vi "DrawOneLineXY.vi"() -> ()   [LabVIEW 2019]
uses:
  <vilib>/Utility/miscctls.llb/LVBoundsTypeDef.ctl
panel:
  out "Plot Area:Size":T1
  in  "stop":bool
  out "XY Graph":cluster{"X":dbl, "Y":dbl}[](graph)
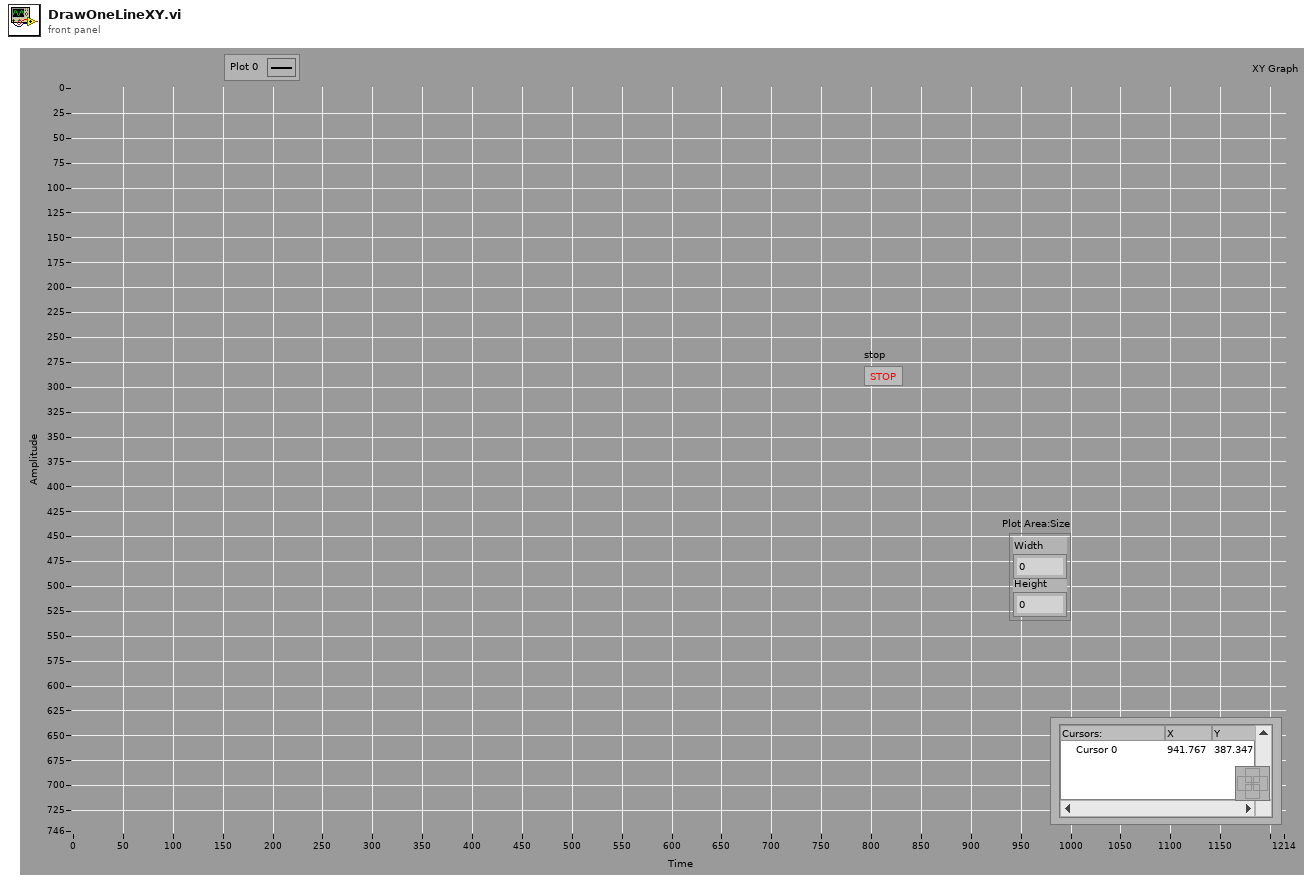
[diagram p1: front panel]
types:
  T1 = typedef "LVBoundsTypeDef.ctl" = cluster{"Width":u32, "Height":u32}
  T2 = typedef "LVPoint32TypeDef.ctl" = cluster{"Horizontal":i32, "Vertical":i32}
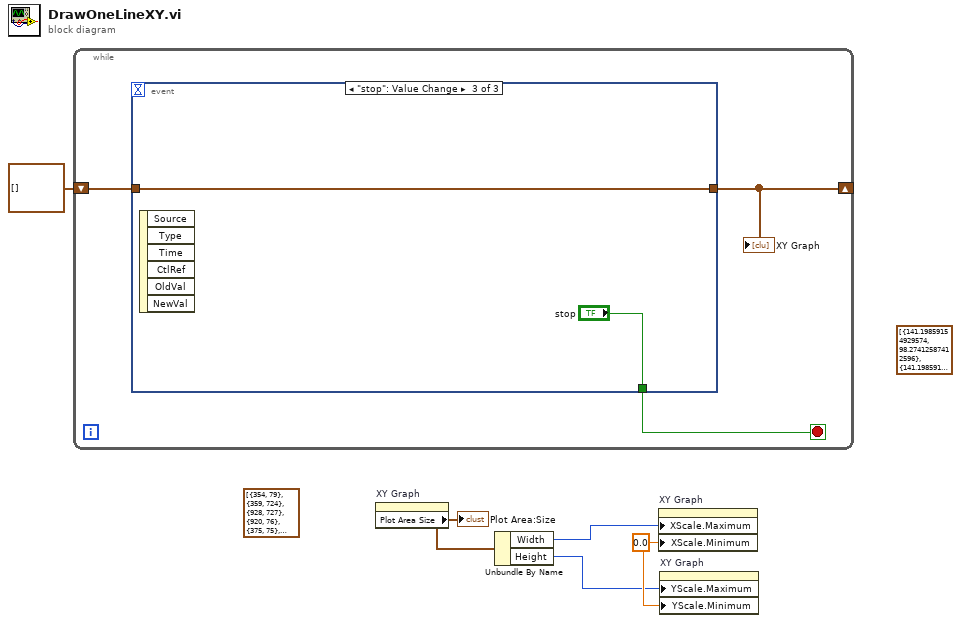
[diagram p0: block diagram]
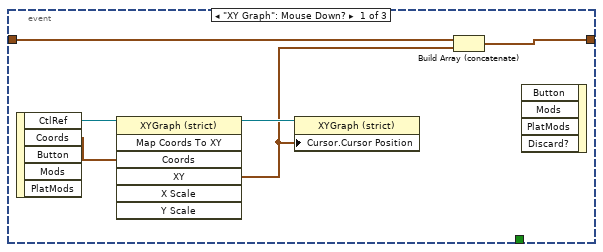
[diagram p2: hidden frame]
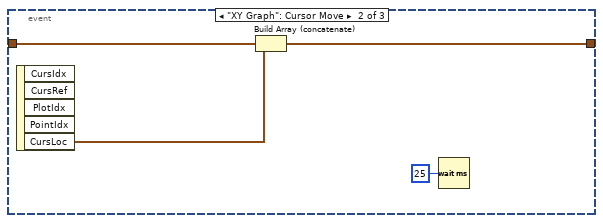
[diagram p3: hidden frame]
diagram:
  w4 = 0.0 ("X Scale.Range:Minimum")
  (unwired) cluster{"X":dbl, "Y":dbl}[] [{"X"=141.19859154929574, "Y"=98.27412587412596}, {"X"=141.19859154929574, "Y"=97.27132867132866}, {"X"=141.19859154929574, "Y"=98.27412587412596}, {"X"=142.19999999999996, "Y"=98.27412587412596}, {"X"=142.19999999999996, "Y"=99.27692307692314}, {"X"=142.19999999999996, "Y"=100.27972027972032}, {"X"=142.19999999999996, "Y"=101.2825174825175}, {"X"=141.19859154929574, "Y"=102.28531468531469}, {"X"=140.1971830985915, "Y"=103.28811188811187}, {"X"=140.1971830985915, "Y"=104.29090909090917}, {"X"=139.19577464788728, "Y"=104.29090909090917}, {"X"=139.19577464788728, "Y"=105.29370629370635}, {"X"=139.19577464788728, "Y"=106.29650349650353}, {"X"=138.19436619718306, "Y"=107.29930069930072}, {"X"=138.19436619718306, "Y"=110.30769230769238}, {"X"=138.19436619718306, "Y"=112.31328671328674}, {"X"=138.19436619718306, "Y"=115.3216783216784}, {"X"=137.19295774647884, "Y"=118.33006993006995}, {"X"=136.1915492957746, "Y"=122.3412587412588}, {"X"=135.19014084507037, "Y"=126.35244755244753}, {"X"=134.18873239436616, "Y"=129.3608391608392}, {"X"=134.18873239436616, "Y"=132.36923076923085}, {"X"=133.18732394366194, "Y"=135.3776223776224}, {"X"=132.18591549295772, "Y"=138.38601398601406}, {"X"=130.18309859154925, "Y"=143.39999999999998}, {"X"=129.18169014084503, "Y"=146.40839160839164}, {"X"=128.18028169014082, "Y"=148.413986013986}, {"X"=126.17746478873235, "Y"=151.42237762237767}, {"X"=126.17746478873235, "Y"=153.42797202797203}, {"X"=125.17605633802813, "Y"=155.4335664335665}, {"X"=124.17464788732391, "Y"=157.43916083916088}, {"X"=122.17183098591545, "Y"=161.45034965034972}, {"X"=121.17042253521123, "Y"=162.4531468531469}, {"X"=121.17042253521123, "Y"=164.45874125874127}, {"X"=120.16901408450701, "Y"=167.46713286713293}, {"X"=119.16760563380276, "Y"=169.4727272727273}, {"X"=118.16619718309855, "Y"=172.48111888111896}, {"X"=117.16478873239433, "Y"=175.4895104895105}, {"X"=116.16338028169011, "Y"=178.49790209790217}, {"X"=115.16197183098589, "Y"=180.50349650349654}, {"X"=113.15915492957743, "Y"=182.5090909090909}, {"X"=112.15774647887321, "Y"=185.51748251748256}, {"X"=111.15633802816899, "Y"=187.52307692307693}, {"X"=109.15352112676052, "Y"=190.5314685314686}, {"X"=108.1521126760563, "Y"=193.53986013986014}, {"X"=107.15070422535209, "Y"=195.54545454545462}, {"X"=106.14929577464784, "Y"=196.5482517482518}, {"X"=106.14929577464784, "Y"=198.55384615384617}, {"X"=105.14788732394362, "Y"=199.55664335664335}, {"X"=104.1464788732394, "Y"=201.56223776223783}, {"X"=103.14507042253518, "Y"=204.57062937062938}, {"X"=101.14225352112672, "Y"=205.57342657342662}, {"X"=100.1408450704225, "Y"=208.58181818181822}, {"X"=98.13802816901406, "Y"=209.5846153846154}, {"X"=97.13661971830982, "Y"=210.5874125874126}, {"X"=96.1352112676056, "Y"=211.59020979020983}, {"X"=95.13380281690138, "Y"=212.593006993007}, {"X"=94.13239436619716, "Y"=214.59860139860143}, {"X"=93.13098591549291, "Y"=216.60419580419585}, {"X"=91.12816901408448, "Y"=217.60699300699304}, {"X"=91.12816901408448, "Y"=219.61258741258746}, {"X"=90.12676056338026, "Y"=221.61818181818182}, {"X"=89.12535211267601, "Y"=221.61818181818182}, {"X"=88.1239436619718, "Y"=222.62097902097906}, {"X"=88.1239436619718, "Y"=223.62377622377625}, {"X"=87.12253521126758, "Y"=224.62657342657343}, {"X"=87.12253521126758, "Y"=225.62937062937067}, {"X"=86.12112676056336, "Y"=226.63216783216785}, {"X"=86.12112676056336, "Y"=227.63496503496503}, {"X"=85.11971830985914, "Y"=228.63776223776227}, {"X"=84.11830985915489, "Y"=228.63776223776227}, {"X"=85.11971830985914, "Y"=227.63496503496503}, {"X"=87.12253521126758, "Y"=224.62657342657343}, {"X"=90.12676056338026, "Y"=220.61538461538464}, {"X"=92.1295774647887, "Y"=218.60979020979022}, {"X"=94.13239436619716, "Y"=215.6013986013986}, {"X"=95.13380281690138, "Y"=214.59860139860143}, {"X"=96.1352112676056, "Y"=213.59580419580425}, {"X"=98.13802816901406, "Y"=212.593006993007}, {"X"=100.1408450704225, "Y"=211.59020979020983}, {"X"=101.14225352112672, "Y"=210.5874125874126}, {"X"=103.14507042253518, "Y"=208.58181818181822}, {"X"=106.14929577464784, "Y"=206.5762237762238}, {"X"=108.1521126760563, "Y"=205.57342657342662}, {"X"=109.15352112676052, "Y"=205.57342657342662}, {"X"=111.15633802816899, "Y"=204.57062937062938}, {"X"=113.15915492957743, "Y"=203.5678321678322}, {"X"=115.16197183098589, "Y"=202.565034965035}, {"X"=117.16478873239433, "Y"=202.565034965035}, {"X"=119.16760563380276, "Y"=201.56223776223783}, {"X"=120.16901408450701, "Y"=201.56223776223783}, {"X"=123.17323943661967, "Y"=200.55944055944053}, {"X"=125.17605633802813, "Y"=200.55944055944053}, {"X"=126.17746478873235, "Y"=200.55944055944053}, {"X"=127.17887323943657, "Y"=200.55944055944053}, {"X"=128.18028169014082, "Y"=200.55944055944053}, {"X"=129.18169014084503, "Y"=199.55664335664335}, {"X"=131.18450704225347, "Y"=200.55944055944053}, {"X"=132.18591549295772, "Y"=200.55944055944053}, {"X"=134.18873239436616, "Y"=201.56223776223783}, {"X"=136.1915492957746, "Y"=202.565034965035}, {"X"=138.19436619718306, "Y"=203.5678321678322}, {"X"=140.1971830985915, "Y"=204.57062937062938}, {"X"=141.19859154929574, "Y"=204.57062937062938}, {"X"=142.19999999999996, "Y"=204.57062937062938}, {"X"=143.20140845070418, "Y"=205.57342657342662}, {"X"=145.20422535211264, "Y"=205.57342657342662}, {"X"=145.20422535211264, "Y"=206.5762237762238}, {"X"=146.20563380281686, "Y"=207.57902097902098}, {"X"=147.20704225352108, "Y"=207.57902097902098}, {"X"=148.2084507042253, "Y"=207.57902097902098}, {"X"=148.2084507042253, "Y"=208.58181818181822}, {"X"=149.20985915492952, "Y"=208.58181818181822}, {"X"=150.21126760563376, "Y"=209.5846153846154}, {"X"=151.21267605633798, "Y"=209.5846153846154}, {"X"=152.2140845070422, "Y"=209.5846153846154}, {"X"=151.21267605633798, "Y"=209.5846153846154}, {"X"=150.21126760563376, "Y"=209.5846153846154}, {"X"=191.26901408450698, "Y"=181.50629370629372}, {"X"=190.26760563380276, "Y"=182.5090909090909}, {"X"=190.26760563380276, "Y"=183.51188811188808}, {"X"=190.26760563380276, "Y"=184.51468531468538}, {"X"=189.26619718309854, "Y"=186.52027972027975}, {"X"=189.26619718309854, "Y"=188.5258741258741}, {"X"=189.26619718309854, "Y"=189.5286713286714}, {"X"=188.26478873239432, "Y"=191.53426573426577}, {"X"=188.26478873239432, "Y"=193.53986013986014}, {"X"=187.2633802816901, "Y"=196.5482517482518}, {"X"=187.2633802816901, "Y"=198.55384615384617}, {"X"=186.26197183098589, "Y"=198.55384615384617}, {"X"=186.26197183098589, "Y"=200.55944055944053}, {"X"=185.2605633802816, "Y"=201.56223776223783}, {"X"=185.2605633802816, "Y"=203.5678321678322}, {"X"=184.2591549295774, "Y"=204.57062937062938}, {"X"=184.2591549295774, "Y"=205.57342657342662}, {"X"=184.2591549295774, "Y"=207.57902097902098}, {"X"=183.25774647887317, "Y"=208.58181818181822}, {"X"=183.25774647887317, "Y"=210.5874125874126}, {"X"=183.25774647887317, "Y"=212.593006993007}, {"X"=182.25633802816895, "Y"=212.593006993007}, {"X"=182.25633802816895, "Y"=215.6013986013986}, {"X"=182.25633802816895, "Y"=216.60419580419585}, {"X"=182.25633802816895, "Y"=217.60699300699304}, {"X"=182.25633802816895, "Y"=218.60979020979022}, {"X"=181.25492957746474, "Y"=218.60979020979022}, {"X"=181.25492957746474, "Y"=219.61258741258746}, {"X"=181.25492957746474, "Y"=220.61538461538464}, {"X"=182.25633802816895, "Y"=221.61818181818182}, {"X"=183.25774647887317, "Y"=221.61818181818182}, {"X"=184.2591549295774, "Y"=221.61818181818182}, {"X"=185.2605633802816, "Y"=221.61818181818182}, {"X"=186.26197183098589, "Y"=221.61818181818182}, {"X"=187.2633802816901, "Y"=221.61818181818182}, {"X"=188.26478873239432, "Y"=220.61538461538464}, {"X"=190.26760563380276, "Y"=220.61538461538464}, {"X"=192.2704225352112, "Y"=219.61258741258746}, {"X"=193.27183098591541, "Y"=218.60979020979022}, {"X"=195.2746478873239, "Y"=218.60979020979022}, {"X"=199.28028169014078, "Y"=217.60699300699304}, {"X"=201.28309859154922, "Y"=217.60699300699304}, {"X"=203.2859154929577, "Y"=216.60419580419585}, {"X"=205.28873239436615, "Y"=216.60419580419585}, {"X"=208.2929577464788, "Y"=215.6013986013986}, {"X"=210.29577464788724, "Y"=215.6013986013986}, {"X"=211.29718309859152, "Y"=215.6013986013986}, {"X"=214.30140845070417, "Y"=214.59860139860143}, {"X"=215.3028169014084, "Y"=214.59860139860143}, {"X"=218.30704225352105, "Y"=213.59580419580425}, {"X"=220.30985915492954, "Y"=213.59580419580425}, {"X"=221.31126760563376, "Y"=212.593006993007}, {"X"=224.31549295774641, "Y"=212.593006993007}, {"X"=226.31830985915485, "Y"=211.59020979020983}, {"X"=227.31971830985907, "Y"=211.59020979020983}, {"X"=228.32112676056335, "Y"=211.59020979020983}, {"X"=229.32253521126756, "Y"=210.5874125874126}, {"X"=230.32394366197178, "Y"=210.5874125874126}, {"X"=231.325352112676, "Y"=210.5874125874126}, {"X"=232.32676056338022, "Y"=210.5874125874126}, {"X"=232.32676056338022, "Y"=209.5846153846154}, {"X"=233.32816901408444, "Y"=209.5846153846154}, {"X"=234.32957746478866, "Y"=209.5846153846154}, {"X"=235.33098591549287, "Y"=208.58181818181822}, {"X"=236.3323943661971, "Y"=208.58181818181822}, {"X"=237.33380281690137, "Y"=208.58181818181822}, {"X"=236.3323943661971, "Y"=208.58181818181822}, {"X"=237.33380281690137, "Y"=208.58181818181822}, {"X"=236.3323943661971, "Y"=208.58181818181822}, {"X"=235.33098591549287, "Y"=208.58181818181822}, {"X"=234.32957746478866, "Y"=208.58181818181822}, {"X"=233.32816901408444, "Y"=208.58181818181822}, {"X"=232.32676056338022, "Y"=208.58181818181822}, {"X"=231.325352112676, "Y"=208.58181818181822}, {"X"=230.32394366197178, "Y"=208.58181818181822}, {"X"=229.32253521126756, "Y"=208.58181818181822}, {"X"=229.32253521126756, "Y"=209.5846153846154}, {"X"=228.32112676056335, "Y"=209.5846153846154}, {"X"=227.31971830985907, "Y"=209.5846153846154}, {"X"=225.31690140845063, "Y"=210.5874125874126}, {"X"=222.31267605633798, "Y"=210.5874125874126}, {"X"=220.30985915492954, "Y"=211.59020979020983}, {"X"=217.30563380281683, "Y"=212.593006993007}, {"X"=213.29999999999995, "Y"=212.593006993007}, {"X"=210.29577464788724, "Y"=213.59580419580425}, {"X"=208.2929577464788, "Y"=213.59580419580425}, {"X"=205.28873239436615, "Y"=214.59860139860143}, {"X"=201.28309859154922, "Y"=214.59860139860143}, {"X"=196.27605633802813, "Y"=215.6013986013986}, {"X"=194.2732394366197, "Y"=216.60419580419585}, {"X"=192.2704225352112, "Y"=216.60419580419585}, {"X"=191.26901408450698, "Y"=216.60419580419585}, {"X"=190.26760563380276, "Y"=216.60419580419585}, {"X"=189.26619718309854, "Y"=216.60419580419585}, {"X"=189.26619718309854, "Y"=217.60699300699304}, {"X"=188.26478873239432, "Y"=217.60699300699304}, {"X"=187.2633802816901, "Y"=217.60699300699304}, {"X"=186.26197183098589, "Y"=217.60699300699304}, {"X"=186.26197183098589, "Y"=216.60419580419585}, {"X"=185.2605633802816, "Y"=216.60419580419585}, {"X"=185.2605633802816, "Y"=215.6013986013986}, {"X"=185.2605633802816, "Y"=214.59860139860143}, {"X"=185.2605633802816, "Y"=213.59580419580425}, {"X"=184.2591549295774, "Y"=213.59580419580425}, {"X"=184.2591549295774, "Y"=212.593006993007}, {"X"=184.2591549295774, "Y"=211.59020979020983}, {"X"=183.25774647887317, "Y"=211.59020979020983}, {"X"=183.25774647887317, "Y"=210.5874125874126}, {"X"=183.25774647887317, "Y"=209.5846153846154}, {"X"=184.2591549295774, "Y"=208.58181818181822}, {"X"=184.2591549295774, "Y"=207.57902097902098}, {"X"=184.2591549295774, "Y"=206.5762237762238}, {"X"=184.2591549295774, "Y"=205.57342657342662}, {"X"=185.2605633802816, "Y"=203.5678321678322}, {"X"=186.26197183098589, "Y"=201.56223776223783}, {"X"=187.2633802816901, "Y"=198.55384615384617}, {"X"=187.2633802816901, "Y"=195.54545454545462}, {"X"=188.26478873239432, "Y"=193.53986013986014}, {"X"=188.26478873239432, "Y"=192.53706293706296}, {"X"=189.26619718309854, "Y"=190.5314685314686}, {"X"=189.26619718309854, "Y"=188.5258741258741}, {"X"=189.26619718309854, "Y"=186.52027972027975}, {"X"=189.26619718309854, "Y"=184.51468531468538}, {"X"=189.26619718309854, "Y"=183.51188811188808}, {"X"=189.26619718309854, "Y"=182.5090909090909}, {"X"=189.26619718309854, "Y"=181.50629370629372}, {"X"=189.26619718309854, "Y"=180.50349650349654}, {"X"=189.26619718309854, "Y"=179.50069930069935}, {"X"=189.26619718309854, "Y"=178.49790209790217}, {"X"=190.26760563380276, "Y"=178.49790209790217}, {"X"=190.26760563380276, "Y"=177.49510489510487}, {"X"=190.26760563380276, "Y"=176.4923076923077}, {"X"=191.26901408450698, "Y"=176.4923076923077}, {"X"=191.26901408450698, "Y"=177.49510489510487}, {"X"=192.2704225352112, "Y"=177.49510489510487}, {"X"=193.27183098591541, "Y"=177.49510489510487}, {"X"=194.2732394366197, "Y"=177.49510489510487}, {"X"=196.27605633802813, "Y"=176.4923076923077}, {"X"=200.281690140845, "Y"=175.4895104895105}, {"X"=205.28873239436615, "Y"=174.48671328671333}, {"X"=210.29577464788724, "Y"=173.48391608391614}, {"X"=216.3042253521126, "Y"=171.47832167832166}, {"X"=220.30985915492954, "Y"=169.4727272727273}, {"X"=223.3140845070422, "Y"=168.46993006993011}, {"X"=227.31971830985907, "Y"=167.46713286713293}, {"X"=230.32394366197178, "Y"=166.46433566433564}, {"X"=233.32816901408444, "Y"=165.46153846153845}, {"X"=236.3323943661971, "Y"=164.45874125874127}, {"X"=239.3366197183098, "Y"=163.4559440559441}, {"X"=241.33943661971824, "Y"=163.4559440559441}, {"X"=242.34084507042246, "Y"=163.4559440559441}, {"X"=244.3436619718309, "Y"=162.4531468531469}, {"X"=247.3478873239436, "Y"=162.4531468531469}, {"X"=248.34929577464783, "Y"=161.45034965034972}, {"X"=249.35070422535205, "Y"=161.45034965034972}, {"X"=250.35211267605627, "Y"=161.45034965034972}, {"X"=251.35352112676048, "Y"=161.45034965034972}, {"X"=252.3549295774647, "Y"=161.45034965034972}, {"X"=253.35633802816892, "Y"=160.44755244755243}, {"X"=254.3577464788732, "Y"=160.44755244755243}, {"X"=255.35915492957741, "Y"=160.44755244755243}, {"X"=256.36056338028163, "Y"=160.44755244755243}, {"X"=257.36197183098585, "Y"=160.44755244755243}, {"X"=258.36338028169007, "Y"=160.44755244755243}, {"X"=257.36197183098585, "Y"=160.44755244755243}, {"X"=257.36197183098585, "Y"=161.45034965034972}, {"X"=256.36056338028163, "Y"=161.45034965034972}, {"X"=251.35352112676048, "Y"=161.45034965034972}, {"X"=246.3464788732394, "Y"=162.4531468531469}, {"X"=240.33802816901402, "Y"=162.4531468531469}, {"X"=234.32957746478866, "Y"=164.45874125874127}, {"X"=228.32112676056335, "Y"=165.46153846153845}, {"X"=223.3140845070422, "Y"=167.46713286713293}, {"X"=219.30845070422527, "Y"=169.4727272727273}, {"X"=216.3042253521126, "Y"=170.47552447552448}, {"X"=213.29999999999995, "Y"=171.47832167832166}, {"X"=210.29577464788724, "Y"=172.48111888111896}, {"X"=208.2929577464788, "Y"=172.48111888111896}, {"X"=206.29014084507037, "Y"=173.48391608391614}, {"X"=204.28732394366193, "Y"=174.48671328671333}, {"X"=202.28450704225344, "Y"=174.48671328671333}, {"X"=200.281690140845, "Y"=175.4895104895105}, {"X"=199.28028169014078, "Y"=175.4895104895105}, {"X"=198.27887323943656, "Y"=176.4923076923077}, {"X"=196.27605633802813, "Y"=176.4923076923077}, {"X"=193.27183098591541, "Y"=177.49510489510487}, {"X"=192.2704225352112, "Y"=178.49790209790217}, {"X"=191.26901408450698, "Y"=181.50629370629372}, {"X"=190.26760563380276, "Y"=183.51188811188808}, {"X"=190.26760563380276, "Y"=186.52027972027975}, {"X"=189.26619718309854, "Y"=189.5286713286714}, {"X"=188.26478873239432, "Y"=190.5314685314686}, {"X"=188.26478873239432, "Y"=191.53426573426577}, {"X"=187.2633802816901, "Y"=193.53986013986014}, {"X"=186.26197183098589, "Y"=194.54265734265732}, {"X"=186.26197183098589, "Y"=195.54545454545462}, {"X"=186.26197183098589, "Y"=196.5482517482518}, {"X"=185.2605633802816, "Y"=196.5482517482518}, {"X"=185.2605633802816, "Y"=197.55104895104898}, {"X"=184.2591549295774, "Y"=197.55104895104898}, {"X"=184.2591549295774, "Y"=198.55384615384617}, {"X"=185.2605633802816, "Y"=198.55384615384617}, {"X"=186.26197183098589, "Y"=198.55384615384617}, {"X"=187.2633802816901, "Y"=198.55384615384617}, {"X"=188.26478873239432, "Y"=198.55384615384617}, {"X"=189.26619718309854, "Y"=198.55384615384617}, {"X"=190.26760563380276, "Y"=198.55384615384617}, {"X"=191.26901408450698, "Y"=197.55104895104898}, {"X"=192.2704225352112, "Y"=197.55104895104898}, {"X"=193.27183098591541, "Y"=197.55104895104898}, {"X"=194.2732394366197, "Y"=197.55104895104898}, {"X"=197.27746478873235, "Y"=197.55104895104898}, {"X"=198.27887323943656, "Y"=197.55104895104898}, {"X"=200.281690140845, "Y"=197.55104895104898}, {"X"=203.2859154929577, "Y"=196.5482517482518}, {"X"=205.28873239436615, "Y"=196.5482517482518}, {"X"=207.2915492957746, "Y"=196.5482517482518}, {"X"=210.29577464788724, "Y"=196.5482517482518}, {"X"=213.29999999999995, "Y"=195.54545454545462}, {"X"=217.30563380281683, "Y"=195.54545454545462}, {"X"=221.31126760563376, "Y"=194.54265734265732}, {"X"=223.3140845070422, "Y"=194.54265734265732}, {"X"=226.31830985915485, "Y"=193.53986013986014}, {"X"=228.32112676056335, "Y"=192.53706293706296}, {"X"=230.32394366197178, "Y"=192.53706293706296}, {"X"=233.32816901408444, "Y"=191.53426573426577}, {"X"=234.32957746478866, "Y"=191.53426573426577}, {"X"=237.33380281690137, "Y"=190.5314685314686}, {"X"=239.3366197183098, "Y"=190.5314685314686}, {"X"=240.33802816901402, "Y"=189.5286713286714}, {"X"=241.33943661971824, "Y"=189.5286713286714}, {"X"=242.34084507042246, "Y"=188.5258741258741}, {"X"=243.34225352112668, "Y"=188.5258741258741}, {"X"=244.3436619718309, "Y"=188.5258741258741}, {"X"=246.3464788732394, "Y"=187.52307692307693}, {"X"=248.34929577464783, "Y"=187.52307692307693}, {"X"=249.35070422535205, "Y"=187.52307692307693}, {"X"=250.35211267605627, "Y"=187.52307692307693}, {"X"=250.35211267605627, "Y"=186.52027972027975}, {"X"=251.35352112676048, "Y"=186.52027972027975}, {"X"=252.3549295774647, "Y"=186.52027972027975}, {"X"=251.35352112676048, "Y"=186.52027972027975}, {"X"=268.3774647887323, "Y"=177.49510489510487}, {"X"=269.37887323943653, "Y"=177.49510489510487}, {"X"=270.38028169014075, "Y"=177.49510489510487}, {"X"=271.381690140845, "Y"=177.49510489510487}, {"X"=272.38309859154924, "Y"=177.49510489510487}, {"X"=273.38450704225346, "Y"=177.49510489510487}, {"X"=274.3859154929577, "Y"=177.49510489510487}, {"X"=275.3873239436619, "Y"=177.49510489510487}, {"X"=277.39014084507033, "Y"=176.4923076923077}, {"X"=278.39154929577455, "Y"=176.4923076923077}, {"X"=281.39577464788727, "Y"=176.4923076923077}, {"X"=283.3985915492957, "Y"=176.4923076923077}, {"X"=286.40281690140836, "Y"=175.4895104895105}, {"X"=288.40563380281685, "Y"=175.4895104895105}, {"X"=289.40704225352107, "Y"=174.48671328671333}, {"X"=291.4098591549295, "Y"=174.48671328671333}, {"X"=293.41267605633794, "Y"=174.48671328671333}, {"X"=296.4169014084506, "Y"=174.48671328671333}, {"X"=299.4211267605633, "Y"=174.48671328671333}, {"X"=301.42394366197175, "Y"=173.48391608391614}, {"X"=304.4281690140844, "Y"=173.48391608391614}, {"X"=308.43380281690133, "Y"=173.48391608391614}, {"X"=312.4394366197182, "Y"=173.48391608391614}, {"X"=315.4436619718309, "Y"=173.48391608391614}, {"X"=317.44647887323936, "Y"=172.48111888111896}, {"X"=320.450704225352, "Y"=172.48111888111896}, {"X"=321.45211267605623, "Y"=172.48111888111896}, {"X"=322.4535211267605, "Y"=172.48111888111896}, {"X"=323.4549295774647, "Y"=172.48111888111896}, {"X"=324.45633802816894, "Y"=172.48111888111896}, {"X"=325.45774647887316, "Y"=172.48111888111896}, {"X"=327.4605633802816, "Y"=172.48111888111896}, {"X"=328.4619718309858, "Y"=172.48111888111896}, {"X"=329.46338028169004, "Y"=172.48111888111896}, {"X"=330.46478873239425, "Y"=172.48111888111896}, {"X"=330.46478873239425, "Y"=171.47832167832166}, {"X"=331.46619718309853, "Y"=171.47832167832166}, {"X"=332.46760563380275, "Y"=171.47832167832166}, {"X"=329.46338028169004, "Y"=171.47832167832166}, {"X"=326.4591549295774, "Y"=172.48111888111896}, {"X"=323.4549295774647, "Y"=172.48111888111896}, {"X"=320.450704225352, "Y"=172.48111888111896}, {"X"=317.44647887323936, "Y"=173.48391608391614}, {"X"=314.4422535211267, "Y"=173.48391608391614}, {"X"=310.43661971830977, "Y"=173.48391608391614}, {"X"=305.4295774647887, "Y"=173.48391608391614}, {"X"=303.4267605633802, "Y"=173.48391608391614}, {"X"=301.42394366197175, "Y"=173.48391608391614}, {"X"=298.4197183098591, "Y"=173.48391608391614}, {"X"=297.4183098591549, "Y"=173.48391608391614}, {"X"=295.4154929577464, "Y"=172.48111888111896}, {"X"=293.41267605633794, "Y"=172.48111888111896}, {"X"=292.4112676056337, "Y"=173.48391608391614}, {"X"=291.4098591549295, "Y"=173.48391608391614}, {"X"=290.4084507042253, "Y"=173.48391608391614}, {"X"=289.40704225352107, "Y"=173.48391608391614}, {"X"=288.40563380281685, "Y"=173.48391608391614}, {"X"=287.4042253521126, "Y"=173.48391608391614}, {"X"=286.40281690140836, "Y"=173.48391608391614}, {"X"=285.40140845070414, "Y"=173.48391608391614}, {"X"=285.40140845070414, "Y"=174.48671328671333}, {"X"=284.3999999999999, "Y"=175.4895104895105}, {"X"=284.3999999999999, "Y"=176.4923076923077}, {"X"=283.3985915492957, "Y"=176.4923076923077}, {"X"=283.3985915492957, "Y"=177.49510489510487}, {"X"=282.3971830985915, "Y"=179.50069930069935}, {"X"=281.39577464788727, "Y"=180.50349650349654}, {"X"=280.39436619718305, "Y"=181.50629370629372}, {"X"=279.39295774647877, "Y"=183.51188811188808}, {"X"=278.39154929577455, "Y"=185.51748251748256}, {"X"=277.39014084507033, "Y"=187.52307692307693}, {"X"=275.3873239436619, "Y"=190.5314685314686}, {"X"=274.3859154929577, "Y"=192.53706293706296}, {"X"=273.38450704225346, "Y"=193.53986013986014}, {"X"=271.381690140845, "Y"=195.54545454545462}, {"X"=270.38028169014075, "Y"=197.55104895104898}, {"X"=268.3774647887323, "Y"=199.55664335664335}, {"X"=267.3760563380281, "Y"=200.55944055944053}, {"X"=266.3746478873239, "Y"=201.56223776223783}, {"X"=265.37323943661966, "Y"=203.5678321678322}, {"X"=264.37183098591544, "Y"=204.57062937062938}, {"X"=264.37183098591544, "Y"=205.57342657342662}, {"X"=263.3704225352112, "Y"=205.57342657342662}, {"X"=263.3704225352112, "Y"=206.5762237762238}, {"X"=263.3704225352112, "Y"=207.57902097902098}, {"X"=262.36901408450694, "Y"=207.57902097902098}, {"X"=262.36901408450694, "Y"=208.58181818181822}, {"X"=262.36901408450694, "Y"=209.5846153846154}, {"X"=261.3676056338027, "Y"=209.5846153846154}, {"X"=260.3661971830985, "Y"=208.58181818181822}, {"X"=259.3647887323943, "Y"=208.58181818181822}, {"X"=259.3647887323943, "Y"=207.57902097902098}, {"X"=372.5239436619717, "Y"=157.43916083916088}, {"X"=371.5225352112675, "Y"=157.43916083916088}, {"X"=371.5225352112675, "Y"=156.4363636363637}, {"X"=370.5211267605633, "Y"=156.4363636363637}, {"X"=369.51971830985906, "Y"=156.4363636363637}, {"X"=368.51830985915484, "Y"=156.4363636363637}, {"X"=367.5169014084506, "Y"=156.4363636363637}, {"X"=366.5154929577464, "Y"=156.4363636363637}, {"X"=365.5140845070422, "Y"=156.4363636363637}, {"X"=364.5126760563379, "Y"=156.4363636363637}, {"X"=364.5126760563379, "Y"=157.43916083916088}, {"X"=363.5112676056337, "Y"=157.43916083916088}, {"X"=362.5098591549295, "Y"=157.43916083916088}, {"X"=361.50845070422525, "Y"=157.43916083916088}, {"X"=360.50704225352104, "Y"=157.43916083916088}, {"X"=359.5056338028168, "Y"=157.43916083916088}, {"X"=358.5042253521126, "Y"=157.43916083916088}, {"X"=357.5028169014084, "Y"=157.43916083916088}, {"X"=357.5028169014084, "Y"=158.44195804195806}, {"X"=356.50140845070416, "Y"=158.44195804195806}, {"X"=355.4999999999999, "Y"=158.44195804195806}, {"X"=354.49859154929567, "Y"=158.44195804195806}, {"X"=353.49718309859145, "Y"=159.44475524475524}, {"X"=352.49577464788723, "Y"=159.44475524475524}, {"X"=351.494366197183, "Y"=159.44475524475524}, {"X"=350.4929577464788, "Y"=160.44755244755243}, {"X"=349.4915492957746, "Y"=160.44755244755243}, {"X"=348.49014084507036, "Y"=161.45034965034972}, {"X"=348.49014084507036, "Y"=162.4531468531469}, {"X"=347.4887323943661, "Y"=163.4559440559441}, {"X"=347.4887323943661, "Y"=164.45874125874127}, {"X"=346.48732394366186, "Y"=164.45874125874127}, {"X"=346.48732394366186, "Y"=165.46153846153845}, {"X"=346.48732394366186, "Y"=168.46993006993011}, {"X"=346.48732394366186, "Y"=169.4727272727273}, {"X"=346.48732394366186, "Y"=170.47552447552448}, {"X"=347.4887323943661, "Y"=171.47832167832166}, {"X"=347.4887323943661, "Y"=172.48111888111896}, {"X"=347.4887323943661, "Y"=173.48391608391614}, {"X"=348.49014084507036, "Y"=173.48391608391614}, {"X"=348.49014084507036, "Y"=175.4895104895105}, {"X"=349.4915492957746, "Y"=176.4923076923077}, {"X"=350.4929577464788, "Y"=177.49510489510487}, {"X"=351.494366197183, "Y"=178.49790209790217}, {"X"=352.49577464788723, "Y"=178.49790209790217}, {"X"=352.49577464788723, "Y"=179.50069930069935}, {"X"=354.49859154929567, "Y"=180.50349650349654}, {"X"=355.4999999999999, "Y"=181.50629370629372}, {"X"=357.5028169014084, "Y"=182.5090909090909}, {"X"=358.5042253521126, "Y"=182.5090909090909}, {"X"=360.50704225352104, "Y"=183.51188811188808}, {"X"=361.50845070422525, "Y"=184.51468531468538}, {"X"=363.5112676056337, "Y"=185.51748251748256}, {"X"=365.5140845070422, "Y"=186.52027972027975}, {"X"=365.5140845070422, "Y"=188.5258741258741}, {"X"=366.5154929577464, "Y"=189.5286713286714}, {"X"=367.5169014084506, "Y"=189.5286713286714}, {"X"=367.5169014084506, "Y"=190.5314685314686}, {"X"=368.51830985915484, "Y"=191.53426573426577}, {"X"=368.51830985915484, "Y"=192.53706293706296}, {"X"=368.51830985915484, "Y"=193.53986013986014}, {"X"=368.51830985915484, "Y"=195.54545454545462}, {"X"=368.51830985915484, "Y"=196.5482517482518}, {"X"=368.51830985915484, "Y"=197.55104895104898}, {"X"=368.51830985915484, "Y"=198.55384615384617}, {"X"=367.5169014084506, "Y"=199.55664335664335}, {"X"=367.5169014084506, "Y"=200.55944055944053}, {"X"=367.5169014084506, "Y"=201.56223776223783}, {"X"=367.5169014084506, "Y"=202.565034965035}, {"X"=366.5154929577464, "Y"=202.565034965035}, {"X"=366.5154929577464, "Y"=203.5678321678322}, {"X"=365.5140845070422, "Y"=204.57062937062938}, {"X"=363.5112676056337, "Y"=204.57062937062938}, {"X"=362.5098591549295, "Y"=205.57342657342662}, {"X"=359.5056338028168, "Y"=205.57342657342662}, {"X"=357.5028169014084, "Y"=205.57342657342662}, {"X"=355.4999999999999, "Y"=205.57342657342662}, {"X"=353.49718309859145, "Y"=205.57342657342662}, {"X"=350.4929577464788, "Y"=205.57342657342662}, {"X"=348.49014084507036, "Y"=205.57342657342662}, {"X"=347.4887323943661, "Y"=205.57342657342662}, {"X"=344.4845070422534, "Y"=205.57342657342662}, {"X"=342.481690140845, "Y"=205.57342657342662}, {"X"=340.47887323943655, "Y"=205.57342657342662}, {"X"=338.47605633802806, "Y"=205.57342657342662}, {"X"=336.4732394366196, "Y"=205.57342657342662}, {"X"=334.4704225352112, "Y"=205.57342657342662}, {"X"=332.46760563380275, "Y"=205.57342657342662}, {"X"=329.46338028169004, "Y"=205.57342657342662}, {"X"=327.4605633802816, "Y"=205.57342657342662}, {"X"=325.45774647887316, "Y"=205.57342657342662}, {"X"=324.45633802816894, "Y"=205.57342657342662}, {"X"=322.4535211267605, "Y"=205.57342657342662}, {"X"=320.450704225352, "Y"=205.57342657342662}, {"X"=318.4478873239436, "Y"=205.57342657342662}, {"X"=317.44647887323936, "Y"=205.57342657342662}, {"X"=317.44647887323936, "Y"=204.57062937062938}, {"X"=316.44507042253514, "Y"=204.57062937062938}, {"X"=315.4436619718309, "Y"=204.57062937062938}, {"X"=314.4422535211267, "Y"=204.57062937062938}, {"X"=313.4408450704224, "Y"=204.57062937062938}, {"X"=312.4394366197182, "Y"=204.57062937062938}, {"X"=312.4394366197182, "Y"=203.5678321678322}, {"X"=552.7774647887322, "Y"=139.38881118881125}, {"X"=552.7774647887322, "Y"=140.39160839160843}, {"X"=551.7760563380281, "Y"=140.39160839160843}, {"X"=550.7746478873238, "Y"=140.39160839160843}, {"X"=549.7732394366196, "Y"=140.39160839160843}, {"X"=548.7718309859154, "Y"=140.39160839160843}, {"X"=547.7704225352111, "Y"=139.38881118881125}, {"X"=546.7690140845069, "Y"=139.38881118881125}, {"X"=545.7676056338026, "Y"=139.38881118881125}, {"X"=544.7661971830985, "Y"=139.38881118881125}, {"X"=543.7647887323942, "Y"=139.38881118881125}, {"X"=542.76338028169, "Y"=139.38881118881125}, {"X"=541.7619718309858, "Y"=138.38601398601406}, {"X"=540.7605633802816, "Y"=138.38601398601406}, {"X"=539.7591549295773, "Y"=138.38601398601406}, {"X"=538.7577464788731, "Y"=138.38601398601406}, {"X"=535.7535211267605, "Y"=138.38601398601406}, {"X"=534.7521126760562, "Y"=138.38601398601406}, {"X"=532.7492957746477, "Y"=137.38321678321677}, {"X"=531.7478873239436, "Y"=137.38321678321677}, {"X"=529.745070422535, "Y"=137.38321678321677}, {"X"=527.7422535211266, "Y"=137.38321678321677}, {"X"=525.7394366197182, "Y"=137.38321678321677}, {"X"=524.738028169014, "Y"=136.38041958041958}, {"X"=522.7352112676055, "Y"=136.38041958041958}, {"X"=520.732394366197, "Y"=136.38041958041958}, {"X"=518.7295774647886, "Y"=136.38041958041958}, {"X"=516.7267605633801, "Y"=136.38041958041958}, {"X"=516.7267605633801, "Y"=137.38321678321677}, {"X"=513.7225352112674, "Y"=137.38321678321677}, {"X"=511.719718309859, "Y"=137.38321678321677}, {"X"=510.71830985915483, "Y"=137.38321678321677}, {"X"=507.7140845070421, "Y"=137.38321678321677}, {"X"=505.7112676056337, "Y"=137.38321678321677}, {"X"=503.70845070422524, "Y"=137.38321678321677}, {"X"=502.70704225352097, "Y"=137.38321678321677}, {"X"=500.70422535211253, "Y"=138.38601398601406}, {"X"=498.7014084507041, "Y"=138.38601398601406}, {"X"=496.69859154929566, "Y"=138.38601398601406}, {"X"=495.6971830985914, "Y"=138.38601398601406}, {"X"=493.69436619718294, "Y"=138.38601398601406}, {"X"=490.69014084507035, "Y"=138.38601398601406}, {"X"=489.68873239436607, "Y"=139.38881118881125}, {"X"=486.68450704225336, "Y"=139.38881118881125}, {"X"=485.6830985915492, "Y"=140.39160839160843}, {"X"=484.6816901408449, "Y"=140.39160839160843}, {"X"=481.6774647887323, "Y"=140.39160839160843}, {"X"=480.67605633802805, "Y"=140.39160839160843}, {"X"=479.6746478873238, "Y"=141.3944055944056}, {"X"=477.67183098591534, "Y"=141.3944055944056}, {"X"=474.66760563380274, "Y"=142.3972027972028}, {"X"=472.6647887323943, "Y"=142.3972027972028}, {"X"=471.66338028169, "Y"=142.3972027972028}, {"X"=469.6605633802816, "Y"=143.39999999999998}, {"X"=467.65774647887315, "Y"=143.39999999999998}, {"X"=466.6563380281689, "Y"=144.40279720279727}, {"X"=464.65352112676044, "Y"=144.40279720279727}, {"X"=463.6521126760563, "Y"=145.40559440559446}, {"X"=462.650704225352, "Y"=145.40559440559446}, {"X"=461.6492957746477, "Y"=145.40559440559446}, {"X"=460.64788732394356, "Y"=145.40559440559446}, {"X"=460.64788732394356, "Y"=146.40839160839164}, {"X"=459.6464788732393, "Y"=146.40839160839164}, {"X"=458.6450704225351, "Y"=146.40839160839164}, {"X"=457.64366197183085, "Y"=147.41118881118882}, {"X"=456.6422535211267, "Y"=147.41118881118882}, {"X"=455.6408450704224, "Y"=147.41118881118882}, {"X"=455.6408450704224, "Y"=148.413986013986}, {"X"=454.63943661971814, "Y"=148.413986013986}, {"X"=452.6366197183097, "Y"=149.4167832167833}, {"X"=452.6366197183097, "Y"=150.41958041958048}, {"X"=451.63521126760554, "Y"=150.41958041958048}, {"X"=450.63380281690127, "Y"=150.41958041958048}, {"X"=450.63380281690127, "Y"=151.42237762237767}, {"X"=449.6323943661971, "Y"=151.42237762237767}, {"X"=448.63098591549283, "Y"=151.42237762237767}, {"X"=449.6323943661971, "Y"=151.42237762237767}, {"X"=489.68873239436607, "Y"=142.3972027972028}, {"X"=488.6873239436618, "Y"=143.39999999999998}, {"X"=487.68591549295763, "Y"=143.39999999999998}, {"X"=487.68591549295763, "Y"=144.40279720279727}, {"X"=486.68450704225336, "Y"=144.40279720279727}, {"X"=485.6830985915492, "Y"=145.40559440559446}, {"X"=484.6816901408449, "Y"=146.40839160839164}, {"X"=483.68028169014076, "Y"=146.40839160839164}, {"X"=483.68028169014076, "Y"=147.41118881118882}, {"X"=482.6788732394365, "Y"=147.41118881118882}, {"X"=480.67605633802805, "Y"=148.413986013986}, {"X"=479.6746478873238, "Y"=149.4167832167833}, {"X"=477.67183098591534, "Y"=150.41958041958048}, {"X"=476.6704225352112, "Y"=151.42237762237767}, {"X"=475.6690140845069, "Y"=152.42517482517485}, {"X"=474.66760563380274, "Y"=152.42517482517485}, {"X"=473.66619718309846, "Y"=153.42797202797203}, {"X"=472.6647887323943, "Y"=154.43076923076922}, {"X"=471.66338028169, "Y"=155.4335664335665}, {"X"=470.66197183098575, "Y"=156.4363636363637}, {"X"=469.6605633802816, "Y"=156.4363636363637}, {"X"=467.65774647887315, "Y"=157.43916083916088}, {"X"=466.6563380281689, "Y"=158.44195804195806}, {"X"=465.6549295774647, "Y"=159.44475524475524}, {"X"=463.6521126760563, "Y"=160.44755244755243}, {"X"=461.6492957746477, "Y"=161.45034965034972}, {"X"=460.64788732394356, "Y"=162.4531468531469}, {"X"=459.6464788732393, "Y"=163.4559440559441}, {"X"=458.6450704225351, "Y"=164.45874125874127}, {"X"=457.64366197183085, "Y"=165.46153846153845}, {"X"=457.64366197183085, "Y"=166.46433566433564}, {"X"=456.6422535211267, "Y"=168.46993006993011}, {"X"=455.6408450704224, "Y"=170.47552447552448}, {"X"=454.63943661971814, "Y"=172.48111888111896}, {"X"=454.63943661971814, "Y"=174.48671328671333}, {"X"=453.638028169014, "Y"=175.4895104895105}, {"X"=453.638028169014, "Y"=176.4923076923077}, {"X"=452.6366197183097, "Y"=176.4923076923077}, {"X"=452.6366197183097, "Y"=177.49510489510487}, {"X"=451.63521126760554, "Y"=179.50069930069935}, {"X"=451.63521126760554, "Y"=180.50349650349654}, {"X"=450.63380281690127, "Y"=181.50629370629372}, {"X"=450.63380281690127, "Y"=182.5090909090909}, {"X"=449.6323943661971, "Y"=184.51468531468538}, {"X"=449.6323943661971, "Y"=185.51748251748256}, {"X"=449.6323943661971, "Y"=186.52027972027975}, {"X"=448.63098591549283, "Y"=187.52307692307693}, {"X"=448.63098591549283, "Y"=189.5286713286714}, {"X"=448.63098591549283, "Y"=190.5314685314686}, {"X"=448.63098591549283, "Y"=191.53426573426577}, {"X"=447.62957746478867, "Y"=191.53426573426577}, {"X"=447.62957746478867, "Y"=192.53706293706296}, {"X"=447.62957746478867, "Y"=193.53986013986014}, {"X"=447.62957746478867, "Y"=194.54265734265732}, {"X"=447.62957746478867, "Y"=195.54545454545462}, {"X"=447.62957746478867, "Y"=196.5482517482518}, {"X"=448.63098591549283, "Y"=197.55104895104898}, {"X"=448.63098591549283, "Y"=198.55384615384617}, {"X"=448.63098591549283, "Y"=199.55664335664335}, {"X"=448.63098591549283, "Y"=200.55944055944053}, {"X"=448.63098591549283, "Y"=201.56223776223783}, {"X"=448.63098591549283, "Y"=202.565034965035}, {"X"=449.6323943661971, "Y"=203.5678321678322}, {"X"=449.6323943661971, "Y"=204.57062937062938}, {"X"=449.6323943661971, "Y"=205.57342657342662}, {"X"=449.6323943661971, "Y"=206.5762237762238}, {"X"=450.63380281690127, "Y"=206.5762237762238}, {"X"=450.63380281690127, "Y"=207.57902097902098}, {"X"=451.63521126760554, "Y"=207.57902097902098}, {"X"=452.6366197183097, "Y"=207.57902097902098}, {"X"=453.638028169014, "Y"=208.58181818181822}, {"X"=454.63943661971814, "Y"=208.58181818181822}, {"X"=455.6408450704224, "Y"=208.58181818181822}, {"X"=456.6422535211267, "Y"=209.5846153846154}, {"X"=458.6450704225351, "Y"=209.5846153846154}, {"X"=460.64788732394356, "Y"=209.5846153846154}, {"X"=463.6521126760563, "Y"=209.5846153846154}, {"X"=465.6549295774647, "Y"=209.5846153846154}, {"X"=471.66338028169, "Y"=209.5846153846154}, {"X"=475.6690140845069, "Y"=209.5846153846154}, {"X"=479.6746478873238, "Y"=208.58181818181822}, {"X"=484.6816901408449, "Y"=207.57902097902098}, {"X"=487.68591549295763, "Y"=207.57902097902098}, {"X"=489.68873239436607, "Y"=206.5762237762238}, {"X"=494.6957746478872, "Y"=205.57342657342662}, {"X"=497.69999999999993, "Y"=205.57342657342662}, {"X"=501.7056338028168, "Y"=204.57062937062938}, {"X"=504.7098591549294, "Y"=203.5678321678322}, {"X"=508.7154929577464, "Y"=202.565034965035}, {"X"=511.719718309859, "Y"=201.56223776223783}, {"X"=513.7225352112674, "Y"=200.55944055944053}, {"X"=515.725352112676, "Y"=200.55944055944053}, {"X"=517.7281690140844, "Y"=199.55664335664335}, {"X"=519.7309859154929, "Y"=198.55384615384617}, {"X"=520.732394366197, "Y"=198.55384615384617}, {"X"=521.7338028169013, "Y"=198.55384615384617}, {"X"=522.7352112676055, "Y"=197.55104895104898}, {"X"=524.738028169014, "Y"=197.55104895104898}, {"X"=523.7366197183097, "Y"=197.55104895104898}, {"X"=522.7352112676055, "Y"=197.55104895104898}, {"X"=521.7338028169013, "Y"=196.5482517482518}, {"X"=520.732394366197, "Y"=196.5482517482518}, {"X"=448.63098591549283, "Y"=187.52307692307693}, {"X"=453.638028169014, "Y"=184.51468531468538}, {"X"=454.63943661971814, "Y"=184.51468531468538}, {"X"=455.6408450704224, "Y"=184.51468531468538}, {"X"=456.6422535211267, "Y"=184.51468531468538}, {"X"=457.64366197183085, "Y"=184.51468531468538}, {"X"=458.6450704225351, "Y"=184.51468531468538}, {"X"=460.64788732394356, "Y"=183.51188811188808}, {"X"=462.650704225352, "Y"=183.51188811188808}, {"X"=466.6563380281689, "Y"=182.5090909090909}, {"X"=469.6605633802816, "Y"=182.5090909090909}, {"X"=473.66619718309846, "Y"=181.50629370629372}, {"X"=475.6690140845069, "Y"=181.50629370629372}, {"X"=479.6746478873238, "Y"=180.50349650349654}, {"X"=482.6788732394365, "Y"=179.50069930069935}, {"X"=486.68450704225336, "Y"=178.49790209790217}, {"X"=489.68873239436607, "Y"=178.49790209790217}, {"X"=492.6929577464788, "Y"=177.49510489510487}, {"X"=494.6957746478872, "Y"=177.49510489510487}, {"X"=498.7014084507041, "Y"=176.4923076923077}, {"X"=500.70422535211253, "Y"=176.4923076923077}, {"X"=503.70845070422524, "Y"=175.4895104895105}, {"X"=505.7112676056337, "Y"=175.4895104895105}, {"X"=507.7140845070421, "Y"=174.48671328671333}, {"X"=509.71690140845055, "Y"=174.48671328671333}, {"X"=511.719718309859, "Y"=174.48671328671333}, {"X"=513.7225352112674, "Y"=173.48391608391614}, {"X"=515.725352112676, "Y"=173.48391608391614}, {"X"=516.7267605633801, "Y"=173.48391608391614}, {"X"=517.7281690140844, "Y"=173.48391608391614}, {"X"=518.7295774647886, "Y"=172.48111888111896}, {"X"=519.7309859154929, "Y"=172.48111888111896}, {"X"=520.732394366197, "Y"=172.48111888111896}, {"X"=521.7338028169013, "Y"=172.48111888111896}, {"X"=522.7352112676055, "Y"=171.47832167832166}, {"X"=523.7366197183097, "Y"=171.47832167832166}, {"X"=525.7394366197182, "Y"=171.47832167832166}, {"X"=524.738028169014, "Y"=171.47832167832166}, {"X"=523.7366197183097, "Y"=171.47832167832166}, {"X"=522.7352112676055, "Y"=170.47552447552448}, {"X"=521.7338028169013, "Y"=170.47552447552448}, {"X"=536.7549295774646, "Y"=198.55384615384617}, {"X"=538.7577464788731, "Y"=197.55104895104898}, {"X"=539.7591549295773, "Y"=196.5482517482518}, {"X"=541.7619718309858, "Y"=195.54545454545462}, {"X"=544.7661971830985, "Y"=194.54265734265732}, {"X"=547.7704225352111, "Y"=191.53426573426577}, {"X"=550.7746478873238, "Y"=189.5286713286714}, {"X"=553.7788732394365, "Y"=186.52027972027975}, {"X"=555.781690140845, "Y"=184.51468531468538}, {"X"=557.7845070422534, "Y"=182.5090909090909}, {"X"=558.7859154929577, "Y"=181.50629370629372}, {"X"=559.7873239436618, "Y"=179.50069930069935}, {"X"=560.7887323943661, "Y"=178.49790209790217}, {"X"=563.7929577464787, "Y"=174.48671328671333}, {"X"=564.794366197183, "Y"=173.48391608391614}, {"X"=565.7957746478872, "Y"=172.48111888111896}, {"X"=568.7999999999998, "Y"=169.4727272727273}, {"X"=570.8028169014083, "Y"=166.46433566433564}, {"X"=572.8056338028167, "Y"=165.46153846153845}, {"X"=573.807042253521, "Y"=164.45874125874127}, {"X"=575.8098591549294, "Y"=162.4531468531469}, {"X"=578.8140845070421, "Y"=159.44475524475524}, {"X"=580.8169014084506, "Y"=158.44195804195806}, {"X"=582.819718309859, "Y"=157.43916083916088}, {"X"=583.8211267605633, "Y"=156.4363636363637}, {"X"=584.8225352112674, "Y"=155.4335664335665}, {"X"=587.8267605633802, "Y"=152.42517482517485}, {"X"=589.8295774647886, "Y"=150.41958041958048}, {"X"=590.8309859154928, "Y"=149.4167832167833}, {"X"=592.8338028169013, "Y"=148.413986013986}, {"X"=592.8338028169013, "Y"=147.41118881118882}, {"X"=593.8352112676055, "Y"=147.41118881118882}, {"X"=593.8352112676055, "Y"=146.40839160839164}, {"X"=594.8366197183097, "Y"=145.40559440559446}, {"X"=595.8380281690139, "Y"=144.40279720279727}, {"X"=595.8380281690139, "Y"=143.39999999999998}, {"X"=596.8394366197182, "Y"=142.3972027972028}, {"X"=596.8394366197182, "Y"=141.3944055944056}, {"X"=596.8394366197182, "Y"=142.3972027972028}, {"X"=595.8380281690139, "Y"=142.3972027972028}, {"X"=595.8380281690139, "Y"=143.39999999999998}, {"X"=594.8366197183097, "Y"=144.40279720279727}, {"X"=593.8352112676055, "Y"=146.40839160839164}, {"X"=592.8338028169013, "Y"=148.413986013986}, {"X"=591.832394366197, "Y"=150.41958041958048}, {"X"=590.8309859154928, "Y"=152.42517482517485}, {"X"=590.8309859154928, "Y"=154.43076923076922}, {"X"=589.8295774647886, "Y"=156.4363636363637}, {"X"=589.8295774647886, "Y"=158.44195804195806}, {"X"=588.8281690140843, "Y"=159.44475524475524}, {"X"=588.8281690140843, "Y"=162.4531468531469}, {"X"=587.8267605633802, "Y"=163.4559440559441}, {"X"=587.8267605633802, "Y"=165.46153846153845}, {"X"=586.8253521126759, "Y"=168.46993006993011}, {"X"=586.8253521126759, "Y"=170.47552447552448}, {"X"=586.8253521126759, "Y"=172.48111888111896}, {"X"=585.8239436619717, "Y"=174.48671328671333}, {"X"=585.8239436619717, "Y"=176.4923076923077}, {"X"=584.8225352112674, "Y"=178.49790209790217}, {"X"=584.8225352112674, "Y"=179.50069930069935}, {"X"=584.8225352112674, "Y"=181.50629370629372}, {"X"=584.8225352112674, "Y"=182.5090909090909}, {"X"=584.8225352112674, "Y"=183.51188811188808}, {"X"=584.8225352112674, "Y"=185.51748251748256}, {"X"=584.8225352112674, "Y"=186.52027972027975}, {"X"=584.8225352112674, "Y"=187.52307692307693}, {"X"=584.8225352112674, "Y"=188.5258741258741}, {"X"=585.8239436619717, "Y"=188.5258741258741}, {"X"=585.8239436619717, "Y"=189.5286713286714}, {"X"=585.8239436619717, "Y"=190.5314685314686}, {"X"=585.8239436619717, "Y"=191.53426573426577}, {"X"=586.8253521126759, "Y"=192.53706293706296}, {"X"=586.8253521126759, "Y"=193.53986013986014}, {"X"=587.8267605633802, "Y"=193.53986013986014}, {"X"=587.8267605633802, "Y"=194.54265734265732}, {"X"=588.8281690140843, "Y"=194.54265734265732}, {"X"=589.8295774647886, "Y"=194.54265734265732}, {"X"=590.8309859154928, "Y"=194.54265734265732}, {"X"=590.8309859154928, "Y"=193.53986013986014}, {"X"=591.832394366197, "Y"=193.53986013986014}, {"X"=594.8366197183097, "Y"=191.53426573426577}, {"X"=596.8394366197182, "Y"=189.5286713286714}, {"X"=597.8408450704223, "Y"=188.5258741258741}, {"X"=599.8436619718308, "Y"=186.52027972027975}, {"X"=600.8450704225351, "Y"=185.51748251748256}, {"X"=601.8464788732393, "Y"=184.51468531468538}, {"X"=603.8492957746478, "Y"=181.50629370629372}, {"X"=606.8535211267604, "Y"=178.49790209790217}, {"X"=607.8549295774646, "Y"=176.4923076923077}, {"X"=608.8563380281689, "Y"=174.48671328671333}, {"X"=609.8577464788731, "Y"=172.48111888111896}, {"X"=611.8605633802815, "Y"=170.47552447552448}, {"X"=611.8605633802815, "Y"=169.4727272727273}, {"X"=613.86338028169, "Y"=167.46713286713293}, {"X"=615.8661971830984, "Y"=164.45874125874127}, {"X"=617.869014084507, "Y"=161.45034965034972}, {"X"=618.8704225352111, "Y"=160.44755244755243}, {"X"=619.8718309859154, "Y"=159.44475524475524}, {"X"=621.8746478873238, "Y"=156.4363636363637}, {"X"=622.876056338028, "Y"=154.43076923076922}, {"X"=624.8788732394364, "Y"=151.42237762237767}, {"X"=625.8802816901407, "Y"=151.42237762237767}, {"X"=626.881690140845, "Y"=150.41958041958048}, {"X"=627.8830985915491, "Y"=148.413986013986}, {"X"=630.8873239436618, "Y"=144.40279720279727}, {"X"=632.8901408450703, "Y"=143.39999999999998}, {"X"=633.8915492957744, "Y"=142.3972027972028}, {"X"=636.8957746478872, "Y"=140.39160839160843}, {"X"=639.8999999999999, "Y"=138.38601398601406}, {"X"=640.901408450704, "Y"=136.38041958041958}, {"X"=642.9042253521126, "Y"=134.37482517482522}, {"X"=643.9056338028167, "Y"=133.37202797202804}, {"X"=644.907042253521, "Y"=133.37202797202804}, {"X"=645.9084507042252, "Y"=131.36643356643356}, {"X"=646.9098591549294, "Y"=130.36363636363637}, {"X"=646.9098591549294, "Y"=129.3608391608392}, {"X"=647.9112676056336, "Y"=129.3608391608392}, {"X"=647.9112676056336, "Y"=128.358041958042}, {"X"=648.9126760563379, "Y"=128.358041958042}, {"X"=648.9126760563379, "Y"=127.35524475524483}, {"X"=649.914084507042, "Y"=127.35524475524483}, {"X"=649.914084507042, "Y"=126.35244755244753}, {"X"=648.9126760563379, "Y"=126.35244755244753}, {"X"=710.9999999999998, "Y"=136.38041958041958}, {"X"=710.9999999999998, "Y"=135.3776223776224}, {"X"=710.9999999999998, "Y"=134.37482517482522}, {"X"=709.9985915492956, "Y"=134.37482517482522}, {"X"=709.9985915492956, "Y"=133.37202797202804}, {"X"=708.9971830985913, "Y"=133.37202797202804}, {"X"=708.9971830985913, "Y"=132.36923076923085}, {"X"=707.9957746478872, "Y"=132.36923076923085}, {"X"=707.9957746478872, "Y"=131.36643356643356}, {"X"=706.9943661971829, "Y"=131.36643356643356}, {"X"=705.9929577464787, "Y"=131.36643356643356}, {"X"=704.9915492957745, "Y"=131.36643356643356}, {"X"=703.9901408450703, "Y"=130.36363636363637}, {"X"=702.988732394366, "Y"=131.36643356643356}, {"X"=700.9859154929576, "Y"=131.36643356643356}, {"X"=698.9830985915492, "Y"=132.36923076923085}, {"X"=696.9802816901407, "Y"=133.37202797202804}, {"X"=693.976056338028, "Y"=134.37482517482522}, {"X"=692.9746478873237, "Y"=135.3776223776224}, {"X"=690.9718309859153, "Y"=135.3776223776224}, {"X"=687.9676056338027, "Y"=137.38321678321677}, {"X"=686.9661971830984, "Y"=137.38321678321677}, {"X"=685.9647887323943, "Y"=138.38601398601406}, {"X"=682.9605633802815, "Y"=140.39160839160843}, {"X"=681.9591549295773, "Y"=141.3944055944056}, {"X"=679.9563380281688, "Y"=142.3972027972028}, {"X"=678.9549295774647, "Y"=143.39999999999998}, {"X"=676.9521126760562, "Y"=144.40279720279727}, {"X"=675.950704225352, "Y"=145.40559440559446}, {"X"=674.9492957746477, "Y"=146.40839160839164}, {"X"=672.9464788732392, "Y"=147.41118881118882}, {"X"=671.9450704225351, "Y"=148.413986013986}, {"X"=669.9422535211266, "Y"=150.41958041958048}, {"X"=668.9408450704224, "Y"=150.41958041958048}, {"X"=667.9394366197181, "Y"=151.42237762237767}, {"X"=664.9352112676055, "Y"=153.42797202797203}, {"X"=661.9309859154928, "Y"=155.4335664335665}, {"X"=660.9295774647886, "Y"=155.4335664335665}, {"X"=659.9281690140843, "Y"=156.4363636363637}, {"X"=657.9253521126759, "Y"=158.44195804195806}, {"X"=655.9225352112675, "Y"=161.45034965034972}, {"X"=654.9211267605632, "Y"=162.4531468531469}, {"X"=653.919718309859, "Y"=162.4531468531469}, {"X"=652.9183098591548, "Y"=164.45874125874127}, {"X"=651.9169014084506, "Y"=167.46713286713293}, {"X"=650.9154929577463, "Y"=169.4727272727273}, {"X"=649.914084507042, "Y"=171.47832167832166}, {"X"=649.914084507042, "Y"=173.48391608391614}, {"X"=648.9126760563379, "Y"=174.48671328671333}, {"X"=647.9112676056336, "Y"=176.4923076923077}, {"X"=646.9098591549294, "Y"=177.49510489510487}, {"X"=645.9084507042252, "Y"=179.50069930069935}, {"X"=644.907042253521, "Y"=181.50629370629372}, {"X"=644.907042253521, "Y"=182.5090909090909}, {"X"=643.9056338028167, "Y"=184.51468531468538}, {"X"=643.9056338028167, "Y"=185.51748251748256}, {"X"=642.9042253521126, "Y"=186.52027972027975}, {"X"=641.9028169014083, "Y"=187.52307692307693}, {"X"=641.9028169014083, "Y"=188.5258741258741}, {"X"=640.901408450704, "Y"=189.5286713286714}, {"X"=640.901408450704, "Y"=190.5314685314686}, {"X"=640.901408450704, "Y"=191.53426573426577}, {"X"=641.9028169014083, "Y"=191.53426573426577}, {"X"=641.9028169014083, "Y"=192.53706293706296}, {"X"=641.9028169014083, "Y"=193.53986013986014}, {"X"=642.9042253521126, "Y"=195.54545454545462}, {"X"=642.9042253521126, "Y"=196.5482517482518}, {"X"=643.9056338028167, "Y"=197.55104895104898}, {"X"=644.907042253521, "Y"=197.55104895104898}, {"X"=646.9098591549294, "Y"=198.55384615384617}, {"X"=648.9126760563379, "Y"=198.55384615384617}, {"X"=651.9169014084506, "Y"=198.55384615384617}, {"X"=654.9211267605632, "Y"=198.55384615384617}, {"X"=655.9225352112675, "Y"=197.55104895104898}, {"X"=658.9267605633801, "Y"=197.55104895104898}, {"X"=660.9295774647886, "Y"=196.5482517482518}, {"X"=662.9323943661971, "Y"=195.54545454545462}, {"X"=665.9366197183097, "Y"=194.54265734265732}, {"X"=667.9394366197181, "Y"=193.53986013986014}, {"X"=670.9436619718308, "Y"=191.53426573426577}, {"X"=672.9464788732392, "Y"=189.5286713286714}, {"X"=673.9478873239435, "Y"=187.52307692307693}, {"X"=674.9492957746477, "Y"=186.52027972027975}, {"X"=676.9521126760562, "Y"=182.5090909090909}, {"X"=677.9535211267604, "Y"=181.50629370629372}, {"X"=678.9549295774647, "Y"=179.50069930069935}, {"X"=678.9549295774647, "Y"=176.4923076923077}, {"X"=679.9563380281688, "Y"=175.4895104895105}, {"X"=679.9563380281688, "Y"=174.48671328671333}, {"X"=679.9563380281688, "Y"=172.48111888111896}, {"X"=679.9563380281688, "Y"=170.47552447552448}, {"X"=678.9549295774647, "Y"=169.4727272727273}, {"X"=678.9549295774647, "Y"=168.46993006993011}, {"X"=678.9549295774647, "Y"=167.46713286713293}, {"X"=676.9521126760562, "Y"=166.46433566433564}, {"X"=676.9521126760562, "Y"=165.46153846153845}, {"X"=675.950704225352, "Y"=165.46153846153845}, {"X"=675.950704225352, "Y"=166.46433566433564}, {"X"=674.9492957746477, "Y"=166.46433566433564}, {"X"=675.950704225352, "Y"=167.46713286713293}, {"X"=676.9521126760562, "Y"=167.46713286713293}, {"X"=678.9549295774647, "Y"=167.46713286713293}, {"X"=682.9605633802815, "Y"=166.46433566433564}, {"X"=684.96338028169, "Y"=166.46433566433564}, {"X"=687.9676056338027, "Y"=166.46433566433564}, {"X"=689.9704225352111, "Y"=166.46433566433564}, {"X"=690.9718309859153, "Y"=166.46433566433564}, {"X"=692.9746478873237, "Y"=166.46433566433564}, {"X"=694.9774647887323, "Y"=166.46433566433564}, {"X"=695.9788732394364, "Y"=166.46433566433564}, {"X"=696.9802816901407, "Y"=166.46433566433564}, {"X"=696.9802816901407, "Y"=167.46713286713293}, {"X"=697.9816901408449, "Y"=167.46713286713293}, {"X"=698.9830985915492, "Y"=168.46993006993011}, {"X"=698.9830985915492, "Y"=169.4727272727273}, {"X"=699.9845070422533, "Y"=169.4727272727273}, {"X"=699.9845070422533, "Y"=170.47552447552448}, {"X"=700.9859154929576, "Y"=170.47552447552448}, {"X"=700.9859154929576, "Y"=171.47832167832166}, {"X"=700.9859154929576, "Y"=172.48111888111896}, {"X"=700.9859154929576, "Y"=173.48391608391614}, {"X"=700.9859154929576, "Y"=174.48671328671333}, {"X"=699.9845070422533, "Y"=175.4895104895105}, {"X"=699.9845070422533, "Y"=177.49510489510487}, {"X"=698.9830985915492, "Y"=179.50069930069935}, {"X"=697.9816901408449, "Y"=181.50629370629372}, {"X"=695.9788732394364, "Y"=184.51468531468538}, {"X"=693.976056338028, "Y"=186.52027972027975}, {"X"=690.9718309859153, "Y"=189.5286713286714}, {"X"=688.9690140845069, "Y"=192.53706293706296}, {"X"=687.9676056338027, "Y"=193.53986013986014}, {"X"=686.9661971830984, "Y"=194.54265734265732}, {"X"=686.9661971830984, "Y"=195.54545454545462}, {"X"=685.9647887323943, "Y"=196.5482517482518}, {"X"=685.9647887323943, "Y"=197.55104895104898}, {"X"=684.96338028169, "Y"=197.55104895104898}, {"X"=684.96338028169, "Y"=198.55384615384617}, {"X"=684.96338028169, "Y"=197.55104895104898}, {"X"=683.9619718309857, "Y"=196.5482517482518}, {"X"=700.9859154929576, "Y"=195.54545454545462}, {"X"=702.988732394366, "Y"=195.54545454545462}, {"X"=703.9901408450703, "Y"=195.54545454545462}, {"X"=706.9943661971829, "Y"=194.54265734265732}, {"X"=713.0028169014083, "Y"=193.53986013986014}, {"X"=718.0098591549294, "Y"=191.53426573426577}, {"X"=725.019718309859, "Y"=189.5286713286714}, {"X"=728.0239436619717, "Y"=188.5258741258741}, {"X"=733.0309859154928, "Y"=186.52027972027975}, {"X"=736.0352112676054, "Y"=185.51748251748256}, {"X"=739.0394366197181, "Y"=184.51468531468538}, {"X"=743.045070422535, "Y"=184.51468531468538}, {"X"=745.0478873239434, "Y"=183.51188811188808}, {"X"=746.0492957746477, "Y"=183.51188811188808}, {"X"=747.050704225352, "Y"=183.51188811188808}, {"X"=747.050704225352, "Y"=182.5090909090909}, {"X"=748.0521126760561, "Y"=182.5090909090909}, {"X"=747.050704225352, "Y"=182.5090909090909}, {"X"=746.0492957746477, "Y"=182.5090909090909}, {"X"=745.0478873239434, "Y"=182.5090909090909}, {"X"=744.0464788732393, "Y"=182.5090909090909}, {"X"=722.0154929577463, "Y"=183.51188811188808}, {"X"=723.0169014084505, "Y"=182.5090909090909}, {"X"=723.0169014084505, "Y"=181.50629370629372}, {"X"=724.0183098591548, "Y"=180.50349650349654}, {"X"=725.019718309859, "Y"=178.49790209790217}, {"X"=726.0211267605632, "Y"=177.49510489510487}, {"X"=726.0211267605632, "Y"=176.4923076923077}, {"X"=727.0225352112674, "Y"=173.48391608391614}, {"X"=728.0239436619717, "Y"=171.47832167832166}, {"X"=728.0239436619717, "Y"=169.4727272727273}, {"X"=729.0253521126759, "Y"=167.46713286713293}, {"X"=730.0267605633801, "Y"=165.46153846153845}, {"X"=731.0281690140844, "Y"=164.45874125874127}, {"X"=731.0281690140844, "Y"=163.4559440559441}, {"X"=732.0295774647885, "Y"=161.45034965034972}, {"X"=732.0295774647885, "Y"=159.44475524475524}, {"X"=733.0309859154928, "Y"=158.44195804195806}, {"X"=734.032394366197, "Y"=157.43916083916088}, {"X"=734.032394366197, "Y"=155.4335664335665}, {"X"=734.032394366197, "Y"=154.43076923076922}, {"X"=735.0338028169012, "Y"=154.43076923076922}, {"X"=735.0338028169012, "Y"=152.42517482517485}, {"X"=736.0352112676054, "Y"=151.42237762237767}, {"X"=736.0352112676054, "Y"=150.41958041958048}, {"X"=737.0366197183097, "Y"=150.41958041958048}, {"X"=738.038028169014, "Y"=148.413986013986}, {"X"=739.0394366197181, "Y"=146.40839160839164}, {"X"=740.0408450704224, "Y"=146.40839160839164}, {"X"=741.0422535211266, "Y"=145.40559440559446}, {"X"=741.0422535211266, "Y"=144.40279720279727}, {"X"=741.0422535211266, "Y"=143.39999999999998}, {"X"=742.0436619718308, "Y"=143.39999999999998}, {"X"=742.0436619718308, "Y"=142.3972027972028}, {"X"=741.0422535211266, "Y"=142.3972027972028}, {"X"=722.0154929577463, "Y"=146.40839160839164}, {"X"=723.0169014084505, "Y"=146.40839160839164}, {"X"=724.0183098591548, "Y"=146.40839160839164}, {"X"=725.019718309859, "Y"=145.40559440559446}, {"X"=728.0239436619717, "Y"=145.40559440559446}, {"X"=731.0281690140844, "Y"=145.40559440559446}, {"X"=732.0295774647885, "Y"=144.40279720279727}, {"X"=734.032394366197, "Y"=144.40279720279727}, {"X"=736.0352112676054, "Y"=144.40279720279727}, {"X"=739.0394366197181, "Y"=143.39999999999998}, {"X"=744.0464788732393, "Y"=143.39999999999998}, {"X"=746.0492957746477, "Y"=142.3972027972028}, {"X"=749.0535211267604, "Y"=142.3972027972028}, {"X"=751.0563380281689, "Y"=141.3944055944056}, {"X"=754.0605633802816, "Y"=141.3944055944056}, {"X"=757.0647887323942, "Y"=141.3944055944056}, {"X"=760.0690140845069, "Y"=140.39160839160843}, {"X"=763.0732394366196, "Y"=140.39160839160843}, {"X"=767.0788732394365, "Y"=139.38881118881125}, {"X"=771.0845070422533, "Y"=139.38881118881125}, {"X"=774.088732394366, "Y"=139.38881118881125}, {"X"=776.0915492957745, "Y"=139.38881118881125}, {"X"=777.0929577464786, "Y"=139.38881118881125}, {"X"=778.0943661971829, "Y"=139.38881118881125}, {"X"=779.0957746478871, "Y"=139.38881118881125}, {"X"=780.0971830985914, "Y"=139.38881118881125}, {"X"=781.0985915492956, "Y"=139.38881118881125}, {"X"=782.0999999999998, "Y"=139.38881118881125}, {"X"=783.1014084507041, "Y"=139.38881118881125}, {"X"=782.0999999999998, "Y"=139.38881118881125}, {"X"=763.0732394366196, "Y"=176.4923076923077}, {"X"=764.0746478873237, "Y"=175.4895104895105}, {"X"=765.076056338028, "Y"=175.4895104895105}, {"X"=765.076056338028, "Y"=174.48671328671333}, {"X"=766.0774647887322, "Y"=174.48671328671333}, {"X"=767.0788732394365, "Y"=173.48391608391614}, {"X"=768.0802816901406, "Y"=173.48391608391614}, {"X"=768.0802816901406, "Y"=172.48111888111896}, {"X"=769.0816901408449, "Y"=172.48111888111896}, {"X"=772.0859154929576, "Y"=169.4727272727273}, {"X"=773.0873239436618, "Y"=168.46993006993011}, {"X"=773.0873239436618, "Y"=167.46713286713293}, {"X"=775.0901408450702, "Y"=166.46433566433564}, {"X"=776.0915492957745, "Y"=165.46153846153845}, {"X"=777.0929577464786, "Y"=164.45874125874127}, {"X"=778.0943661971829, "Y"=163.4559440559441}, {"X"=779.0957746478871, "Y"=162.4531468531469}, {"X"=780.0971830985914, "Y"=161.45034965034972}, {"X"=781.0985915492956, "Y"=161.45034965034972}, {"X"=783.1014084507041, "Y"=159.44475524475524}, {"X"=785.1042253521125, "Y"=158.44195804195806}, {"X"=786.1056338028167, "Y"=156.4363636363637}, {"X"=787.107042253521, "Y"=155.4335664335665}, {"X"=788.1084507042252, "Y"=154.43076923076922}, {"X"=790.1112676056337, "Y"=153.42797202797203}, {"X"=790.1112676056337, "Y"=152.42517482517485}, {"X"=791.1126760563378, "Y"=152.42517482517485}, {"X"=791.1126760563378, "Y"=151.42237762237767}, {"X"=794.1169014084505, "Y"=149.4167832167833}, {"X"=796.119718309859, "Y"=148.413986013986}, {"X"=798.1225352112674, "Y"=147.41118881118882}, {"X"=799.1239436619717, "Y"=146.40839160839164}, {"X"=800.1253521126758, "Y"=145.40559440559446}, {"X"=801.1267605633801, "Y"=145.40559440559446}, {"X"=803.1295774647886, "Y"=143.39999999999998}, {"X"=804.1309859154927, "Y"=142.3972027972028}, {"X"=805.132394366197, "Y"=142.3972027972028}, {"X"=805.132394366197, "Y"=141.3944055944056}, {"X"=806.1338028169013, "Y"=141.3944055944056}, {"X"=806.1338028169013, "Y"=140.39160839160843}, {"X"=807.1352112676054, "Y"=140.39160839160843}, {"X"=807.1352112676054, "Y"=139.38881118881125}, {"X"=808.1366197183097, "Y"=139.38881118881125}, {"X"=808.1366197183097, "Y"=138.38601398601406}, {"X"=809.1380281690139, "Y"=138.38601398601406}, {"X"=809.1380281690139, "Y"=137.38321678321677}, {"X"=809.1380281690139, "Y"=138.38601398601406}, {"X"=809.1380281690139, "Y"=139.38881118881125}, {"X"=808.1366197183097, "Y"=139.38881118881125}, {"X"=808.1366197183097, "Y"=141.3944055944056}, {"X"=807.1352112676054, "Y"=143.39999999999998}, {"X"=806.1338028169013, "Y"=145.40559440559446}, {"X"=806.1338028169013, "Y"=147.41118881118882}, {"X"=805.132394366197, "Y"=148.413986013986}, {"X"=804.1309859154927, "Y"=150.41958041958048}, {"X"=804.1309859154927, "Y"=151.42237762237767}, {"X"=803.1295774647886, "Y"=154.43076923076922}, {"X"=802.1281690140843, "Y"=156.4363636363637}, {"X"=801.1267605633801, "Y"=157.43916083916088}, {"X"=800.1253521126758, "Y"=158.44195804195806}, {"X"=800.1253521126758, "Y"=159.44475524475524}, {"X"=799.1239436619717, "Y"=159.44475524475524}, {"X"=799.1239436619717, "Y"=160.44755244755243}, {"X"=798.1225352112674, "Y"=161.45034965034972}, {"X"=798.1225352112674, "Y"=162.4531468531469}, {"X"=798.1225352112674, "Y"=163.4559440559441}, {"X"=798.1225352112674, "Y"=164.45874125874127}, {"X"=798.1225352112674, "Y"=165.46153846153845}, {"X"=799.1239436619717, "Y"=166.46433566433564}, {"X"=799.1239436619717, "Y"=167.46713286713293}, {"X"=799.1239436619717, "Y"=168.46993006993011}, {"X"=800.1253521126758, "Y"=168.46993006993011}, {"X"=800.1253521126758, "Y"=169.4727272727273}, {"X"=800.1253521126758, "Y"=170.47552447552448}, {"X"=801.1267605633801, "Y"=170.47552447552448}, {"X"=802.1281690140843, "Y"=170.47552447552448}, {"X"=803.1295774647886, "Y"=170.47552447552448}, {"X"=804.1309859154927, "Y"=170.47552447552448}, {"X"=805.132394366197, "Y"=169.4727272727273}, {"X"=808.1366197183097, "Y"=168.46993006993011}, {"X"=810.1394366197181, "Y"=167.46713286713293}, {"X"=811.1408450704223, "Y"=166.46433566433564}, {"X"=813.1436619718307, "Y"=165.46153846153845}, {"X"=816.1478873239435, "Y"=163.4559440559441}, {"X"=818.1507042253519, "Y"=163.4559440559441}, {"X"=820.1535211267603, "Y"=161.45034965034972}, {"X"=821.1549295774646, "Y"=161.45034965034972}, {"X"=822.1563380281688, "Y"=160.44755244755243}, {"X"=823.157746478873, "Y"=159.44475524475524}, {"X"=825.1605633802815, "Y"=158.44195804195806}, {"X"=827.1633802816899, "Y"=156.4363636363637}, {"X"=829.1661971830983, "Y"=155.4335664335665}, {"X"=831.1690140845069, "Y"=154.43076923076922}, {"X"=832.1704225352111, "Y"=153.42797202797203}, {"X"=833.1718309859153, "Y"=152.42517482517485}, {"X"=835.1746478873238, "Y"=151.42237762237767}, {"X"=836.1760563380279, "Y"=150.41958041958048}, {"X"=838.1788732394364, "Y"=148.413986013986}, {"X"=839.1802816901406, "Y"=147.41118881118882}, {"X"=840.1816901408449, "Y"=147.41118881118882}, {"X"=841.1830985915491, "Y"=146.40839160839164}, {"X"=844.1873239436618, "Y"=144.40279720279727}, {"X"=845.188732394366, "Y"=143.39999999999998}, {"X"=846.1901408450702, "Y"=142.3972027972028}, {"X"=849.194366197183, "Y"=140.39160839160843}, {"X"=850.1957746478871, "Y"=138.38601398601406}, {"X"=852.1985915492955, "Y"=137.38321678321677}, {"X"=854.201408450704, "Y"=135.3776223776224}, {"X"=856.2042253521124, "Y"=134.37482517482522}, {"X"=857.2056338028167, "Y"=133.37202797202804}, {"X"=857.2056338028167, "Y"=132.36923076923085}, {"X"=858.207042253521, "Y"=132.36923076923085}, {"X"=859.2084507042251, "Y"=131.36643356643356}, {"X"=860.2098591549294, "Y"=130.36363636363637}, {"X"=862.2126760563378, "Y"=129.3608391608392}, {"X"=862.2126760563378, "Y"=128.358041958042}, {"X"=863.214084507042, "Y"=128.358041958042}, {"X"=863.214084507042, "Y"=127.35524475524483}, {"X"=864.2154929577463, "Y"=127.35524475524483}, {"X"=864.2154929577463, "Y"=126.35244755244753}, {"X"=863.214084507042, "Y"=126.35244755244753}, {"X"=911.2816901408448, "Y"=124.34685314685316}, {"X"=910.2802816901407, "Y"=124.34685314685316}, {"X"=909.2788732394364, "Y"=124.34685314685316}, {"X"=908.2774647887322, "Y"=124.34685314685316}, {"X"=905.2732394366195, "Y"=124.34685314685316}, {"X"=902.2690140845068, "Y"=125.34965034965035}, {"X"=900.2661971830984, "Y"=125.34965034965035}, {"X"=899.2647887323942, "Y"=125.34965034965035}, {"X"=897.2619718309857, "Y"=125.34965034965035}, {"X"=896.2605633802815, "Y"=125.34965034965035}, {"X"=895.2591549295772, "Y"=124.34685314685316}, {"X"=894.2577464788731, "Y"=124.34685314685316}, {"X"=893.2563380281688, "Y"=124.34685314685316}, {"X"=891.2535211267603, "Y"=125.34965034965035}, {"X"=890.2521126760561, "Y"=125.34965034965035}, {"X"=888.2492957746476, "Y"=125.34965034965035}, {"X"=887.2478873239435, "Y"=125.34965034965035}, {"X"=884.2436619718308, "Y"=126.35244755244753}, {"X"=883.2422535211266, "Y"=126.35244755244753}, {"X"=882.2408450704223, "Y"=126.35244755244753}, {"X"=881.239436619718, "Y"=126.35244755244753}, {"X"=880.2380281690139, "Y"=127.35524475524483}, {"X"=878.2352112676055, "Y"=127.35524475524483}, {"X"=877.2338028169012, "Y"=128.358041958042}, {"X"=875.2309859154927, "Y"=128.358041958042}, {"X"=874.2295774647886, "Y"=129.3608391608392}, {"X"=873.2281690140843, "Y"=129.3608391608392}, {"X"=872.22676056338, "Y"=130.36363636363637}, {"X"=870.2239436619716, "Y"=130.36363636363637}, {"X"=870.2239436619716, "Y"=131.36643356643356}, {"X"=868.2211267605632, "Y"=131.36643356643356}, {"X"=867.219718309859, "Y"=132.36923076923085}, {"X"=867.219718309859, "Y"=133.37202797202804}, {"X"=866.2183098591547, "Y"=134.37482517482522}, {"X"=864.2154929577463, "Y"=136.38041958041958}, {"X"=863.214084507042, "Y"=139.38881118881125}, {"X"=861.2112676056336, "Y"=141.3944055944056}, {"X"=861.2112676056336, "Y"=142.3972027972028}, {"X"=861.2112676056336, "Y"=144.40279720279727}, {"X"=860.2098591549294, "Y"=146.40839160839164}, {"X"=859.2084507042251, "Y"=148.413986013986}, {"X"=859.2084507042251, "Y"=149.4167832167833}, {"X"=858.207042253521, "Y"=151.42237762237767}, {"X"=858.207042253521, "Y"=152.42517482517485}, {"X"=858.207042253521, "Y"=153.42797202797203}, {"X"=856.2042253521124, "Y"=156.4363636363637}, {"X"=855.2028169014083, "Y"=157.43916083916088}, {"X"=855.2028169014083, "Y"=158.44195804195806}, {"X"=854.201408450704, "Y"=158.44195804195806}, {"X"=854.201408450704, "Y"=159.44475524475524}, {"X"=853.1999999999998, "Y"=160.44755244755243}, {"X"=852.1985915492955, "Y"=161.45034965034972}, {"X"=852.1985915492955, "Y"=162.4531468531469}, {"X"=852.1985915492955, "Y"=163.4559440559441}, {"X"=851.1971830985914, "Y"=163.4559440559441}, {"X"=851.1971830985914, "Y"=164.45874125874127}, {"X"=851.1971830985914, "Y"=165.46153846153845}, {"X"=850.1957746478871, "Y"=165.46153846153845}, {"X"=850.1957746478871, "Y"=166.46433566433564}, {"X"=850.1957746478871, "Y"=167.46713286713293}, {"X"=850.1957746478871, "Y"=168.46993006993011}, {"X"=850.1957746478871, "Y"=169.4727272727273}, {"X"=851.1971830985914, "Y"=169.4727272727273}, {"X"=851.1971830985914, "Y"=170.47552447552448}, {"X"=852.1985915492955, "Y"=170.47552447552448}, {"X"=852.1985915492955, "Y"=171.47832167832166}, {"X"=853.1999999999998, "Y"=171.47832167832166}, {"X"=854.201408450704, "Y"=171.47832167832166}, {"X"=855.2028169014083, "Y"=171.47832167832166}, {"X"=855.2028169014083, "Y"=172.48111888111896}, {"X"=856.2042253521124, "Y"=172.48111888111896}, {"X"=857.2056338028167, "Y"=172.48111888111896}, {"X"=858.207042253521, "Y"=172.48111888111896}, {"X"=859.2084507042251, "Y"=172.48111888111896}, {"X"=860.2098591549294, "Y"=172.48111888111896}, {"X"=861.2112676056336, "Y"=172.48111888111896}, {"X"=864.2154929577463, "Y"=171.47832167832166}, {"X"=867.219718309859, "Y"=171.47832167832166}, {"X"=869.2225352112674, "Y"=171.47832167832166}, {"X"=870.2239436619716, "Y"=170.47552447552448}, {"X"=872.22676056338, "Y"=171.47832167832166}, {"X"=874.2295774647886, "Y"=170.47552447552448}, {"X"=876.232394366197, "Y"=170.47552447552448}, {"X"=877.2338028169012, "Y"=170.47552447552448}, {"X"=880.2380281690139, "Y"=169.4727272727273}, {"X"=881.239436619718, "Y"=169.4727272727273}, {"X"=883.2422535211266, "Y"=169.4727272727273}, {"X"=886.2464788732392, "Y"=167.46713286713293}, {"X"=888.2492957746476, "Y"=167.46713286713293}, {"X"=889.2507042253519, "Y"=166.46433566433564}, {"X"=891.2535211267603, "Y"=165.46153846153845}, {"X"=892.2549295774646, "Y"=165.46153846153845}, {"X"=893.2563380281688, "Y"=165.46153846153845}, {"X"=894.2577464788731, "Y"=165.46153846153845}, {"X"=895.2591549295772, "Y"=165.46153846153845}, {"X"=896.2605633802815, "Y"=164.45874125874127}, {"X"=897.2619718309857, "Y"=164.45874125874127}, {"X"=898.2633802816899, "Y"=164.45874125874127}, {"X"=898.2633802816899, "Y"=163.4559440559441}, {"X"=899.2647887323942, "Y"=163.4559440559441}, {"X"=900.2661971830984, "Y"=162.4531468531469}, {"X"=901.2676056338026, "Y"=162.4531468531469}, {"X"=900.2661971830984, "Y"=162.4531468531469}, {"X"=901.2676056338026, "Y"=162.4531468531469}, {"X"=900.2661971830984, "Y"=162.4531468531469}, {"X"=901.2676056338026, "Y"=162.4531468531469}, {"X"=900.2661971830984, "Y"=162.4531468531469}, {"X"=899.2647887323942, "Y"=162.4531468531469}, {"X"=899.2647887323942, "Y"=163.4559440559441}, {"X"=898.2633802816899, "Y"=163.4559440559441}, {"X"=897.2619718309857, "Y"=163.4559440559441}, {"X"=894.2577464788731, "Y"=163.4559440559441}, {"X"=891.2535211267603, "Y"=164.45874125874127}, {"X"=889.2507042253519, "Y"=164.45874125874127}, {"X"=887.2478873239435, "Y"=164.45874125874127}, {"X"=884.2436619718308, "Y"=165.46153846153845}, {"X"=881.239436619718, "Y"=165.46153846153845}, {"X"=877.2338028169012, "Y"=165.46153846153845}, {"X"=872.22676056338, "Y"=165.46153846153845}, {"X"=871.2253521126759, "Y"=165.46153846153845}, {"X"=869.2225352112674, "Y"=166.46433566433564}, {"X"=865.2169014084506, "Y"=166.46433566433564}, {"X"=863.214084507042, "Y"=166.46433566433564}, {"X"=859.2084507042251, "Y"=166.46433566433564}, {"X"=857.2056338028167, "Y"=167.46713286713293}, {"X"=853.1999999999998, "Y"=167.46713286713293}, {"X"=852.1985915492955, "Y"=167.46713286713293}, {"X"=850.1957746478871, "Y"=167.46713286713293}, {"X"=849.194366197183, "Y"=167.46713286713293}, {"X"=848.1929577464787, "Y"=167.46713286713293}, {"X"=848.1929577464787, "Y"=166.46433566433564}, {"X"=848.1929577464787, "Y"=167.46713286713293}, {"X"=848.1929577464787, "Y"=166.46433566433564}, {"X"=848.1929577464787, "Y"=167.46713286713293}, {"X"=849.194366197183, "Y"=165.46153846153845}, {"X"=849.194366197183, "Y"=163.4559440559441}, {"X"=850.1957746478871, "Y"=162.4531468531469}, {"X"=851.1971830985914, "Y"=160.44755244755243}, {"X"=851.1971830985914, "Y"=158.44195804195806}, {"X"=851.1971830985914, "Y"=157.43916083916088}, {"X"=852.1985915492955, "Y"=156.4363636363637}, {"X"=852.1985915492955, "Y"=155.4335664335665}, {"X"=852.1985915492955, "Y"=154.43076923076922}, {"X"=852.1985915492955, "Y"=153.42797202797203}, {"X"=853.1999999999998, "Y"=153.42797202797203}, {"X"=854.201408450704, "Y"=153.42797202797203}, {"X"=855.2028169014083, "Y"=153.42797202797203}, {"X"=857.2056338028167, "Y"=153.42797202797203}, {"X"=861.2112676056336, "Y"=153.42797202797203}, {"X"=864.2154929577463, "Y"=152.42517482517485}, {"X"=867.219718309859, "Y"=152.42517482517485}, {"X"=871.2253521126759, "Y"=152.42517482517485}, {"X"=874.2295774647886, "Y"=152.42517482517485}, {"X"=878.2352112676055, "Y"=151.42237762237767}, {"X"=880.2380281690139, "Y"=151.42237762237767}, {"X"=883.2422535211266, "Y"=150.41958041958048}, {"X"=885.245070422535, "Y"=150.41958041958048}, {"X"=887.2478873239435, "Y"=150.41958041958048}, {"X"=889.2507042253519, "Y"=150.41958041958048}, {"X"=890.2521126760561, "Y"=150.41958041958048}, {"X"=891.2535211267603, "Y"=149.4167832167833}, {"X"=892.2549295774646, "Y"=149.4167832167833}, {"X"=893.2563380281688, "Y"=149.4167832167833}, {"X"=894.2577464788731, "Y"=149.4167832167833}, {"X"=895.2591549295772, "Y"=149.4167832167833}, {"X"=896.2605633802815, "Y"=148.413986013986}, {"X"=896.2605633802815, "Y"=149.4167832167833}, {"X"=897.2619718309857, "Y"=149.4167832167833}, {"X"=897.2619718309857, "Y"=148.413986013986}, {"X"=896.2605633802815, "Y"=148.413986013986}, {"X"=934.314084507042, "Y"=131.36643356643356}, {"X"=933.3126760563379, "Y"=131.36643356643356}, {"X"=932.3112676056336, "Y"=132.36923076923085}, {"X"=932.3112676056336, "Y"=133.37202797202804}, {"X"=931.3098591549293, "Y"=134.37482517482522}, {"X"=929.3070422535209, "Y"=135.3776223776224}, {"X"=928.3056338028167, "Y"=137.38321678321677}, {"X"=926.3028169014083, "Y"=138.38601398601406}, {"X"=923.2985915492956, "Y"=141.3944055944056}, {"X"=922.2971830985913, "Y"=143.39999999999998}, {"X"=921.2957746478871, "Y"=144.40279720279727}, {"X"=920.2943661971829, "Y"=145.40559440559446}, {"X"=918.2915492957744, "Y"=146.40839160839164}, {"X"=918.2915492957744, "Y"=147.41118881118882}, {"X"=916.288732394366, "Y"=148.413986013986}, {"X"=915.2873239436617, "Y"=149.4167832167833}, {"X"=914.2859154929575, "Y"=150.41958041958048}, {"X"=913.2845070422533, "Y"=151.42237762237767}, {"X"=911.2816901408448, "Y"=153.42797202797203}, {"X"=910.2802816901407, "Y"=154.43076923076922}, {"X"=909.2788732394364, "Y"=155.4335664335665}, {"X"=909.2788732394364, "Y"=156.4363636363637}, {"X"=908.2774647887322, "Y"=156.4363636363637}, {"X"=908.2774647887322, "Y"=157.43916083916088}, {"X"=907.276056338028, "Y"=157.43916083916088}, {"X"=907.276056338028, "Y"=158.44195804195806}, {"X"=906.2746478873237, "Y"=158.44195804195806}, {"X"=906.2746478873237, "Y"=159.44475524475524}, {"X"=906.2746478873237, "Y"=160.44755244755243}, {"X"=906.2746478873237, "Y"=161.45034965034972}, {"X"=906.2746478873237, "Y"=162.4531468531469}, {"X"=907.276056338028, "Y"=162.4531468531469}, {"X"=908.2774647887322, "Y"=162.4531468531469}, {"X"=909.2788732394364, "Y"=162.4531468531469}, {"X"=910.2802816901407, "Y"=162.4531468531469}, {"X"=911.2816901408448, "Y"=162.4531468531469}, {"X"=912.2830985915491, "Y"=162.4531468531469}, {"X"=913.2845070422533, "Y"=162.4531468531469}, {"X"=914.2859154929575, "Y"=162.4531468531469}, {"X"=915.2873239436617, "Y"=162.4531468531469}, {"X"=917.2901408450703, "Y"=162.4531468531469}, {"X"=918.2915492957744, "Y"=163.4559440559441}, {"X"=919.2929577464787, "Y"=163.4559440559441}, {"X"=921.2957746478871, "Y"=163.4559440559441}, {"X"=923.2985915492956, "Y"=162.4531468531469}, {"X"=925.301408450704, "Y"=162.4531468531469}, {"X"=926.3028169014083, "Y"=162.4531468531469}, {"X"=929.3070422535209, "Y"=162.4531468531469}, {"X"=930.3084507042252, "Y"=162.4531468531469}, {"X"=931.3098591549293, "Y"=161.45034965034972}, {"X"=932.3112676056336, "Y"=161.45034965034972}, {"X"=934.314084507042, "Y"=161.45034965034972}, {"X"=936.3169014084505, "Y"=161.45034965034972}, {"X"=938.3197183098589, "Y"=161.45034965034972}, {"X"=939.3211267605632, "Y"=160.44755244755243}, {"X"=941.3239436619716, "Y"=160.44755244755243}, {"X"=943.32676056338, "Y"=160.44755244755243}, {"X"=944.3281690140843, "Y"=159.44475524475524}, {"X"=945.3295774647885, "Y"=159.44475524475524}, {"X"=947.3323943661969, "Y"=159.44475524475524}, {"X"=949.3352112676054, "Y"=159.44475524475524}, {"X"=950.3366197183096, "Y"=159.44475524475524}, {"X"=952.3394366197182, "Y"=159.44475524475524}, {"X"=954.3422535211265, "Y"=159.44475524475524}, {"X"=955.3436619718308, "Y"=159.44475524475524}, {"X"=956.3450704225351, "Y"=159.44475524475524}, {"X"=956.3450704225351, "Y"=158.44195804195806}, {"X"=957.3464788732391, "Y"=158.44195804195806}, {"X"=958.3478873239434, "Y"=158.44195804195806}, {"X"=957.3464788732391, "Y"=158.44195804195806}, {"X"=956.3450704225351, "Y"=158.44195804195806}, {"X"=956.3450704225351, "Y"=159.44475524475524}, {"X"=955.3436619718308, "Y"=159.44475524475524}, {"X"=954.3422535211265, "Y"=159.44475524475524}, {"X"=952.3394366197182, "Y"=160.44755244755243}, {"X"=951.3380281690139, "Y"=160.44755244755243}, {"X"=949.3352112676054, "Y"=161.45034965034972}, {"X"=945.3295774647885, "Y"=161.45034965034972}, {"X"=944.3281690140843, "Y"=161.45034965034972}, {"X"=942.3253521126759, "Y"=161.45034965034972}, {"X"=938.3197183098589, "Y"=162.4531468531469}, {"X"=935.3154929577463, "Y"=162.4531468531469}, {"X"=931.3098591549293, "Y"=162.4531468531469}, {"X"=927.3042253521124, "Y"=162.4531468531469}, {"X"=924.2999999999997, "Y"=162.4531468531469}, {"X"=923.2985915492956, "Y"=162.4531468531469}, {"X"=921.2957746478871, "Y"=162.4531468531469}, {"X"=919.2929577464787, "Y"=162.4531468531469}, {"X"=917.2901408450703, "Y"=162.4531468531469}, {"X"=916.288732394366, "Y"=162.4531468531469}, {"X"=915.2873239436617, "Y"=162.4531468531469}, {"X"=915.2873239436617, "Y"=161.45034965034972}, {"X"=914.2859154929575, "Y"=161.45034965034972}, {"X"=913.2845070422533, "Y"=161.45034965034972}, {"X"=913.2845070422533, "Y"=160.44755244755243}, {"X"=912.2830985915491, "Y"=159.44475524475524}, {"X"=912.2830985915491, "Y"=158.44195804195806}, {"X"=911.2816901408448, "Y"=158.44195804195806}, {"X"=910.2802816901407, "Y"=157.43916083916088}, {"X"=910.2802816901407, "Y"=156.4363636363637}, {"X"=910.2802816901407, "Y"=155.4335664335665}, {"X"=910.2802816901407, "Y"=154.43076923076922}, {"X"=911.2816901408448, "Y"=153.42797202797203}, {"X"=911.2816901408448, "Y"=152.42517482517485}, {"X"=911.2816901408448, "Y"=151.42237762237767}, {"X"=912.2830985915491, "Y"=151.42237762237767}, {"X"=912.2830985915491, "Y"=150.41958041958048}, {"X"=913.2845070422533, "Y"=149.4167832167833}, {"X"=914.2859154929575, "Y"=148.413986013986}, {"X"=914.2859154929575, "Y"=147.41118881118882}, {"X"=915.2873239436617, "Y"=146.40839160839164}, {"X"=916.288732394366, "Y"=145.40559440559446}, {"X"=917.2901408450703, "Y"=144.40279720279727}, {"X"=917.2901408450703, "Y"=143.39999999999998}, {"X"=918.2915492957744, "Y"=143.39999999999998}, {"X"=919.2929577464787, "Y"=141.3944055944056}, {"X"=920.2943661971829, "Y"=139.38881118881125}, {"X"=922.2971830985913, "Y"=136.38041958041958}, {"X"=922.2971830985913, "Y"=135.3776223776224}, {"X"=924.2999999999997, "Y"=132.36923076923085}, {"X"=925.301408450704, "Y"=131.36643356643356}, {"X"=926.3028169014083, "Y"=129.3608391608392}, {"X"=927.3042253521124, "Y"=129.3608391608392}, {"X"=927.3042253521124, "Y"=128.358041958042}, {"X"=927.3042253521124, "Y"=127.35524475524483}, {"X"=928.3056338028167, "Y"=127.35524475524483}, {"X"=928.3056338028167, "Y"=126.35244755244753}, {"X"=929.3070422535209, "Y"=125.34965034965035}, {"X"=930.3084507042252, "Y"=124.34685314685316}, {"X"=931.3098591549293, "Y"=124.34685314685316}, {"X"=932.3112676056336, "Y"=124.34685314685316}, {"X"=933.3126760563379, "Y"=124.34685314685316}, {"X"=933.3126760563379, "Y"=125.34965034965035}, {"X"=935.3154929577463, "Y"=125.34965034965035}, {"X"=937.3183098591547, "Y"=125.34965034965035}, {"X"=941.3239436619716, "Y"=124.34685314685316}, {"X"=943.32676056338, "Y"=124.34685314685316}, {"X"=948.3338028169012, "Y"=123.34405594405598}, {"X"=951.3380281690139, "Y"=123.34405594405598}, {"X"=955.3436619718308, "Y"=122.3412587412588}, {"X"=958.3478873239434, "Y"=122.3412587412588}, {"X"=959.3492957746477, "Y"=122.3412587412588}, {"X"=963.3549295774645, "Y"=122.3412587412588}, {"X"=966.3591549295771, "Y"=121.33846153846162}, {"X"=967.3605633802814, "Y"=121.33846153846162}, {"X"=969.36338028169, "Y"=121.33846153846162}, {"X"=972.3676056338026, "Y"=122.3412587412588}, {"X"=973.3690140845068, "Y"=122.3412587412588}, {"X"=974.3704225352111, "Y"=122.3412587412588}, {"X"=975.3718309859152, "Y"=122.3412587412588}, {"X"=976.3732394366194, "Y"=121.33846153846162}, {"X"=977.3746478873237, "Y"=121.33846153846162}, {"X"=978.376056338028, "Y"=121.33846153846162}, {"X"=979.3774647887323, "Y"=121.33846153846162}, {"X"=980.3788732394363, "Y"=122.3412587412588}, {"X"=976.3732394366194, "Y"=122.3412587412588}, {"X"=974.3704225352111, "Y"=122.3412587412588}, {"X"=969.36338028169, "Y"=123.34405594405598}, {"X"=963.3549295774645, "Y"=124.34685314685316}, {"X"=954.3422535211265, "Y"=124.34685314685316}, {"X"=949.3352112676054, "Y"=125.34965034965035}, {"X"=946.3309859154928, "Y"=125.34965034965035}, {"X"=944.3281690140843, "Y"=126.35244755244753}, {"X"=942.3253521126759, "Y"=126.35244755244753}, {"X"=939.3211267605632, "Y"=126.35244755244753}, {"X"=939.3211267605632, "Y"=127.35524475524483}, {"X"=937.3183098591547, "Y"=127.35524475524483}, {"X"=935.3154929577463, "Y"=127.35524475524483}, {"X"=933.3126760563379, "Y"=128.358041958042}, {"X"=931.3098591549293, "Y"=128.358041958042}, {"X"=929.3070422535209, "Y"=129.3608391608392}, {"X"=928.3056338028167, "Y"=130.36363636363637}, {"X"=925.301408450704, "Y"=133.37202797202804}, {"X"=923.2985915492956, "Y"=134.37482517482522}, {"X"=921.2957746478871, "Y"=137.38321678321677}, {"X"=919.2929577464787, "Y"=138.38601398601406}, {"X"=918.2915492957744, "Y"=139.38881118881125}, {"X"=918.2915492957744, "Y"=140.39160839160843}, {"X"=917.2901408450703, "Y"=142.3972027972028}, {"X"=917.2901408450703, "Y"=143.39999999999998}, {"X"=917.2901408450703, "Y"=144.40279720279727}, {"X"=917.2901408450703, "Y"=145.40559440559446}, {"X"=916.288732394366, "Y"=145.40559440559446}, {"X"=916.288732394366, "Y"=146.40839160839164}, {"X"=916.288732394366, "Y"=147.41118881118882}, {"X"=917.2901408450703, "Y"=147.41118881118882}, {"X"=918.2915492957744, "Y"=147.41118881118882}, {"X"=919.2929577464787, "Y"=147.41118881118882}, {"X"=920.2943661971829, "Y"=147.41118881118882}, {"X"=924.2999999999997, "Y"=146.40839160839164}, {"X"=927.3042253521124, "Y"=146.40839160839164}, {"X"=931.3098591549293, "Y"=145.40559440559446}, {"X"=937.3183098591547, "Y"=145.40559440559446}, {"X"=942.3253521126759, "Y"=144.40279720279727}, {"X"=944.3281690140843, "Y"=144.40279720279727}, {"X"=948.3338028169012, "Y"=144.40279720279727}, {"X"=952.3394366197182, "Y"=143.39999999999998}, {"X"=955.3436619718308, "Y"=143.39999999999998}, {"X"=956.3450704225351, "Y"=143.39999999999998}, {"X"=957.3464788732391, "Y"=142.3972027972028}, {"X"=960.3507042253519, "Y"=142.3972027972028}, {"X"=962.3535211267603, "Y"=142.3972027972028}, {"X"=963.3549295774645, "Y"=142.3972027972028}, {"X"=964.3563380281688, "Y"=142.3972027972028}, {"X"=965.3577464788731, "Y"=142.3972027972028}, {"X"=966.3591549295771, "Y"=142.3972027972028}, {"X"=967.3605633802814, "Y"=142.3972027972028}, {"X"=968.3619718309857, "Y"=142.3972027972028}, {"X"=969.36338028169, "Y"=142.3972027972028}, {"X"=970.3647887323942, "Y"=142.3972027972028}, {"X"=971.3661971830983, "Y"=141.3944055944056}, {"X"=972.3676056338026, "Y"=141.3944055944056}, {"X"=973.3690140845068, "Y"=141.3944055944056}, {"X"=974.3704225352111, "Y"=141.3944055944056}, {"X"=975.3718309859152, "Y"=141.3944055944056}, {"X"=976.3732394366194, "Y"=141.3944055944056}, {"X"=977.3746478873237, "Y"=141.3944055944056}, {"X"=978.376056338028, "Y"=141.3944055944056}, {"X"=979.3774647887323, "Y"=141.3944055944056}, {"X"=980.3788732394363, "Y"=141.3944055944056}, {"X"=981.3802816901406, "Y"=140.39160839160843}, {"X"=982.3816901408449, "Y"=140.39160839160843}, {"X"=983.3830985915491, "Y"=140.39160839160843}, {"X"=983.3830985915491, "Y"=139.38881118881125}, {"X"=983.3830985915491, "Y"=138.38601398601406}, {"X"=984.3845070422532, "Y"=137.38321678321677}, {"X"=984.3845070422532, "Y"=136.38041958041958}, {"X"=985.3859154929575, "Y"=135.3776223776224}, {"X"=986.3873239436617, "Y"=135.3776223776224}, {"X"=986.3873239436617, "Y"=134.37482517482522}, {"X"=987.388732394366, "Y"=133.37202797202804}, {"X"=987.388732394366, "Y"=132.36923076923085}, {"X"=989.3915492957743, "Y"=129.3608391608392}, {"X"=990.3929577464786, "Y"=128.358041958042}, {"X"=991.3943661971829, "Y"=127.35524475524483}, {"X"=991.3943661971829, "Y"=126.35244755244753}, {"X"=993.3971830985914, "Y"=125.34965034965035}, {"X"=994.3985915492955, "Y"=124.34685314685316}, {"X"=995.3999999999997, "Y"=124.34685314685316}, {"X"=997.4028169014083, "Y"=123.34405594405598}, {"X"=998.4042253521123, "Y"=123.34405594405598}, {"X"=1000.4070422535209, "Y"=122.3412587412588}, {"X"=1001.4084507042252, "Y"=122.3412587412588}, {"X"=1002.4098591549294, "Y"=122.3412587412588}, {"X"=1005.414084507042, "Y"=120.33566433566432}, {"X"=1006.4154929577463, "Y"=120.33566433566432}, {"X"=1008.4183098591546, "Y"=119.33286713286714}, {"X"=1009.4197183098589, "Y"=119.33286713286714}, {"X"=1010.4211267605632, "Y"=119.33286713286714}, {"X"=1012.4239436619715, "Y"=119.33286713286714}, {"X"=1013.4253521126758, "Y"=118.33006993006995}, {"X"=1014.4267605633801, "Y"=118.33006993006995}, {"X"=1015.4281690140843, "Y"=118.33006993006995}, {"X"=1017.4309859154927, "Y"=119.33286713286714}, {"X"=1018.432394366197, "Y"=119.33286713286714}, {"X"=1019.4338028169012, "Y"=119.33286713286714}, {"X"=1019.4338028169012, "Y"=120.33566433566432}, {"X"=1021.4366197183095, "Y"=121.33846153846162}, {"X"=1021.4366197183095, "Y"=122.3412587412588}, {"X"=1021.4366197183095, "Y"=125.34965034965035}, {"X"=1021.4366197183095, "Y"=128.358041958042}, {"X"=1019.4338028169012, "Y"=131.36643356643356}, {"X"=1018.432394366197, "Y"=132.36923076923085}, {"X"=1016.4295774647884, "Y"=134.37482517482522}, {"X"=1013.4253521126758, "Y"=136.38041958041958}, {"X"=1011.4225352112675, "Y"=138.38601398601406}, {"X"=1010.4211267605632, "Y"=139.38881118881125}, {"X"=1008.4183098591546, "Y"=140.39160839160843}, {"X"=1005.414084507042, "Y"=141.3944055944056}, {"X"=1002.4098591549294, "Y"=142.3972027972028}, {"X"=1000.4070422535209, "Y"=143.39999999999998}, {"X"=996.401408450704, "Y"=144.40279720279727}, {"X"=992.3957746478872, "Y"=146.40839160839164}, {"X"=990.3929577464786, "Y"=146.40839160839164}, {"X"=988.3901408450703, "Y"=147.41118881118882}, {"X"=987.388732394366, "Y"=148.413986013986}, {"X"=986.3873239436617, "Y"=148.413986013986}, {"X"=985.3859154929575, "Y"=148.413986013986}, {"X"=985.3859154929575, "Y"=149.4167832167833}, {"X"=986.3873239436617, "Y"=149.4167832167833}, {"X"=987.388732394366, "Y"=149.4167832167833}, {"X"=987.388732394366, "Y"=150.41958041958048}, {"X"=989.3915492957743, "Y"=150.41958041958048}, {"X"=990.3929577464786, "Y"=152.42517482517485}, {"X"=992.3957746478872, "Y"=153.42797202797203}, {"X"=994.3985915492955, "Y"=154.43076923076922}, {"X"=998.4042253521123, "Y"=157.43916083916088}, {"X"=999.4056338028166, "Y"=158.44195804195806}, {"X"=1000.4070422535209, "Y"=159.44475524475524}, {"X"=1002.4098591549294, "Y"=160.44755244755243}, {"X"=1004.4126760563378, "Y"=161.45034965034972}, {"X"=1005.414084507042, "Y"=162.4531468531469}, {"X"=1009.4197183098589, "Y"=163.4559440559441}, {"X"=1010.4211267605632, "Y"=164.45874125874127}, {"X"=1012.4239436619715, "Y"=165.46153846153845}, {"X"=1013.4253521126758, "Y"=167.46713286713293}, {"X"=1014.4267605633801, "Y"=167.46713286713293}, {"X"=1014.4267605633801, "Y"=168.46993006993011}, {"X"=1015.4281690140843, "Y"=168.46993006993011}, {"X"=1015.4281690140843, "Y"=169.4727272727273}, {"X"=1016.4295774647884, "Y"=169.4727272727273}, {"X"=1017.4309859154927, "Y"=169.4727272727273}, {"X"=1017.4309859154927, "Y"=170.47552447552448}, {"X"=1017.4309859154927, "Y"=169.4727272727273}, {"X"=1017.4309859154927, "Y"=170.47552447552448}, {"X"=1015.4281690140843, "Y"=169.4727272727273}, {"X"=1011.4225352112675, "Y"=167.46713286713293}, {"X"=1008.4183098591546, "Y"=165.46153846153845}, {"X"=1006.4154929577463, "Y"=164.45874125874127}, {"X"=1002.4098591549294, "Y"=162.4531468531469}, {"X"=998.4042253521123, "Y"=161.45034965034972}, {"X"=995.3999999999997, "Y"=159.44475524475524}, {"X"=992.3957746478872, "Y"=157.43916083916088}, {"X"=991.3943661971829, "Y"=156.4363636363637}, {"X"=990.3929577464786, "Y"=155.4335664335665}, {"X"=989.3915492957743, "Y"=155.4335664335665}, {"X"=988.3901408450703, "Y"=154.43076923076922}, {"X"=987.388732394366, "Y"=153.42797202797203}, {"X"=986.3873239436617, "Y"=152.42517482517485}, {"X"=986.3873239436617, "Y"=151.42237762237767}, {"X"=985.3859154929575, "Y"=151.42237762237767}, {"X"=985.3859154929575, "Y"=150.41958041958048}, {"X"=986.3873239436617, "Y"=150.41958041958048}, {"X"=986.3873239436617, "Y"=149.4167832167833}, {"X"=986.3873239436617, "Y"=148.413986013986}, {"X"=987.388732394366, "Y"=148.413986013986}, {"X"=987.388732394366, "Y"=147.41118881118882}, {"X"=987.388732394366, "Y"=146.40839160839164}, {"X"=987.388732394366, "Y"=145.40559440559446}, {"X"=987.388732394366, "Y"=144.40279720279727}, {"X"=988.3901408450703, "Y"=143.39999999999998}, {"X"=988.3901408450703, "Y"=142.3972027972028}, {"X"=988.3901408450703, "Y"=141.3944055944056}, {"X"=988.3901408450703, "Y"=140.39160839160843}, {"X"=989.3915492957743, "Y"=139.38881118881125}, {"X"=989.3915492957743, "Y"=138.38601398601406}, {"X"=989.3915492957743, "Y"=138.38601398601406}, {"X"=988.3901408450703, "Y"=139.38881118881125}, {"X"=986.3873239436617, "Y"=141.3944055944056}, {"X"=984.3845070422532, "Y"=145.40559440559446}, {"X"=982.3816901408449, "Y"=149.4167832167833}, {"X"=980.3788732394363, "Y"=152.42517482517485}, {"X"=978.376056338028, "Y"=157.43916083916088}, {"X"=976.3732394366194, "Y"=159.44475524475524}, {"X"=975.3718309859152, "Y"=161.45034965034972}, {"X"=975.3718309859152, "Y"=162.4531468531469}, {"X"=974.3704225352111, "Y"=163.4559440559441}, {"X"=973.3690140845068, "Y"=163.4559440559441}, {"X"=973.3690140845068, "Y"=164.45874125874127}, {"X"=973.3690140845068, "Y"=165.46153846153845}, {"X"=972.3676056338026, "Y"=165.46153846153845}, {"X"=972.3676056338026, "Y"=166.46433566433564}, {"X"=972.3676056338026, "Y"=167.46713286713293}, {"X"=971.3661971830983, "Y"=168.46993006993011}, {"X"=972.3676056338026, "Y"=168.46993006993011}, {"X"=971.3661971830983, "Y"=167.46713286713293}, {"X"=45.063380281690115, "Y"=385.0741258741259}, {"X"=48.0676056338028, "Y"=383.0685314685315}, {"X"=49.06901408450702, "Y"=382.0657342657343}, {"X"=51.07183098591547, "Y"=380.0601398601399}, {"X"=52.0732394366197, "Y"=379.0573426573427}, {"X"=56.078873239436604, "Y"=376.04895104895104}, {"X"=62.08732394366194, "Y"=370.03216783216783}, {"X"=64.09014084507041, "Y"=368.02657342657346}, {"X"=67.09436619718306, "Y"=365.01818181818186}, {"X"=70.09859154929575, "Y"=362.00979020979025}, {"X"=72.10140845070418, "Y"=360.00419580419583}, {"X"=75.10563380281687, "Y"=356.9958041958042}, {"X"=78.10985915492955, "Y"=354.9902097902098}, {"X"=80.11267605633799, "Y"=351.9818181818182}, {"X"=82.11549295774645, "Y"=349.9762237762238}, {"X"=86.12112676056336, "Y"=346.96783216783217}, {"X"=89.12535211267601, "Y"=343.95944055944057}, {"X"=90.12676056338026, "Y"=341.9538461538462}, {"X"=93.13098591549291, "Y"=338.94545454545454}, {"X"=96.1352112676056, "Y"=336.9398601398602}, {"X"=98.13802816901406, "Y"=333.93146853146857}, {"X"=100.1408450704225, "Y"=330.92307692307696}, {"X"=102.14366197183094, "Y"=327.91468531468536}, {"X"=103.14507042253518, "Y"=325.90909090909093}, {"X"=106.14929577464784, "Y"=321.8979020979021}, {"X"=108.1521126760563, "Y"=318.8895104895105}, {"X"=109.15352112676052, "Y"=317.8867132867133}, {"X"=110.15492957746474, "Y"=315.8811188811189}, {"X"=111.15633802816899, "Y"=314.8783216783217}, {"X"=113.15915492957743, "Y"=312.8727272727273}, {"X"=114.16056338028164, "Y"=311.8699300699301}, {"X"=115.16197183098589, "Y"=309.86433566433567}, {"X"=116.16338028169011, "Y"=309.86433566433567}, {"X"=117.16478873239433, "Y"=308.8615384615385}, {"X"=117.16478873239433, "Y"=307.8587412587413}, {"X"=118.16619718309855, "Y"=307.8587412587413}, {"X"=119.16760563380276, "Y"=306.85594405594406}, {"X"=120.16901408450701, "Y"=305.8531468531469}, {"X"=121.17042253521123, "Y"=304.8503496503497}, {"X"=122.17183098591545, "Y"=304.8503496503497}, {"X"=122.17183098591545, "Y"=303.84755244755246}, {"X"=123.17323943661967, "Y"=303.84755244755246}, {"X"=123.17323943661967, "Y"=304.8503496503497}, {"X"=123.17323943661967, "Y"=305.8531468531469}, {"X"=123.17323943661967, "Y"=307.8587412587413}, {"X"=122.17183098591545, "Y"=307.8587412587413}, {"X"=121.17042253521123, "Y"=310.8671328671329}, {"X"=120.16901408450701, "Y"=313.8755244755245}, {"X"=119.16760563380276, "Y"=315.8811188811189}, {"X"=118.16619718309855, "Y"=318.8895104895105}, {"X"=117.16478873239433, "Y"=324.90629370629375}, {"X"=116.16338028169011, "Y"=329.9202797202797}, {"X"=115.16197183098589, "Y"=333.93146853146857}, {"X"=114.16056338028164, "Y"=337.94265734265736}, {"X"=113.15915492957743, "Y"=341.9538461538462}, {"X"=112.15774647887321, "Y"=345.965034965035}, {"X"=110.15492957746474, "Y"=349.9762237762238}, {"X"=109.15352112676052, "Y"=352.9846153846154}, {"X"=108.1521126760563, "Y"=355.993006993007}, {"X"=106.14929577464784, "Y"=359.0013986013986}, {"X"=105.14788732394362, "Y"=362.00979020979025}, {"X"=104.1464788732394, "Y"=364.0153846153846}, {"X"=103.14507042253518, "Y"=367.0237762237762}, {"X"=102.14366197183094, "Y"=369.02937062937065}, {"X"=101.14225352112672, "Y"=371.03496503496507}, {"X"=100.1408450704225, "Y"=374.0433566433567}, {"X"=99.13943661971828, "Y"=376.04895104895104}, {"X"=99.13943661971828, "Y"=378.05454545454546}, {"X"=98.13802816901406, "Y"=381.06293706293707}, {"X"=98.13802816901406, "Y"=382.0657342657343}, {"X"=97.13661971830982, "Y"=382.0657342657343}, {"X"=97.13661971830982, "Y"=383.0685314685315}, {"X"=97.13661971830982, "Y"=384.0713286713287}, {"X"=96.1352112676056, "Y"=386.0769230769231}, {"X"=96.1352112676056, "Y"=387.0797202797203}, {"X"=95.13380281690138, "Y"=388.0825174825175}, {"X"=95.13380281690138, "Y"=389.0853146853147}, {"X"=95.13380281690138, "Y"=390.0881118881119}, {"X"=95.13380281690138, "Y"=389.0853146853147}, {"X"=95.13380281690138, "Y"=388.0825174825175}, {"X"=97.13661971830982, "Y"=385.0741258741259}, {"X"=98.13802816901406, "Y"=381.06293706293707}, {"X"=100.1408450704225, "Y"=376.04895104895104}, {"X"=101.14225352112672, "Y"=372.03776223776225}, {"X"=103.14507042253518, "Y"=368.02657342657346}, {"X"=105.14788732394362, "Y"=364.0153846153846}, {"X"=108.1521126760563, "Y"=359.0013986013986}, {"X"=109.15352112676052, "Y"=356.9958041958042}, {"X"=109.15352112676052, "Y"=355.993006993007}, {"X"=110.15492957746474, "Y"=353.9874125874126}, {"X"=110.15492957746474, "Y"=351.9818181818182}, {"X"=110.15492957746474, "Y"=350.979020979021}, {"X"=108.1521126760563, "Y"=351.9818181818182}, {"X"=105.14788732394362, "Y"=352.9846153846154}, {"X"=102.14366197183094, "Y"=353.9874125874126}, {"X"=98.13802816901406, "Y"=354.9902097902098}, {"X"=93.13098591549291, "Y"=355.993006993007}, {"X"=86.12112676056336, "Y"=357.9986013986014}, {"X"=82.11549295774645, "Y"=359.0013986013986}, {"X"=79.11126760563377, "Y"=359.0013986013986}, {"X"=77.10845070422533, "Y"=359.0013986013986}, {"X"=76.10704225352109, "Y"=360.00419580419583}, {"X"=75.10563380281687, "Y"=360.00419580419583}, {"X"=74.10422535211265, "Y"=360.00419580419583}, {"X"=72.10140845070418, "Y"=360.00419580419583}, {"X"=71.09999999999997, "Y"=361.006993006993}, {"X"=70.09859154929575, "Y"=362.00979020979025}, {"X"=72.10140845070418, "Y"=362.00979020979025}, {"X"=74.10422535211265, "Y"=361.006993006993}, {"X"=78.10985915492955, "Y"=361.006993006993}, {"X"=88.1239436619718, "Y"=359.0013986013986}, {"X"=93.13098591549291, "Y"=356.9958041958042}, {"X"=97.13661971830982, "Y"=355.993006993007}, {"X"=103.14507042253518, "Y"=352.9846153846154}, {"X"=106.14929577464784, "Y"=351.9818181818182}, {"X"=109.15352112676052, "Y"=350.979020979021}, {"X"=111.15633802816899, "Y"=349.9762237762238}, {"X"=112.15774647887321, "Y"=349.9762237762238}, {"X"=113.15915492957743, "Y"=349.9762237762238}, {"X"=114.16056338028164, "Y"=349.9762237762238}, {"X"=115.16197183098589, "Y"=349.9762237762238}, {"X"=115.16197183098589, "Y"=350.979020979021}, {"X"=114.16056338028164, "Y"=350.979020979021}, {"X"=113.15915492957743, "Y"=350.979020979021}, {"X"=153.21549295774642, "Y"=327.91468531468536}, {"X"=152.2140845070422, "Y"=331.92587412587415}, {"X"=151.21267605633798, "Y"=333.93146853146857}, {"X"=150.21126760563376, "Y"=334.93426573426575}, {"X"=149.20985915492952, "Y"=336.9398601398602}, {"X"=148.2084507042253, "Y"=339.9482517482518}, {"X"=146.20563380281686, "Y"=344.9622377622378}, {"X"=144.2028169014084, "Y"=348.9734265734266}, {"X"=143.20140845070418, "Y"=349.9762237762238}, {"X"=142.19999999999996, "Y"=351.9818181818182}, {"X"=140.1971830985915, "Y"=354.9902097902098}, {"X"=138.19436619718306, "Y"=356.9958041958042}, {"X"=137.19295774647884, "Y"=359.0013986013986}, {"X"=135.19014084507037, "Y"=362.00979020979025}, {"X"=134.18873239436616, "Y"=365.01818181818186}, {"X"=132.18591549295772, "Y"=367.0237762237762}, {"X"=132.18591549295772, "Y"=368.02657342657346}, {"X"=131.18450704225347, "Y"=369.02937062937065}, {"X"=131.18450704225347, "Y"=370.03216783216783}, {"X"=130.18309859154925, "Y"=372.03776223776225}, {"X"=129.18169014084503, "Y"=374.0433566433567}, {"X"=129.18169014084503, "Y"=376.04895104895104}, {"X"=128.18028169014082, "Y"=377.0517482517483}, {"X"=128.18028169014082, "Y"=378.05454545454546}, {"X"=128.18028169014082, "Y"=379.0573426573427}, {"X"=128.18028169014082, "Y"=378.05454545454546}, {"X"=128.18028169014082, "Y"=377.0517482517483}, {"X"=129.18169014084503, "Y"=377.0517482517483}, {"X"=129.18169014084503, "Y"=375.04615384615386}, {"X"=129.18169014084503, "Y"=374.0433566433567}, {"X"=130.18309859154925, "Y"=372.03776223776225}, {"X"=132.18591549295772, "Y"=369.02937062937065}, {"X"=134.18873239436616, "Y"=365.01818181818186}, {"X"=136.1915492957746, "Y"=362.00979020979025}, {"X"=139.19577464788728, "Y"=359.0013986013986}, {"X"=143.20140845070418, "Y"=354.9902097902098}, {"X"=145.20422535211264, "Y"=352.9846153846154}, {"X"=149.20985915492952, "Y"=348.9734265734266}, {"X"=152.2140845070422, "Y"=345.965034965035}, {"X"=156.2197183098591, "Y"=339.9482517482518}, {"X"=159.2239436619718, "Y"=335.93706293706293}, {"X"=162.22816901408447, "Y"=331.92587412587415}, {"X"=164.2309859154929, "Y"=329.9202797202797}, {"X"=168.2366197183098, "Y"=325.90909090909093}, {"X"=172.2422535211267, "Y"=320.8951048951049}, {"X"=172.2422535211267, "Y"=319.8923076923077}, {"X"=175.2464788732394, "Y"=317.8867132867133}, {"X"=178.25070422535205, "Y"=315.8811188811189}, {"X"=179.2521126760563, "Y"=314.8783216783217}, {"X"=180.25352112676052, "Y"=313.8755244755245}, {"X"=181.25492957746474, "Y"=313.8755244755245}, {"X"=182.25633802816895, "Y"=313.8755244755245}, {"X"=183.25774647887317, "Y"=312.8727272727273}, {"X"=184.2591549295774, "Y"=311.8699300699301}, {"X"=185.2605633802816, "Y"=312.8727272727273}, {"X"=186.26197183098589, "Y"=313.8755244755245}, {"X"=186.26197183098589, "Y"=315.8811188811189}, {"X"=186.26197183098589, "Y"=316.8839160839161}, {"X"=185.2605633802816, "Y"=322.90069930069933}, {"X"=184.2591549295774, "Y"=326.9118881118881}, {"X"=184.2591549295774, "Y"=329.9202797202797}, {"X"=182.25633802816895, "Y"=334.93426573426575}, {"X"=180.25352112676052, "Y"=339.9482517482518}, {"X"=178.25070422535205, "Y"=343.95944055944057}, {"X"=176.24788732394362, "Y"=348.9734265734266}, {"X"=175.2464788732394, "Y"=351.9818181818182}, {"X"=174.24507042253515, "Y"=354.9902097902098}, {"X"=172.2422535211267, "Y"=357.9986013986014}, {"X"=171.2408450704225, "Y"=360.00419580419583}, {"X"=170.23943661971825, "Y"=362.00979020979025}, {"X"=169.23802816901403, "Y"=363.01258741258744}, {"X"=168.2366197183098, "Y"=366.02097902097904}, {"X"=166.23380281690135, "Y"=368.02657342657346}, {"X"=165.23239436619713, "Y"=370.03216783216783}, {"X"=165.23239436619713, "Y"=371.03496503496507}, {"X"=164.2309859154929, "Y"=372.03776223776225}, {"X"=164.2309859154929, "Y"=373.04055944055943}, {"X"=163.2295774647887, "Y"=374.0433566433567}, {"X"=163.2295774647887, "Y"=375.04615384615386}, {"X"=162.22816901408447, "Y"=376.04895104895104}, {"X"=162.22816901408447, "Y"=377.0517482517483}, {"X"=162.22816901408447, "Y"=377.0517482517483}, {"X"=163.2295774647887, "Y"=374.0433566433567}, {"X"=163.2295774647887, "Y"=373.04055944055943}, {"X"=163.2295774647887, "Y"=372.03776223776225}, {"X"=164.2309859154929, "Y"=372.03776223776225}, {"X"=164.2309859154929, "Y"=371.03496503496507}, {"X"=164.2309859154929, "Y"=370.03216783216783}, {"X"=165.23239436619713, "Y"=370.03216783216783}, {"X"=165.23239436619713, "Y"=369.02937062937065}, {"X"=167.2352112676056, "Y"=368.02657342657346}, {"X"=170.23943661971825, "Y"=364.0153846153846}, {"X"=173.24366197183093, "Y"=360.00419580419583}, {"X"=177.24929577464783, "Y"=354.9902097902098}, {"X"=181.25492957746474, "Y"=350.979020979021}, {"X"=185.2605633802816, "Y"=345.965034965035}, {"X"=189.26619718309854, "Y"=340.95104895104896}, {"X"=193.27183098591541, "Y"=336.9398601398602}, {"X"=198.27887323943656, "Y"=332.9286713286713}, {"X"=201.28309859154922, "Y"=329.9202797202797}, {"X"=203.2859154929577, "Y"=327.91468531468536}, {"X"=205.28873239436615, "Y"=325.90909090909093}, {"X"=206.29014084507037, "Y"=324.90629370629375}, {"X"=207.2915492957746, "Y"=323.9034965034965}, {"X"=208.2929577464788, "Y"=322.90069930069933}, {"X"=208.2929577464788, "Y"=321.8979020979021}, {"X"=209.29436619718302, "Y"=321.8979020979021}, {"X"=210.29577464788724, "Y"=321.8979020979021}, {"X"=211.29718309859152, "Y"=321.8979020979021}, {"X"=212.29859154929574, "Y"=322.90069930069933}, {"X"=212.29859154929574, "Y"=323.9034965034965}, {"X"=212.29859154929574, "Y"=325.90909090909093}, {"X"=212.29859154929574, "Y"=327.91468531468536}, {"X"=211.29718309859152, "Y"=331.92587412587415}, {"X"=211.29718309859152, "Y"=333.93146853146857}, {"X"=211.29718309859152, "Y"=336.9398601398602}, {"X"=209.29436619718302, "Y"=340.95104895104896}, {"X"=208.2929577464788, "Y"=344.9622377622378}, {"X"=207.2915492957746, "Y"=348.9734265734266}, {"X"=206.29014084507037, "Y"=350.979020979021}, {"X"=205.28873239436615, "Y"=352.9846153846154}, {"X"=203.2859154929577, "Y"=355.993006993007}, {"X"=201.28309859154922, "Y"=359.0013986013986}, {"X"=200.281690140845, "Y"=362.00979020979025}, {"X"=197.27746478873235, "Y"=366.02097902097904}, {"X"=195.2746478873239, "Y"=369.02937062937065}, {"X"=194.2732394366197, "Y"=371.03496503496507}, {"X"=192.2704225352112, "Y"=374.0433566433567}, {"X"=191.26901408450698, "Y"=375.04615384615386}, {"X"=191.26901408450698, "Y"=377.0517482517483}, {"X"=189.26619718309854, "Y"=381.06293706293707}, {"X"=189.26619718309854, "Y"=383.0685314685315}, {"X"=188.26478873239432, "Y"=384.0713286713287}, {"X"=188.26478873239432, "Y"=385.0741258741259}, {"X"=188.26478873239432, "Y"=386.0769230769231}, {"X"=187.2633802816901, "Y"=387.0797202797203}, {"X"=187.2633802816901, "Y"=388.0825174825175}, {"X"=187.2633802816901, "Y"=387.0797202797203}, {"X"=187.2633802816901, "Y"=386.0769230769231}, {"X"=239.3366197183098, "Y"=325.90909090909093}, {"X"=238.3352112676056, "Y"=326.9118881118881}, {"X"=238.3352112676056, "Y"=328.91748251748254}, {"X"=238.3352112676056, "Y"=329.9202797202797}, {"X"=238.3352112676056, "Y"=330.92307692307696}, {"X"=238.3352112676056, "Y"=331.92587412587415}, {"X"=238.3352112676056, "Y"=332.9286713286713}, {"X"=238.3352112676056, "Y"=333.93146853146857}, {"X"=237.33380281690137, "Y"=333.93146853146857}, {"X"=237.33380281690137, "Y"=334.93426573426575}, {"X"=237.33380281690137, "Y"=335.93706293706293}, {"X"=237.33380281690137, "Y"=336.9398601398602}, {"X"=237.33380281690137, "Y"=337.94265734265736}, {"X"=236.3323943661971, "Y"=338.94545454545454}, {"X"=236.3323943661971, "Y"=339.9482517482518}, {"X"=236.3323943661971, "Y"=340.95104895104896}, {"X"=236.3323943661971, "Y"=341.9538461538462}, {"X"=235.33098591549287, "Y"=342.9566433566434}, {"X"=235.33098591549287, "Y"=343.95944055944057}, {"X"=235.33098591549287, "Y"=344.9622377622378}, {"X"=234.32957746478866, "Y"=345.965034965035}, {"X"=234.32957746478866, "Y"=347.9706293706294}, {"X"=233.32816901408444, "Y"=348.9734265734266}, {"X"=233.32816901408444, "Y"=350.979020979021}, {"X"=232.32676056338022, "Y"=352.9846153846154}, {"X"=232.32676056338022, "Y"=354.9902097902098}, {"X"=231.325352112676, "Y"=355.993006993007}, {"X"=230.32394366197178, "Y"=356.9958041958042}, {"X"=230.32394366197178, "Y"=357.9986013986014}, {"X"=230.32394366197178, "Y"=359.0013986013986}, {"X"=229.32253521126756, "Y"=361.006993006993}, {"X"=228.32112676056335, "Y"=362.00979020979025}, {"X"=228.32112676056335, "Y"=363.01258741258744}, {"X"=227.31971830985907, "Y"=364.0153846153846}, {"X"=227.31971830985907, "Y"=365.01818181818186}, {"X"=227.31971830985907, "Y"=366.02097902097904}, {"X"=227.31971830985907, "Y"=367.0237762237762}, {"X"=226.31830985915485, "Y"=367.0237762237762}, {"X"=226.31830985915485, "Y"=368.02657342657346}, {"X"=226.31830985915485, "Y"=369.02937062937065}, {"X"=226.31830985915485, "Y"=370.03216783216783}, {"X"=226.31830985915485, "Y"=371.03496503496507}, {"X"=225.31690140845063, "Y"=371.03496503496507}, {"X"=225.31690140845063, "Y"=372.03776223776225}, {"X"=225.31690140845063, "Y"=371.03496503496507}, {"X"=231.325352112676, "Y"=324.90629370629375}, {"X"=230.32394366197178, "Y"=324.90629370629375}, {"X"=231.325352112676, "Y"=324.90629370629375}, {"X"=231.325352112676, "Y"=323.9034965034965}, {"X"=232.32676056338022, "Y"=323.9034965034965}, {"X"=232.32676056338022, "Y"=322.90069930069933}, {"X"=233.32816901408444, "Y"=321.8979020979021}, {"X"=233.32816901408444, "Y"=320.8951048951049}, {"X"=234.32957746478866, "Y"=320.8951048951049}, {"X"=234.32957746478866, "Y"=319.8923076923077}, {"X"=235.33098591549287, "Y"=319.8923076923077}, {"X"=235.33098591549287, "Y"=318.8895104895105}, {"X"=236.3323943661971, "Y"=318.8895104895105}, {"X"=236.3323943661971, "Y"=317.8867132867133}, {"X"=237.33380281690137, "Y"=316.8839160839161}, {"X"=238.3352112676056, "Y"=316.8839160839161}, {"X"=239.3366197183098, "Y"=315.8811188811189}, {"X"=240.33802816901402, "Y"=315.8811188811189}, {"X"=240.33802816901402, "Y"=314.8783216783217}, {"X"=241.33943661971824, "Y"=314.8783216783217}, {"X"=242.34084507042246, "Y"=313.8755244755245}, {"X"=243.34225352112668, "Y"=313.8755244755245}, {"X"=244.3436619718309, "Y"=313.8755244755245}, {"X"=245.34507042253517, "Y"=312.8727272727273}, {"X"=247.3478873239436, "Y"=312.8727272727273}, {"X"=248.34929577464783, "Y"=311.8699300699301}, {"X"=249.35070422535205, "Y"=311.8699300699301}, {"X"=250.35211267605627, "Y"=311.8699300699301}, {"X"=252.3549295774647, "Y"=311.8699300699301}, {"X"=255.35915492957741, "Y"=310.8671328671329}, {"X"=256.36056338028163, "Y"=310.8671328671329}, {"X"=258.36338028169007, "Y"=310.8671328671329}, {"X"=259.3647887323943, "Y"=310.8671328671329}, {"X"=261.3676056338027, "Y"=310.8671328671329}, {"X"=262.36901408450694, "Y"=310.8671328671329}, {"X"=263.3704225352112, "Y"=310.8671328671329}, {"X"=264.37183098591544, "Y"=310.8671328671329}, {"X"=265.37323943661966, "Y"=310.8671328671329}, {"X"=266.3746478873239, "Y"=310.8671328671329}, {"X"=267.3760563380281, "Y"=310.8671328671329}, {"X"=267.3760563380281, "Y"=311.8699300699301}, {"X"=268.3774647887323, "Y"=311.8699300699301}, {"X"=269.37887323943653, "Y"=311.8699300699301}, {"X"=270.38028169014075, "Y"=312.8727272727273}, {"X"=270.38028169014075, "Y"=313.8755244755245}, {"X"=271.381690140845, "Y"=313.8755244755245}, {"X"=271.381690140845, "Y"=314.8783216783217}, {"X"=271.381690140845, "Y"=316.8839160839161}, {"X"=269.37887323943653, "Y"=318.8895104895105}, {"X"=268.3774647887323, "Y"=319.8923076923077}, {"X"=266.3746478873239, "Y"=322.90069930069933}, {"X"=264.37183098591544, "Y"=324.90629370629375}, {"X"=260.3661971830985, "Y"=326.9118881118881}, {"X"=258.36338028169007, "Y"=328.91748251748254}, {"X"=255.35915492957741, "Y"=330.92307692307696}, {"X"=252.3549295774647, "Y"=332.9286713286713}, {"X"=251.35352112676048, "Y"=332.9286713286713}, {"X"=250.35211267605627, "Y"=333.93146853146857}, {"X"=249.35070422535205, "Y"=333.93146853146857}, {"X"=247.3478873239436, "Y"=335.93706293706293}, {"X"=246.3464788732394, "Y"=336.9398601398602}, {"X"=245.34507042253517, "Y"=337.94265734265736}, {"X"=244.3436619718309, "Y"=337.94265734265736}, {"X"=243.34225352112668, "Y"=338.94545454545454}, {"X"=242.34084507042246, "Y"=338.94545454545454}, {"X"=243.34225352112668, "Y"=338.94545454545454}, {"X"=244.3436619718309, "Y"=338.94545454545454}, {"X"=245.34507042253517, "Y"=338.94545454545454}, {"X"=248.34929577464783, "Y"=338.94545454545454}, {"X"=250.35211267605627, "Y"=338.94545454545454}, {"X"=252.3549295774647, "Y"=338.94545454545454}, {"X"=254.3577464788732, "Y"=338.94545454545454}, {"X"=256.36056338028163, "Y"=339.9482517482518}, {"X"=258.36338028169007, "Y"=340.95104895104896}, {"X"=259.3647887323943, "Y"=341.9538461538462}, {"X"=260.3661971830985, "Y"=343.95944055944057}, {"X"=263.3704225352112, "Y"=345.965034965035}, {"X"=264.37183098591544, "Y"=346.96783216783217}, {"X"=265.37323943661966, "Y"=347.9706293706294}, {"X"=266.3746478873239, "Y"=347.9706293706294}, {"X"=268.3774647887323, "Y"=349.9762237762238}, {"X"=269.37887323943653, "Y"=350.979020979021}, {"X"=270.38028169014075, "Y"=350.979020979021}, {"X"=270.38028169014075, "Y"=351.9818181818182}, {"X"=271.381690140845, "Y"=351.9818181818182}, {"X"=272.38309859154924, "Y"=352.9846153846154}, {"X"=273.38450704225346, "Y"=353.9874125874126}, {"X"=274.3859154929577, "Y"=353.9874125874126}, {"X"=274.3859154929577, "Y"=354.9902097902098}, {"X"=275.3873239436619, "Y"=354.9902097902098}, {"X"=275.3873239436619, "Y"=355.993006993007}, {"X"=275.3873239436619, "Y"=356.9958041958042}, {"X"=275.3873239436619, "Y"=357.9986013986014}, {"X"=274.3859154929577, "Y"=359.0013986013986}, {"X"=274.3859154929577, "Y"=360.00419580419583}, {"X"=273.38450704225346, "Y"=361.006993006993}, {"X"=273.38450704225346, "Y"=362.00979020979025}, {"X"=273.38450704225346, "Y"=363.01258741258744}, {"X"=272.38309859154924, "Y"=364.0153846153846}, {"X"=271.381690140845, "Y"=365.01818181818186}, {"X"=269.37887323943653, "Y"=365.01818181818186}, {"X"=268.3774647887323, "Y"=367.0237762237762}, {"X"=267.3760563380281, "Y"=368.02657342657346}, {"X"=265.37323943661966, "Y"=368.02657342657346}, {"X"=264.37183098591544, "Y"=369.02937062937065}, {"X"=262.36901408450694, "Y"=369.02937062937065}, {"X"=259.3647887323943, "Y"=371.03496503496507}, {"X"=257.36197183098585, "Y"=372.03776223776225}, {"X"=255.35915492957741, "Y"=373.04055944055943}, {"X"=250.35211267605627, "Y"=375.04615384615386}, {"X"=248.34929577464783, "Y"=375.04615384615386}, {"X"=246.3464788732394, "Y"=376.04895104895104}, {"X"=243.34225352112668, "Y"=377.0517482517483}, {"X"=242.34084507042246, "Y"=377.0517482517483}, {"X"=241.33943661971824, "Y"=377.0517482517483}, {"X"=239.3366197183098, "Y"=377.0517482517483}, {"X"=235.33098591549287, "Y"=378.05454545454546}, {"X"=233.32816901408444, "Y"=379.0573426573427}, {"X"=231.325352112676, "Y"=379.0573426573427}, {"X"=229.32253521126756, "Y"=379.0573426573427}, {"X"=228.32112676056335, "Y"=379.0573426573427}, {"X"=227.31971830985907, "Y"=379.0573426573427}, {"X"=226.31830985915485, "Y"=380.0601398601399}, {"X"=225.31690140845063, "Y"=380.0601398601399}, {"X"=224.31549295774641, "Y"=380.0601398601399}, {"X"=223.3140845070422, "Y"=380.0601398601399}, {"X"=222.31267605633798, "Y"=381.06293706293707}, {"X"=222.31267605633798, "Y"=380.0601398601399}, {"X"=270.38028169014075, "Y"=371.03496503496507}, {"X"=269.37887323943653, "Y"=372.03776223776225}, {"X"=269.37887323943653, "Y"=371.03496503496507}, {"X"=270.38028169014075, "Y"=371.03496503496507}, {"X"=271.381690140845, "Y"=371.03496503496507}, {"X"=272.38309859154924, "Y"=371.03496503496507}, {"X"=274.3859154929577, "Y"=370.03216783216783}, {"X"=277.39014084507033, "Y"=369.02937062937065}, {"X"=281.39577464788727, "Y"=368.02657342657346}, {"X"=285.40140845070414, "Y"=367.0237762237762}, {"X"=290.4084507042253, "Y"=366.02097902097904}, {"X"=295.4154929577464, "Y"=365.01818181818186}, {"X"=298.4197183098591, "Y"=364.0153846153846}, {"X"=303.4267605633802, "Y"=363.01258741258744}, {"X"=309.43521126760555, "Y"=362.00979020979025}, {"X"=313.4408450704224, "Y"=362.00979020979025}, {"X"=316.44507042253514, "Y"=361.006993006993}, {"X"=320.450704225352, "Y"=360.00419580419583}, {"X"=322.4535211267605, "Y"=359.0013986013986}, {"X"=324.45633802816894, "Y"=359.0013986013986}, {"X"=325.45774647887316, "Y"=357.9986013986014}, {"X"=326.4591549295774, "Y"=357.9986013986014}, {"X"=327.4605633802816, "Y"=357.9986013986014}, {"X"=328.4619718309858, "Y"=356.9958041958042}, {"X"=329.46338028169004, "Y"=356.9958041958042}, {"X"=330.46478873239425, "Y"=356.9958041958042}, {"X"=329.46338028169004, "Y"=356.9958041958042}, {"X"=328.4619718309858, "Y"=356.9958041958042}, {"X"=327.4605633802816, "Y"=356.9958041958042}, {"X"=324.45633802816894, "Y"=356.9958041958042}, {"X"=323.4549295774647, "Y"=357.9986013986014}, {"X"=320.450704225352, "Y"=357.9986013986014}, {"X"=315.4436619718309, "Y"=360.00419580419583}, {"X"=309.43521126760555, "Y"=361.006993006993}, {"X"=305.4295774647887, "Y"=362.00979020979025}, {"X"=302.42535211267597, "Y"=363.01258741258744}, {"X"=300.42253521126753, "Y"=363.01258741258744}, {"X"=298.4197183098591, "Y"=364.0153846153846}, {"X"=297.4183098591549, "Y"=364.0153846153846}, {"X"=296.4169014084506, "Y"=364.0153846153846}, {"X"=295.4154929577464, "Y"=364.0153846153846}, {"X"=294.41408450704216, "Y"=365.01818181818186}, {"X"=293.41267605633794, "Y"=365.01818181818186}, {"X"=292.4112676056337, "Y"=365.01818181818186}, {"X"=291.4098591549295, "Y"=365.01818181818186}, {"X"=291.4098591549295, "Y"=364.0153846153846}, {"X"=291.4098591549295, "Y"=363.01258741258744}, {"X"=291.4098591549295, "Y"=362.00979020979025}, {"X"=293.41267605633794, "Y"=359.0013986013986}, {"X"=293.41267605633794, "Y"=356.9958041958042}, {"X"=294.41408450704216, "Y"=355.993006993007}, {"X"=294.41408450704216, "Y"=353.9874125874126}, {"X"=295.4154929577464, "Y"=351.9818181818182}, {"X"=296.4169014084506, "Y"=348.9734265734266}, {"X"=297.4183098591549, "Y"=345.965034965035}, {"X"=298.4197183098591, "Y"=343.95944055944057}, {"X"=298.4197183098591, "Y"=341.9538461538462}, {"X"=299.4211267605633, "Y"=339.9482517482518}, {"X"=300.42253521126753, "Y"=337.94265734265736}, {"X"=302.42535211267597, "Y"=334.93426573426575}, {"X"=304.4281690140844, "Y"=332.9286713286713}, {"X"=305.4295774647887, "Y"=329.9202797202797}, {"X"=306.4309859154929, "Y"=326.9118881118881}, {"X"=307.4323943661971, "Y"=325.90909090909093}, {"X"=307.4323943661971, "Y"=323.9034965034965}, {"X"=308.43380281690133, "Y"=322.90069930069933}, {"X"=308.43380281690133, "Y"=321.8979020979021}, {"X"=309.43521126760555, "Y"=319.8923076923077}, {"X"=310.43661971830977, "Y"=318.8895104895105}, {"X"=310.43661971830977, "Y"=317.8867132867133}, {"X"=311.438028169014, "Y"=316.8839160839161}, {"X"=310.43661971830977, "Y"=316.8839160839161}, {"X"=309.43521126760555, "Y"=316.8839160839161}, {"X"=308.43380281690133, "Y"=317.8867132867133}, {"X"=307.4323943661971, "Y"=317.8867132867133}, {"X"=306.4309859154929, "Y"=317.8867132867133}, {"X"=304.4281690140844, "Y"=318.8895104895105}, {"X"=301.42394366197175, "Y"=318.8895104895105}, {"X"=298.4197183098591, "Y"=320.8951048951049}, {"X"=294.41408450704216, "Y"=321.8979020979021}, {"X"=293.41267605633794, "Y"=322.90069930069933}, {"X"=291.4098591549295, "Y"=323.9034965034965}, {"X"=288.40563380281685, "Y"=323.9034965034965}, {"X"=287.4042253521126, "Y"=323.9034965034965}, {"X"=285.40140845070414, "Y"=323.9034965034965}, {"X"=283.3985915492957, "Y"=324.90629370629375}, {"X"=282.3971830985915, "Y"=324.90629370629375}, {"X"=280.39436619718305, "Y"=324.90629370629375}, {"X"=280.39436619718305, "Y"=324.90629370629375}, {"X"=282.3971830985915, "Y"=324.90629370629375}, {"X"=283.3985915492957, "Y"=324.90629370629375}, {"X"=289.40704225352107, "Y"=324.90629370629375}, {"X"=294.41408450704216, "Y"=322.90069930069933}, {"X"=300.42253521126753, "Y"=321.8979020979021}, {"X"=309.43521126760555, "Y"=319.8923076923077}, {"X"=317.44647887323936, "Y"=318.8895104895105}, {"X"=321.45211267605623, "Y"=317.8867132867133}, {"X"=325.45774647887316, "Y"=316.8839160839161}, {"X"=329.46338028169004, "Y"=315.8811188811189}, {"X"=331.46619718309853, "Y"=315.8811188811189}, {"X"=335.4718309859154, "Y"=314.8783216783217}, {"X"=339.47746478873233, "Y"=314.8783216783217}, {"X"=340.47887323943655, "Y"=314.8783216783217}, {"X"=341.48028169014077, "Y"=314.8783216783217}, {"X"=342.481690140845, "Y"=314.8783216783217}, {"X"=343.4830985915492, "Y"=314.8783216783217}, {"X"=344.4845070422534, "Y"=314.8783216783217}, {"X"=345.48591549295764, "Y"=314.8783216783217}, {"X"=345.48591549295764, "Y"=313.8755244755245}, {"X"=346.48732394366186, "Y"=313.8755244755245}, {"X"=346.48732394366186, "Y"=314.8783216783217}, {"X"=347.4887323943661, "Y"=314.8783216783217}, {"X"=348.49014084507036, "Y"=314.8783216783217}, {"X"=349.4915492957746, "Y"=313.8755244755245}, {"X"=350.4929577464788, "Y"=313.8755244755245}, {"X"=351.494366197183, "Y"=313.8755244755245}, {"X"=352.49577464788723, "Y"=313.8755244755245}, {"X"=353.49718309859145, "Y"=313.8755244755245}, {"X"=353.49718309859145, "Y"=314.8783216783217}, {"X"=353.49718309859145, "Y"=315.8811188811189}, {"X"=353.49718309859145, "Y"=316.8839160839161}, {"X"=353.49718309859145, "Y"=317.8867132867133}, {"X"=353.49718309859145, "Y"=319.8923076923077}, {"X"=353.49718309859145, "Y"=321.8979020979021}, {"X"=353.49718309859145, "Y"=322.90069930069933}, {"X"=353.49718309859145, "Y"=324.90629370629375}, {"X"=353.49718309859145, "Y"=326.9118881118881}, {"X"=353.49718309859145, "Y"=327.91468531468536}, {"X"=354.49859154929567, "Y"=327.91468531468536}, {"X"=355.4999999999999, "Y"=327.91468531468536}, {"X"=356.50140845070416, "Y"=327.91468531468536}, {"X"=357.5028169014084, "Y"=326.9118881118881}, {"X"=359.5056338028168, "Y"=325.90909090909093}, {"X"=361.50845070422525, "Y"=325.90909090909093}, {"X"=362.5098591549295, "Y"=324.90629370629375}, {"X"=363.5112676056337, "Y"=323.9034965034965}, {"X"=365.5140845070422, "Y"=322.90069930069933}, {"X"=366.5154929577464, "Y"=322.90069930069933}, {"X"=372.5239436619717, "Y"=320.8951048951049}, {"X"=375.5281690140844, "Y"=319.8923076923077}, {"X"=379.5338028169013, "Y"=318.8895104895105}, {"X"=384.54084507042245, "Y"=317.8867132867133}, {"X"=388.5464788732393, "Y"=316.8839160839161}, {"X"=389.54788732394354, "Y"=316.8839160839161}, {"X"=393.5535211267605, "Y"=315.8811188811189}, {"X"=394.5549295774647, "Y"=315.8811188811189}, {"X"=396.5577464788731, "Y"=314.8783216783217}, {"X"=397.55915492957735, "Y"=314.8783216783217}, {"X"=399.56197183098584, "Y"=314.8783216783217}, {"X"=401.5647887323943, "Y"=313.8755244755245}, {"X"=402.5661971830985, "Y"=313.8755244755245}, {"X"=403.5676056338027, "Y"=313.8755244755245}, {"X"=404.56901408450693, "Y"=313.8755244755245}, {"X"=403.5676056338027, "Y"=313.8755244755245}, {"X"=402.5661971830985, "Y"=314.8783216783217}, {"X"=401.5647887323943, "Y"=314.8783216783217}, {"X"=400.56338028169006, "Y"=314.8783216783217}, {"X"=398.56056338028156, "Y"=315.8811188811189}, {"X"=397.55915492957735, "Y"=316.8839160839161}, {"X"=396.5577464788731, "Y"=316.8839160839161}, {"X"=393.5535211267605, "Y"=316.8839160839161}, {"X"=392.55211267605625, "Y"=316.8839160839161}, {"X"=388.5464788732393, "Y"=317.8867132867133}, {"X"=387.5450704225351, "Y"=317.8867132867133}, {"X"=385.54225352112667, "Y"=317.8867132867133}, {"X"=383.53943661971823, "Y"=317.8867132867133}, {"X"=382.538028169014, "Y"=317.8867132867133}, {"X"=381.53661971830974, "Y"=317.8867132867133}, {"X"=381.53661971830974, "Y"=318.8895104895105}, {"X"=381.53661971830974, "Y"=317.8867132867133}, {"X"=382.538028169014, "Y"=317.8867132867133}, {"X"=383.53943661971823, "Y"=317.8867132867133}, {"X"=383.53943661971823, "Y"=316.8839160839161}, {"X"=384.54084507042245, "Y"=316.8839160839161}, {"X"=385.54225352112667, "Y"=316.8839160839161}, {"X"=384.54084507042245, "Y"=316.8839160839161}, {"X"=384.54084507042245, "Y"=317.8867132867133}, {"X"=383.53943661971823, "Y"=317.8867132867133}, {"X"=382.538028169014, "Y"=319.8923076923077}, {"X"=382.538028169014, "Y"=320.8951048951049}, {"X"=381.53661971830974, "Y"=322.90069930069933}, {"X"=379.5338028169013, "Y"=326.9118881118881}, {"X"=377.53098591549286, "Y"=328.91748251748254}, {"X"=375.5281690140844, "Y"=333.93146853146857}, {"X"=374.5267605633802, "Y"=335.93706293706293}, {"X"=372.5239436619717, "Y"=337.94265734265736}, {"X"=371.5225352112675, "Y"=340.95104895104896}, {"X"=368.51830985915484, "Y"=343.95944055944057}, {"X"=365.5140845070422, "Y"=347.9706293706294}, {"X"=363.5112676056337, "Y"=348.9734265734266}, {"X"=361.50845070422525, "Y"=351.9818181818182}, {"X"=359.5056338028168, "Y"=352.9846153846154}, {"X"=357.5028169014084, "Y"=354.9902097902098}, {"X"=356.50140845070416, "Y"=355.993006993007}, {"X"=355.4999999999999, "Y"=355.993006993007}, {"X"=355.4999999999999, "Y"=356.9958041958042}, {"X"=354.49859154929567, "Y"=357.9986013986014}, {"X"=353.49718309859145, "Y"=359.0013986013986}, {"X"=353.49718309859145, "Y"=360.00419580419583}, {"X"=352.49577464788723, "Y"=360.00419580419583}, {"X"=353.49718309859145, "Y"=360.00419580419583}, {"X"=352.49577464788723, "Y"=360.00419580419583}, {"X"=432.6084507042252, "Y"=316.8839160839161}, {"X"=435.61267605633793, "Y"=315.8811188811189}, {"X"=436.61408450704215, "Y"=315.8811188811189}, {"X"=438.61690140845064, "Y"=315.8811188811189}, {"X"=439.6183098591548, "Y"=314.8783216783217}, {"X"=440.6197183098591, "Y"=314.8783216783217}, {"X"=441.62112676056324, "Y"=314.8783216783217}, {"X"=443.6239436619717, "Y"=313.8755244755245}, {"X"=444.62535211267596, "Y"=313.8755244755245}, {"X"=446.6281690140844, "Y"=313.8755244755245}, {"X"=447.62957746478867, "Y"=313.8755244755245}, {"X"=449.6323943661971, "Y"=313.8755244755245}, {"X"=450.63380281690127, "Y"=312.8727272727273}, {"X"=452.6366197183097, "Y"=312.8727272727273}, {"X"=453.638028169014, "Y"=312.8727272727273}, {"X"=454.63943661971814, "Y"=312.8727272727273}, {"X"=455.6408450704224, "Y"=312.8727272727273}, {"X"=456.6422535211267, "Y"=312.8727272727273}, {"X"=457.64366197183085, "Y"=311.8699300699301}, {"X"=459.6464788732393, "Y"=311.8699300699301}, {"X"=460.64788732394356, "Y"=310.8671328671329}, {"X"=461.6492957746477, "Y"=310.8671328671329}, {"X"=463.6521126760563, "Y"=310.8671328671329}, {"X"=463.6521126760563, "Y"=309.86433566433567}, {"X"=464.65352112676044, "Y"=309.86433566433567}, {"X"=466.6563380281689, "Y"=309.86433566433567}, {"X"=468.6591549295773, "Y"=309.86433566433567}, {"X"=469.6605633802816, "Y"=309.86433566433567}, {"X"=470.66197183098575, "Y"=308.8615384615385}, {"X"=472.6647887323943, "Y"=308.8615384615385}, {"X"=473.66619718309846, "Y"=308.8615384615385}, {"X"=474.66760563380274, "Y"=308.8615384615385}, {"X"=475.6690140845069, "Y"=307.8587412587413}, {"X"=476.6704225352112, "Y"=307.8587412587413}, {"X"=477.67183098591534, "Y"=307.8587412587413}, {"X"=478.6732394366196, "Y"=307.8587412587413}, {"X"=479.6746478873238, "Y"=307.8587412587413}, {"X"=480.67605633802805, "Y"=307.8587412587413}, {"X"=481.6774647887323, "Y"=307.8587412587413}, {"X"=482.6788732394365, "Y"=307.8587412587413}, {"X"=483.68028169014076, "Y"=307.8587412587413}, {"X"=484.6816901408449, "Y"=307.8587412587413}, {"X"=485.6830985915492, "Y"=307.8587412587413}, {"X"=485.6830985915492, "Y"=306.85594405594406}, {"X"=486.68450704225336, "Y"=306.85594405594406}, {"X"=487.68591549295763, "Y"=306.85594405594406}, {"X"=486.68450704225336, "Y"=306.85594405594406}, {"X"=485.6830985915492, "Y"=306.85594405594406}, {"X"=484.6816901408449, "Y"=306.85594405594406}, {"X"=483.68028169014076, "Y"=307.8587412587413}, {"X"=482.6788732394365, "Y"=307.8587412587413}, {"X"=480.67605633802805, "Y"=307.8587412587413}, {"X"=479.6746478873238, "Y"=307.8587412587413}, {"X"=478.6732394366196, "Y"=307.8587412587413}, {"X"=472.6647887323943, "Y"=308.8615384615385}, {"X"=469.6605633802816, "Y"=308.8615384615385}, {"X"=464.65352112676044, "Y"=309.86433566433567}, {"X"=462.650704225352, "Y"=309.86433566433567}, {"X"=461.6492957746477, "Y"=310.8671328671329}, {"X"=460.64788732394356, "Y"=310.8671328671329}, {"X"=459.6464788732393, "Y"=310.8671328671329}, {"X"=458.6450704225351, "Y"=310.8671328671329}, {"X"=457.64366197183085, "Y"=310.8671328671329}, {"X"=456.6422535211267, "Y"=310.8671328671329}, {"X"=455.6408450704224, "Y"=310.8671328671329}, {"X"=454.63943661971814, "Y"=310.8671328671329}, {"X"=453.638028169014, "Y"=310.8671328671329}, {"X"=452.6366197183097, "Y"=311.8699300699301}, {"X"=452.6366197183097, "Y"=312.8727272727273}, {"X"=451.63521126760554, "Y"=313.8755244755245}, {"X"=451.63521126760554, "Y"=314.8783216783217}, {"X"=450.63380281690127, "Y"=314.8783216783217}, {"X"=450.63380281690127, "Y"=316.8839160839161}, {"X"=449.6323943661971, "Y"=317.8867132867133}, {"X"=449.6323943661971, "Y"=320.8951048951049}, {"X"=447.62957746478867, "Y"=324.90629370629375}, {"X"=446.6281690140844, "Y"=326.9118881118881}, {"X"=446.6281690140844, "Y"=329.9202797202797}, {"X"=445.6267605633801, "Y"=331.92587412587415}, {"X"=444.62535211267596, "Y"=335.93706293706293}, {"X"=443.6239436619717, "Y"=338.94545454545454}, {"X"=443.6239436619717, "Y"=339.9482517482518}, {"X"=441.62112676056324, "Y"=342.9566433566434}, {"X"=440.6197183098591, "Y"=344.9622377622378}, {"X"=440.6197183098591, "Y"=346.96783216783217}, {"X"=439.6183098591548, "Y"=347.9706293706294}, {"X"=439.6183098591548, "Y"=348.9734265734266}, {"X"=439.6183098591548, "Y"=349.9762237762238}, {"X"=439.6183098591548, "Y"=350.979020979021}, {"X"=438.61690140845064, "Y"=350.979020979021}, {"X"=438.61690140845064, "Y"=351.9818181818182}, {"X"=438.61690140845064, "Y"=352.9846153846154}, {"X"=438.61690140845064, "Y"=353.9874125874126}, {"X"=438.61690140845064, "Y"=354.9902097902098}, {"X"=437.61549295774637, "Y"=354.9902097902098}, {"X"=437.61549295774637, "Y"=355.993006993007}, {"X"=436.61408450704215, "Y"=355.993006993007}, {"X"=435.61267605633793, "Y"=355.993006993007}, {"X"=434.6112676056337, "Y"=354.9902097902098}, {"X"=433.6098591549295, "Y"=354.9902097902098}, {"X"=432.6084507042252, "Y"=355.993006993007}, {"X"=430.6056338028168, "Y"=355.993006993007}, {"X"=428.60281690140835, "Y"=355.993006993007}, {"X"=425.5985915492957, "Y"=356.9958041958042}, {"X"=422.594366197183, "Y"=356.9958041958042}, {"X"=418.5887323943661, "Y"=357.9986013986014}, {"X"=416.58591549295767, "Y"=357.9986013986014}, {"X"=411.5788732394365, "Y"=359.0013986013986}, {"X"=409.5760563380281, "Y"=359.0013986013986}, {"X"=408.57464788732386, "Y"=360.00419580419583}, {"X"=407.5732394366196, "Y"=360.00419580419583}, {"X"=406.57183098591537, "Y"=360.00419580419583}, {"X"=405.57042253521115, "Y"=360.00419580419583}, {"X"=404.56901408450693, "Y"=360.00419580419583}, {"X"=405.57042253521115, "Y"=360.00419580419583}, {"X"=406.57183098591537, "Y"=360.00419580419583}, {"X"=407.5732394366196, "Y"=360.00419580419583}, {"X"=410.5774647887323, "Y"=359.0013986013986}, {"X"=413.58169014084496, "Y"=357.9986013986014}, {"X"=416.58591549295767, "Y"=357.9986013986014}, {"X"=418.5887323943661, "Y"=356.9958041958042}, {"X"=427.6014084507041, "Y"=354.9902097902098}, {"X"=431.607042253521, "Y"=353.9874125874126}, {"X"=439.6183098591548, "Y"=351.9818181818182}, {"X"=445.6267605633801, "Y"=349.9762237762238}, {"X"=448.63098591549283, "Y"=348.9734265734266}, {"X"=454.63943661971814, "Y"=347.9706293706294}, {"X"=459.6464788732393, "Y"=345.965034965035}, {"X"=461.6492957746477, "Y"=345.965034965035}, {"X"=464.65352112676044, "Y"=344.9622377622378}, {"X"=467.65774647887315, "Y"=343.95944055944057}, {"X"=469.6605633802816, "Y"=343.95944055944057}, {"X"=470.66197183098575, "Y"=342.9566433566434}, {"X"=471.66338028169, "Y"=342.9566433566434}, {"X"=472.6647887323943, "Y"=342.9566433566434}, {"X"=473.66619718309846, "Y"=342.9566433566434}, {"X"=472.6647887323943, "Y"=342.9566433566434}, {"X"=471.66338028169, "Y"=342.9566433566434}, {"X"=471.66338028169, "Y"=341.9538461538462}, {"X"=470.66197183098575, "Y"=341.9538461538462}, {"X"=469.6605633802816, "Y"=341.9538461538462}, {"X"=468.6591549295773, "Y"=341.9538461538462}, {"X"=503.70845070422524, "Y"=311.8699300699301}, {"X"=502.70704225352097, "Y"=312.8727272727273}, {"X"=501.7056338028168, "Y"=313.8755244755245}, {"X"=500.70422535211253, "Y"=313.8755244755245}, {"X"=499.70281690140837, "Y"=314.8783216783217}, {"X"=498.7014084507041, "Y"=315.8811188811189}, {"X"=497.69999999999993, "Y"=315.8811188811189}, {"X"=497.69999999999993, "Y"=316.8839160839161}, {"X"=494.6957746478872, "Y"=318.8895104895105}, {"X"=493.69436619718294, "Y"=320.8951048951049}, {"X"=491.6915492957745, "Y"=321.8979020979021}, {"X"=491.6915492957745, "Y"=322.90069930069933}, {"X"=490.69014084507035, "Y"=324.90629370629375}, {"X"=488.6873239436618, "Y"=325.90909090909093}, {"X"=487.68591549295763, "Y"=328.91748251748254}, {"X"=487.68591549295763, "Y"=329.9202797202797}, {"X"=486.68450704225336, "Y"=331.92587412587415}, {"X"=485.6830985915492, "Y"=332.9286713286713}, {"X"=485.6830985915492, "Y"=333.93146853146857}, {"X"=484.6816901408449, "Y"=335.93706293706293}, {"X"=484.6816901408449, "Y"=336.9398601398602}, {"X"=483.68028169014076, "Y"=337.94265734265736}, {"X"=483.68028169014076, "Y"=338.94545454545454}, {"X"=483.68028169014076, "Y"=339.9482517482518}, {"X"=484.6816901408449, "Y"=340.95104895104896}, {"X"=484.6816901408449, "Y"=341.9538461538462}, {"X"=485.6830985915492, "Y"=343.95944055944057}, {"X"=486.68450704225336, "Y"=344.9622377622378}, {"X"=488.6873239436618, "Y"=345.965034965035}, {"X"=491.6915492957745, "Y"=346.96783216783217}, {"X"=494.6957746478872, "Y"=346.96783216783217}, {"X"=495.6971830985914, "Y"=346.96783216783217}, {"X"=499.70281690140837, "Y"=345.965034965035}, {"X"=502.70704225352097, "Y"=344.9622377622378}, {"X"=504.7098591549294, "Y"=343.95944055944057}, {"X"=509.71690140845055, "Y"=340.95104895104896}, {"X"=513.7225352112674, "Y"=337.94265734265736}, {"X"=517.7281690140844, "Y"=334.93426573426575}, {"X"=518.7295774647886, "Y"=333.93146853146857}, {"X"=521.7338028169013, "Y"=331.92587412587415}, {"X"=525.7394366197182, "Y"=328.91748251748254}, {"X"=526.7408450704224, "Y"=326.9118881118881}, {"X"=528.7436619718309, "Y"=324.90629370629375}, {"X"=529.745070422535, "Y"=322.90069930069933}, {"X"=530.7464788732393, "Y"=320.8951048951049}, {"X"=531.7478873239436, "Y"=317.8867132867133}, {"X"=531.7478873239436, "Y"=316.8839160839161}, {"X"=531.7478873239436, "Y"=315.8811188811189}, {"X"=530.7464788732393, "Y"=313.8755244755245}, {"X"=528.7436619718309, "Y"=311.8699300699301}, {"X"=527.7422535211266, "Y"=311.8699300699301}, {"X"=524.738028169014, "Y"=310.8671328671329}, {"X"=522.7352112676055, "Y"=309.86433566433567}, {"X"=520.732394366197, "Y"=309.86433566433567}, {"X"=519.7309859154929, "Y"=308.8615384615385}, {"X"=518.7295774647886, "Y"=308.8615384615385}, {"X"=516.7267605633801, "Y"=308.8615384615385}, {"X"=515.725352112676, "Y"=308.8615384615385}, {"X"=514.7239436619717, "Y"=308.8615384615385}, {"X"=513.7225352112674, "Y"=308.8615384615385}, {"X"=512.7211267605633, "Y"=308.8615384615385}, {"X"=511.719718309859, "Y"=308.8615384615385}, {"X"=510.71830985915483, "Y"=308.8615384615385}, {"X"=510.71830985915483, "Y"=309.86433566433567}, {"X"=509.71690140845055, "Y"=309.86433566433567}, {"X"=508.7154929577464, "Y"=309.86433566433567}, {"X"=507.7140845070421, "Y"=310.8671328671329}, {"X"=506.71267605633795, "Y"=310.8671328671329}, {"X"=540.7605633802816, "Y"=312.8727272727273}, {"X"=540.7605633802816, "Y"=313.8755244755245}, {"X"=539.7591549295773, "Y"=313.8755244755245}, {"X"=539.7591549295773, "Y"=314.8783216783217}, {"X"=538.7577464788731, "Y"=315.8811188811189}, {"X"=537.7563380281689, "Y"=316.8839160839161}, {"X"=537.7563380281689, "Y"=317.8867132867133}, {"X"=536.7549295774646, "Y"=317.8867132867133}, {"X"=536.7549295774646, "Y"=318.8895104895105}, {"X"=536.7549295774646, "Y"=319.8923076923077}, {"X"=535.7535211267605, "Y"=319.8923076923077}, {"X"=535.7535211267605, "Y"=320.8951048951049}, {"X"=534.7521126760562, "Y"=321.8979020979021}, {"X"=534.7521126760562, "Y"=322.90069930069933}, {"X"=534.7521126760562, "Y"=323.9034965034965}, {"X"=534.7521126760562, "Y"=324.90629370629375}, {"X"=533.750704225352, "Y"=325.90909090909093}, {"X"=532.7492957746477, "Y"=326.9118881118881}, {"X"=532.7492957746477, "Y"=327.91468531468536}, {"X"=532.7492957746477, "Y"=328.91748251748254}, {"X"=531.7478873239436, "Y"=329.9202797202797}, {"X"=531.7478873239436, "Y"=330.92307692307696}, {"X"=531.7478873239436, "Y"=331.92587412587415}, {"X"=531.7478873239436, "Y"=332.9286713286713}, {"X"=530.7464788732393, "Y"=332.9286713286713}, {"X"=530.7464788732393, "Y"=333.93146853146857}, {"X"=530.7464788732393, "Y"=334.93426573426575}, {"X"=530.7464788732393, "Y"=335.93706293706293}, {"X"=530.7464788732393, "Y"=336.9398601398602}, {"X"=531.7478873239436, "Y"=337.94265734265736}, {"X"=531.7478873239436, "Y"=338.94545454545454}, {"X"=531.7478873239436, "Y"=339.9482517482518}, {"X"=531.7478873239436, "Y"=340.95104895104896}, {"X"=531.7478873239436, "Y"=341.9538461538462}, {"X"=531.7478873239436, "Y"=342.9566433566434}, {"X"=532.7492957746477, "Y"=343.95944055944057}, {"X"=533.750704225352, "Y"=344.9622377622378}, {"X"=534.7521126760562, "Y"=344.9622377622378}, {"X"=535.7535211267605, "Y"=345.965034965035}, {"X"=536.7549295774646, "Y"=345.965034965035}, {"X"=537.7563380281689, "Y"=345.965034965035}, {"X"=539.7591549295773, "Y"=345.965034965035}, {"X"=541.7619718309858, "Y"=345.965034965035}, {"X"=542.76338028169, "Y"=345.965034965035}, {"X"=546.7690140845069, "Y"=344.9622377622378}, {"X"=549.7732394366196, "Y"=343.95944055944057}, {"X"=550.7746478873238, "Y"=343.95944055944057}, {"X"=552.7774647887322, "Y"=343.95944055944057}, {"X"=555.781690140845, "Y"=341.9538461538462}, {"X"=557.7845070422534, "Y"=340.95104895104896}, {"X"=561.7901408450703, "Y"=338.94545454545454}, {"X"=563.7929577464787, "Y"=336.9398601398602}, {"X"=566.7971830985914, "Y"=334.93426573426575}, {"X"=567.7985915492957, "Y"=334.93426573426575}, {"X"=569.8014084507041, "Y"=331.92587412587415}, {"X"=571.8042253521126, "Y"=329.9202797202797}, {"X"=572.8056338028167, "Y"=328.91748251748254}, {"X"=574.8084507042253, "Y"=325.90909090909093}, {"X"=577.8126760563379, "Y"=321.8979020979021}, {"X"=578.8140845070421, "Y"=320.8951048951049}, {"X"=580.8169014084506, "Y"=317.8867132867133}, {"X"=581.8183098591547, "Y"=315.8811188811189}, {"X"=583.8211267605633, "Y"=313.8755244755245}, {"X"=584.8225352112674, "Y"=311.8699300699301}, {"X"=584.8225352112674, "Y"=310.8671328671329}, {"X"=584.8225352112674, "Y"=309.86433566433567}, {"X"=584.8225352112674, "Y"=308.8615384615385}, {"X"=584.8225352112674, "Y"=307.8587412587413}, {"X"=584.8225352112674, "Y"=306.85594405594406}, {"X"=584.8225352112674, "Y"=305.8531468531469}, {"X"=584.8225352112674, "Y"=304.8503496503497}, {"X"=583.8211267605633, "Y"=304.8503496503497}, {"X"=581.8183098591547, "Y"=304.8503496503497}, {"X"=625.8802816901407, "Y"=303.84755244755246}, {"X"=623.8774647887323, "Y"=302.8447552447553}, {"X"=622.876056338028, "Y"=301.84195804195804}, {"X"=621.8746478873238, "Y"=301.84195804195804}, {"X"=620.8732394366195, "Y"=301.84195804195804}, {"X"=619.8718309859154, "Y"=301.84195804195804}, {"X"=618.8704225352111, "Y"=301.84195804195804}, {"X"=617.869014084507, "Y"=301.84195804195804}, {"X"=617.869014084507, "Y"=300.83916083916085}, {"X"=616.8676056338027, "Y"=300.83916083916085}, {"X"=615.8661971830984, "Y"=300.83916083916085}, {"X"=614.8647887323942, "Y"=300.83916083916085}, {"X"=613.86338028169, "Y"=300.83916083916085}, {"X"=613.86338028169, "Y"=301.84195804195804}, {"X"=612.8619718309858, "Y"=301.84195804195804}, {"X"=611.8605633802815, "Y"=301.84195804195804}, {"X"=610.8591549295774, "Y"=301.84195804195804}, {"X"=609.8577464788731, "Y"=302.8447552447553}, {"X"=608.8563380281689, "Y"=302.8447552447553}, {"X"=607.8549295774646, "Y"=303.84755244755246}, {"X"=606.8535211267604, "Y"=304.8503496503497}, {"X"=605.8521126760562, "Y"=304.8503496503497}, {"X"=604.8507042253519, "Y"=305.8531468531469}, {"X"=604.8507042253519, "Y"=306.85594405594406}, {"X"=603.8492957746478, "Y"=307.8587412587413}, {"X"=603.8492957746478, "Y"=308.8615384615385}, {"X"=603.8492957746478, "Y"=309.86433566433567}, {"X"=603.8492957746478, "Y"=310.8671328671329}, {"X"=603.8492957746478, "Y"=311.8699300699301}, {"X"=604.8507042253519, "Y"=311.8699300699301}, {"X"=604.8507042253519, "Y"=312.8727272727273}, {"X"=605.8521126760562, "Y"=313.8755244755245}, {"X"=606.8535211267604, "Y"=313.8755244755245}, {"X"=606.8535211267604, "Y"=314.8783216783217}, {"X"=608.8563380281689, "Y"=315.8811188811189}, {"X"=609.8577464788731, "Y"=316.8839160839161}, {"X"=610.8591549295774, "Y"=316.8839160839161}, {"X"=611.8605633802815, "Y"=317.8867132867133}, {"X"=612.8619718309858, "Y"=318.8895104895105}, {"X"=614.8647887323942, "Y"=319.8923076923077}, {"X"=615.8661971830984, "Y"=320.8951048951049}, {"X"=615.8661971830984, "Y"=321.8979020979021}, {"X"=617.869014084507, "Y"=322.90069930069933}, {"X"=617.869014084507, "Y"=323.9034965034965}, {"X"=618.8704225352111, "Y"=324.90629370629375}, {"X"=619.8718309859154, "Y"=325.90909090909093}, {"X"=619.8718309859154, "Y"=326.9118881118881}, {"X"=620.8732394366195, "Y"=328.91748251748254}, {"X"=621.8746478873238, "Y"=330.92307692307696}, {"X"=621.8746478873238, "Y"=331.92587412587415}, {"X"=621.8746478873238, "Y"=333.93146853146857}, {"X"=621.8746478873238, "Y"=335.93706293706293}, {"X"=621.8746478873238, "Y"=337.94265734265736}, {"X"=620.8732394366195, "Y"=338.94545454545454}, {"X"=620.8732394366195, "Y"=339.9482517482518}, {"X"=620.8732394366195, "Y"=340.95104895104896}, {"X"=620.8732394366195, "Y"=341.9538461538462}, {"X"=620.8732394366195, "Y"=342.9566433566434}, {"X"=620.8732394366195, "Y"=343.95944055944057}, {"X"=620.8732394366195, "Y"=344.9622377622378}, {"X"=620.8732394366195, "Y"=345.965034965035}, {"X"=619.8718309859154, "Y"=345.965034965035}, {"X"=619.8718309859154, "Y"=346.96783216783217}, {"X"=617.869014084507, "Y"=346.96783216783217}, {"X"=616.8676056338027, "Y"=346.96783216783217}, {"X"=614.8647887323942, "Y"=346.96783216783217}, {"X"=611.8605633802815, "Y"=347.9706293706294}, {"X"=610.8591549295774, "Y"=347.9706293706294}, {"X"=608.8563380281689, "Y"=347.9706293706294}, {"X"=607.8549295774646, "Y"=347.9706293706294}, {"X"=603.8492957746478, "Y"=347.9706293706294}, {"X"=600.8450704225351, "Y"=346.96783216783217}, {"X"=595.8380281690139, "Y"=346.96783216783217}, {"X"=593.8352112676055, "Y"=346.96783216783217}, {"X"=588.8281690140843, "Y"=346.96783216783217}, {"X"=585.8239436619717, "Y"=346.96783216783217}, {"X"=584.8225352112674, "Y"=346.96783216783217}, {"X"=583.8211267605633, "Y"=346.96783216783217}, {"X"=582.819718309859, "Y"=346.96783216783217}, {"X"=581.8183098591547, "Y"=346.96783216783217}, {"X"=580.8169014084506, "Y"=345.965034965035}, {"X"=580.8169014084506, "Y"=344.9622377622378}, {"X"=655.9225352112675, "Y"=307.8587412587413}, {"X"=654.9211267605632, "Y"=311.8699300699301}, {"X"=653.919718309859, "Y"=312.8727272727273}, {"X"=653.919718309859, "Y"=314.8783216783217}, {"X"=652.9183098591548, "Y"=316.8839160839161}, {"X"=652.9183098591548, "Y"=317.8867132867133}, {"X"=651.9169014084506, "Y"=318.8895104895105}, {"X"=651.9169014084506, "Y"=319.8923076923077}, {"X"=650.9154929577463, "Y"=320.8951048951049}, {"X"=649.914084507042, "Y"=323.9034965034965}, {"X"=649.914084507042, "Y"=324.90629370629375}, {"X"=648.9126760563379, "Y"=326.9118881118881}, {"X"=647.9112676056336, "Y"=327.91468531468536}, {"X"=647.9112676056336, "Y"=329.9202797202797}, {"X"=645.9084507042252, "Y"=331.92587412587415}, {"X"=645.9084507042252, "Y"=332.9286713286713}, {"X"=644.907042253521, "Y"=335.93706293706293}, {"X"=643.9056338028167, "Y"=336.9398601398602}, {"X"=642.9042253521126, "Y"=338.94545454545454}, {"X"=641.9028169014083, "Y"=340.95104895104896}, {"X"=640.901408450704, "Y"=341.9538461538462}, {"X"=640.901408450704, "Y"=342.9566433566434}, {"X"=640.901408450704, "Y"=343.95944055944057}, {"X"=639.8999999999999, "Y"=345.965034965035}, {"X"=637.8971830985914, "Y"=347.9706293706294}, {"X"=637.8971830985914, "Y"=348.9734265734266}, {"X"=636.8957746478872, "Y"=350.979020979021}, {"X"=636.8957746478872, "Y"=351.9818181818182}, {"X"=635.894366197183, "Y"=351.9818181818182}, {"X"=635.894366197183, "Y"=352.9846153846154}, {"X"=634.8929577464787, "Y"=353.9874125874126}, {"X"=634.8929577464787, "Y"=354.9902097902098}, {"X"=633.8915492957744, "Y"=355.993006993007}, {"X"=632.8901408450703, "Y"=356.9958041958042}, {"X"=631.888732394366, "Y"=357.9986013986014}, {"X"=631.888732394366, "Y"=359.0013986013986}, {"X"=632.8901408450703, "Y"=359.0013986013986}, {"X"=633.8915492957744, "Y"=357.9986013986014}, {"X"=634.8929577464787, "Y"=357.9986013986014}, {"X"=635.894366197183, "Y"=357.9986013986014}, {"X"=636.8957746478872, "Y"=356.9958041958042}, {"X"=637.8971830985914, "Y"=356.9958041958042}, {"X"=638.8985915492956, "Y"=356.9958041958042}, {"X"=640.901408450704, "Y"=355.993006993007}, {"X"=642.9042253521126, "Y"=355.993006993007}, {"X"=644.907042253521, "Y"=354.9902097902098}, {"X"=645.9084507042252, "Y"=353.9874125874126}, {"X"=647.9112676056336, "Y"=352.9846153846154}, {"X"=649.914084507042, "Y"=352.9846153846154}, {"X"=651.9169014084506, "Y"=351.9818181818182}, {"X"=652.9183098591548, "Y"=351.9818181818182}, {"X"=656.9239436619716, "Y"=350.979020979021}, {"X"=657.9253521126759, "Y"=350.979020979021}, {"X"=659.9281690140843, "Y"=349.9762237762238}, {"X"=660.9295774647886, "Y"=349.9762237762238}, {"X"=664.9352112676055, "Y"=349.9762237762238}, {"X"=666.9380281690139, "Y"=349.9762237762238}, {"X"=667.9394366197181, "Y"=349.9762237762238}, {"X"=668.9408450704224, "Y"=349.9762237762238}, {"X"=669.9422535211266, "Y"=349.9762237762238}, {"X"=671.9450704225351, "Y"=349.9762237762238}, {"X"=672.9464788732392, "Y"=349.9762237762238}, {"X"=673.9478873239435, "Y"=349.9762237762238}, {"X"=674.9492957746477, "Y"=350.979020979021}, {"X"=675.950704225352, "Y"=350.979020979021}, {"X"=676.9521126760562, "Y"=350.979020979021}, {"X"=677.9535211267604, "Y"=350.979020979021}, {"X"=678.9549295774647, "Y"=350.979020979021}, {"X"=677.9535211267604, "Y"=350.979020979021}, {"X"=677.9535211267604, "Y"=351.9818181818182}, {"X"=677.9535211267604, "Y"=350.979020979021}, {"X"=695.9788732394364, "Y"=309.86433566433567}, {"X"=697.9816901408449, "Y"=311.8699300699301}, {"X"=699.9845070422533, "Y"=314.8783216783217}, {"X"=701.9873239436617, "Y"=315.8811188811189}, {"X"=703.9901408450703, "Y"=317.8867132867133}, {"X"=704.9915492957745, "Y"=319.8923076923077}, {"X"=706.9943661971829, "Y"=321.8979020979021}, {"X"=707.9957746478872, "Y"=322.90069930069933}, {"X"=707.9957746478872, "Y"=324.90629370629375}, {"X"=708.9971830985913, "Y"=325.90909090909093}, {"X"=709.9985915492956, "Y"=326.9118881118881}, {"X"=709.9985915492956, "Y"=327.91468531468536}, {"X"=710.9999999999998, "Y"=328.91748251748254}, {"X"=710.9999999999998, "Y"=329.9202797202797}, {"X"=712.001408450704, "Y"=330.92307692307696}, {"X"=712.001408450704, "Y"=331.92587412587415}, {"X"=712.001408450704, "Y"=332.9286713286713}, {"X"=712.001408450704, "Y"=331.92587412587415}, {"X"=710.9999999999998, "Y"=331.92587412587415}, {"X"=728.0239436619717, "Y"=308.8615384615385}, {"X"=727.0225352112674, "Y"=309.86433566433567}, {"X"=726.0211267605632, "Y"=309.86433566433567}, {"X"=725.019718309859, "Y"=310.8671328671329}, {"X"=724.0183098591548, "Y"=311.8699300699301}, {"X"=723.0169014084505, "Y"=313.8755244755245}, {"X"=721.0140845070421, "Y"=314.8783216783217}, {"X"=720.0126760563379, "Y"=316.8839160839161}, {"X"=718.0098591549294, "Y"=318.8895104895105}, {"X"=716.0070422535209, "Y"=322.90069930069933}, {"X"=714.0042253521125, "Y"=323.9034965034965}, {"X"=710.9999999999998, "Y"=327.91468531468536}, {"X"=709.9985915492956, "Y"=328.91748251748254}, {"X"=706.9943661971829, "Y"=331.92587412587415}, {"X"=704.9915492957745, "Y"=334.93426573426575}, {"X"=702.988732394366, "Y"=335.93706293706293}, {"X"=700.9859154929576, "Y"=338.94545454545454}, {"X"=699.9845070422533, "Y"=339.9482517482518}, {"X"=697.9816901408449, "Y"=341.9538461538462}, {"X"=697.9816901408449, "Y"=342.9566433566434}, {"X"=695.9788732394364, "Y"=344.9622377622378}, {"X"=694.9774647887323, "Y"=346.96783216783217}, {"X"=693.976056338028, "Y"=347.9706293706294}, {"X"=692.9746478873237, "Y"=349.9762237762238}, {"X"=691.9732394366196, "Y"=349.9762237762238}, {"X"=690.9718309859153, "Y"=350.979020979021}, {"X"=690.9718309859153, "Y"=351.9818181818182}, {"X"=689.9704225352111, "Y"=352.9846153846154}, {"X"=688.9690140845069, "Y"=352.9846153846154}, {"X"=688.9690140845069, "Y"=353.9874125874126}, {"X"=687.9676056338027, "Y"=354.9902097902098}, {"X"=686.9661971830984, "Y"=355.993006993007}, {"X"=686.9661971830984, "Y"=356.9958041958042}, {"X"=686.9661971830984, "Y"=355.993006993007}, {"X"=686.9661971830984, "Y"=354.9902097902098}, {"X"=813.1436619718307, "Y"=258.7216783216783}, {"X"=806.1338028169013, "Y"=271.758041958042}, {"X"=802.1281690140843, "Y"=278.7776223776224}, {"X"=798.1225352112674, "Y"=286.8}, {"X"=793.1154929577463, "Y"=297.83076923076925}, {"X"=792.1140845070421, "Y"=300.83916083916085}, {"X"=789.1098591549294, "Y"=306.85594405594406}, {"X"=786.1056338028167, "Y"=313.8755244755245}, {"X"=782.0999999999998, "Y"=321.8979020979021}, {"X"=779.0957746478871, "Y"=330.92307692307696}, {"X"=778.0943661971829, "Y"=332.9286713286713}, {"X"=777.0929577464786, "Y"=336.9398601398602}, {"X"=776.0915492957745, "Y"=337.94265734265736}, {"X"=776.0915492957745, "Y"=339.9482517482518}, {"X"=776.0915492957745, "Y"=340.95104895104896}, {"X"=776.0915492957745, "Y"=341.9538461538462}, {"X"=775.0901408450702, "Y"=342.9566433566434}, {"X"=775.0901408450702, "Y"=343.95944055944057}, {"X"=775.0901408450702, "Y"=344.9622377622378}, {"X"=775.0901408450702, "Y"=345.965034965035}, {"X"=774.088732394366, "Y"=345.965034965035}, {"X"=774.088732394366, "Y"=346.96783216783217}, {"X"=774.088732394366, "Y"=345.965034965035}, {"X"=775.0901408450702, "Y"=345.965034965035}, {"X"=775.0901408450702, "Y"=344.9622377622378}, {"X"=776.0915492957745, "Y"=343.95944055944057}, {"X"=776.0915492957745, "Y"=342.9566433566434}, {"X"=776.0915492957745, "Y"=341.9538461538462}, {"X"=774.088732394366, "Y"=368.02657342657346}, {"X"=776.0915492957745, "Y"=366.02097902097904}, {"X"=777.0929577464786, "Y"=366.02097902097904}, {"X"=778.0943661971829, "Y"=367.0237762237762}, {"X"=778.0943661971829, "Y"=368.02657342657346}, {"X"=777.0929577464786, "Y"=370.03216783216783}, {"X"=776.0915492957745, "Y"=371.03496503496507}, {"X"=775.0901408450702, "Y"=372.03776223776225}, {"X"=774.088732394366, "Y"=373.04055944055943}, {"X"=772.0859154929576, "Y"=374.0433566433567}, {"X"=771.0845070422533, "Y"=374.0433566433567}, {"X"=770.0830985915491, "Y"=372.03776223776225}, {"X"=770.0830985915491, "Y"=371.03496503496507}, {"X"=770.0830985915491, "Y"=370.03216783216783}, {"X"=771.0845070422533, "Y"=369.02937062937065}, {"X"=774.088732394366, "Y"=368.02657342657346}, {"X"=775.0901408450702, "Y"=368.02657342657346}, {"X"=775.0901408450702, "Y"=369.02937062937065}, {"X"=774.088732394366, "Y"=369.02937062937065}, {"X"=774.088732394366, "Y"=370.03216783216783}, {"X"=773.0873239436618, "Y"=370.03216783216783}, {"X"=772.0859154929576, "Y"=369.02937062937065}, {"X"=864.2154929577463, "Y"=266.74405594405596}, {"X"=862.2126760563378, "Y"=270.7552447552448}, {"X"=861.2112676056336, "Y"=272.76083916083917}, {"X"=861.2112676056336, "Y"=274.7664335664336}, {"X"=859.2084507042251, "Y"=277.7748251748252}, {"X"=858.207042253521, "Y"=280.7832167832168}, {"X"=856.2042253521124, "Y"=283.7916083916084}, {"X"=854.201408450704, "Y"=286.8}, {"X"=852.1985915492955, "Y"=291.81398601398604}, {"X"=851.1971830985914, "Y"=294.82237762237764}, {"X"=849.194366197183, "Y"=300.83916083916085}, {"X"=847.1915492957744, "Y"=303.84755244755246}, {"X"=845.188732394366, "Y"=308.8615384615385}, {"X"=844.1873239436618, "Y"=310.8671328671329}, {"X"=842.1845070422534, "Y"=314.8783216783217}, {"X"=839.1802816901406, "Y"=321.8979020979021}, {"X"=838.1788732394364, "Y"=324.90629370629375}, {"X"=835.1746478873238, "Y"=330.92307692307696}, {"X"=834.1732394366195, "Y"=333.93146853146857}, {"X"=832.1704225352111, "Y"=338.94545454545454}, {"X"=831.1690140845069, "Y"=340.95104895104896}, {"X"=830.1676056338026, "Y"=344.9622377622378}, {"X"=829.1661971830983, "Y"=346.96783216783217}, {"X"=827.1633802816899, "Y"=350.979020979021}, {"X"=827.1633802816899, "Y"=352.9846153846154}, {"X"=826.1619718309857, "Y"=354.9902097902098}, {"X"=825.1605633802815, "Y"=355.993006993007}, {"X"=825.1605633802815, "Y"=357.9986013986014}, {"X"=825.1605633802815, "Y"=359.0013986013986}, {"X"=825.1605633802815, "Y"=360.00419580419583}, {"X"=824.1591549295773, "Y"=360.00419580419583}, {"X"=824.1591549295773, "Y"=361.006993006993}, {"X"=824.1591549295773, "Y"=362.00979020979025}, {"X"=823.157746478873, "Y"=363.01258741258744}, {"X"=823.157746478873, "Y"=364.0153846153846}, {"X"=823.157746478873, "Y"=363.01258741258744}, {"X"=823.157746478873, "Y"=362.00979020979025}, {"X"=825.1605633802815, "Y"=383.0685314685315}, {"X"=822.1563380281688, "Y"=383.0685314685315}, {"X"=821.1549295774646, "Y"=382.0657342657343}, {"X"=821.1549295774646, "Y"=381.06293706293707}, {"X"=821.1549295774646, "Y"=380.0601398601399}, {"X"=822.1563380281688, "Y"=379.0573426573427}, {"X"=824.1591549295773, "Y"=379.0573426573427}, {"X"=825.1605633802815, "Y"=379.0573426573427}, {"X"=827.1633802816899, "Y"=379.0573426573427}, {"X"=828.1647887323942, "Y"=381.06293706293707}, {"X"=828.1647887323942, "Y"=382.0657342657343}, {"X"=827.1633802816899, "Y"=382.0657342657343}, {"X"=826.1619718309857, "Y"=383.0685314685315}, {"X"=825.1605633802815, "Y"=383.0685314685315}, {"X"=824.1591549295773, "Y"=383.0685314685315}, {"X"=823.157746478873, "Y"=382.0657342657343}, {"X"=819.1521126760562, "Y"=381.06293706293707}, {"X"=818.1507042253519, "Y"=382.0657342657343}, {"X"=819.1521126760562, "Y"=382.0657342657343}, {"X"=821.1549295774646, "Y"=382.0657342657343}, {"X"=823.157746478873, "Y"=382.0657342657343}, {"X"=825.1605633802815, "Y"=382.0657342657343}, {"X"=828.1647887323942, "Y"=383.0685314685315}, {"X"=830.1676056338026, "Y"=383.0685314685315}, {"X"=832.1704225352111, "Y"=383.0685314685315}, {"X"=834.1732394366195, "Y"=383.0685314685315}, {"X"=836.1760563380279, "Y"=384.0713286713287}, {"X"=838.1788732394364, "Y"=385.0741258741259}, {"X"=840.1816901408449, "Y"=386.0769230769231}, {"X"=844.1873239436618, "Y"=387.0797202797203}, {"X"=848.1929577464787, "Y"=389.0853146853147}, {"X"=850.1957746478871, "Y"=390.0881118881119}, {"X"=851.1971830985914, "Y"=391.0909090909091}, {"X"=854.201408450704, "Y"=394.0993006993007}, {"X"=856.2042253521124, "Y"=395.1020979020979}, {"X"=857.2056338028167, "Y"=398.1104895104895}, {"X"=857.2056338028167, "Y"=402.12167832167836}, {"X"=857.2056338028167, "Y"=405.13006993006996}, {"X"=854.201408450704, "Y"=409.14125874125875}, {"X"=853.1999999999998, "Y"=411.1468531468532}, {"X"=850.1957746478871, "Y"=414.1552447552448}, {"X"=848.1929577464787, "Y"=416.1608391608392}, {"X"=841.1830985915491, "Y"=420.172027972028}, {"X"=837.1774647887322, "Y"=422.1776223776224}, {"X"=825.1605633802815, "Y"=428.1944055944056}, {"X"=819.1521126760562, "Y"=430.2}, {"X"=807.1352112676054, "Y"=434.21118881118883}, {"X"=801.1267605633801, "Y"=435.213986013986}, {"X"=786.1056338028167, "Y"=438.2223776223776}, {"X"=777.0929577464786, "Y"=439.22517482517486}, {"X"=756.06338028169, "Y"=441.2307692307692}, {"X"=746.0492957746477, "Y"=441.2307692307692}, {"X"=721.0140845070421, "Y"=442.23356643356647}, {"X"=712.001408450704, "Y"=442.23356643356647}, {"X"=692.9746478873237, "Y"=442.23356643356647}, {"X"=684.96338028169, "Y"=442.23356643356647}, {"X"=668.9408450704224, "Y"=442.23356643356647}, {"X"=660.9295774647886, "Y"=442.23356643356647}, {"X"=646.9098591549294, "Y"=441.2307692307692}, {"X"=636.8957746478872, "Y"=440.22797202797204}, {"X"=623.8774647887323, "Y"=439.22517482517486}, {"X"=616.8676056338027, "Y"=439.22517482517486}, {"X"=603.8492957746478, "Y"=438.2223776223776}, {"X"=592.8338028169013, "Y"=437.21958041958044}, {"X"=578.8140845070421, "Y"=435.213986013986}, {"X"=571.8042253521126, "Y"=435.213986013986}, {"X"=555.781690140845, "Y"=433.20839160839165}, {"X"=543.7647887323942, "Y"=431.2027972027972}, {"X"=527.7422535211266, "Y"=429.1972027972028}, {"X"=519.7309859154929, "Y"=429.1972027972028}, {"X"=503.70845070422524, "Y"=427.1916083916084}, {"X"=496.69859154929566, "Y"=425.186013986014}, {"X"=488.6873239436618, "Y"=424.1832167832168}, {"X"=473.66619718309846, "Y"=422.1776223776224}, {"X"=459.6464788732393, "Y"=421.1748251748252}, {"X"=453.638028169014, "Y"=421.1748251748252}, {"X"=444.62535211267596, "Y"=420.172027972028}, {"X"=440.6197183098591, "Y"=420.172027972028}, {"X"=436.61408450704215, "Y"=420.172027972028}, {"X"=423.5957746478872, "Y"=420.172027972028}, {"X"=412.58028169014074, "Y"=421.1748251748252}, {"X"=407.5732394366196, "Y"=421.1748251748252}, {"X"=401.5647887323943, "Y"=421.1748251748252}, {"X"=388.5464788732393, "Y"=422.1776223776224}, {"X"=382.538028169014, "Y"=423.1804195804196}, {"X"=364.5126760563379, "Y"=425.186013986014}, {"X"=357.5028169014084, "Y"=427.1916083916084}, {"X"=346.48732394366186, "Y"=428.1944055944056}, {"X"=341.48028169014077, "Y"=429.1972027972028}, {"X"=329.46338028169004, "Y"=432.2055944055944}, {"X"=323.4549295774647, "Y"=434.21118881118883}, {"X"=312.4394366197182, "Y"=437.21958041958044}, {"X"=306.4309859154929, "Y"=439.22517482517486}, {"X"=300.42253521126753, "Y"=440.22797202797204}, {"X"=288.40563380281685, "Y"=445.24195804195807}, {"X"=283.3985915492957, "Y"=447.24755244755244}, {"X"=268.3774647887323, "Y"=453.2643356643357}, {"X"=263.3704225352112, "Y"=455.26993006993007}, {"X"=253.35633802816892, "Y"=460.2839160839161}, {"X"=249.35070422535205, "Y"=462.28951048951046}, {"X"=242.34084507042246, "Y"=468.30629370629373}, {"X"=238.3352112676056, "Y"=472.3174825174825}, {"X"=233.32816901408444, "Y"=480.33986013986015}, {"X"=231.325352112676, "Y"=484.35104895104894}, {"X"=228.32112676056335, "Y"=493.3762237762238}, {"X"=227.31971830985907, "Y"=497.3874125874126}, {"X"=226.31830985915485, "Y"=503.4041958041958}, {"X"=226.31830985915485, "Y"=506.4125874125874}, {"X"=226.31830985915485, "Y"=512.4293706293706}, {"X"=227.31971830985907, "Y"=515.4377622377623}, {"X"=228.32112676056335, "Y"=520.4517482517483}, {"X"=230.32394366197178, "Y"=523.4601398601399}, {"X"=232.32676056338022, "Y"=526.4685314685314}, {"X"=237.33380281690137, "Y"=531.4825174825176}, {"X"=240.33802816901402, "Y"=532.4853146853147}, {"X"=251.35352112676048, "Y"=535.4937062937063}, {"X"=257.36197183098585, "Y"=535.4937062937063}, {"X"=271.381690140845, "Y"=535.4937062937063}, {"X"=278.39154929577455, "Y"=535.4937062937063}, {"X"=293.41267605633794, "Y"=534.4909090909091}, {"X"=307.4323943661971, "Y"=533.4881118881119}, {"X"=325.45774647887316, "Y"=532.4853146853147}, {"X"=335.4718309859154, "Y"=531.4825174825176}, {"X"=343.4830985915492, "Y"=531.4825174825176}, {"X"=367.5169014084506, "Y"=530.4797202797203}, {"X"=376.52957746478864, "Y"=529.4769230769231}, {"X"=393.5535211267605, "Y"=529.4769230769231}, {"X"=402.5661971830985, "Y"=529.4769230769231}, {"X"=422.594366197183, "Y"=530.4797202797203}, {"X"=429.60422535211256, "Y"=531.4825174825176}, {"X"=444.62535211267596, "Y"=534.4909090909091}, {"X"=450.63380281690127, "Y"=536.4965034965035}, {"X"=462.650704225352, "Y"=539.5048951048951}, {"X"=468.6591549295773, "Y"=541.5104895104895}, {"X"=479.6746478873238, "Y"=546.5244755244755}, {"X"=483.68028169014076, "Y"=548.5300699300699}, {"X"=489.68873239436607, "Y"=554.5468531468532}, {"X"=491.6915492957745, "Y"=557.5552447552448}, {"X"=495.6971830985914, "Y"=564.5748251748252}, {"X"=496.69859154929566, "Y"=568.586013986014}, {"X"=495.6971830985914, "Y"=576.6083916083917}, {"X"=494.6957746478872, "Y"=581.6223776223776}, {"X"=490.69014084507035, "Y"=589.6447552447553}, {"X"=487.68591549295763, "Y"=592.6531468531468}, {"X"=482.6788732394365, "Y"=598.66993006993}, {"X"=477.67183098591534, "Y"=600.6755244755245}, {"X"=468.6591549295773, "Y"=603.6839160839161}, {"X"=463.6521126760563, "Y"=604.6867132867133}, {"X"=454.63943661971814, "Y"=606.6923076923077}, {"X"=444.62535211267596, "Y"=607.6951048951049}, {"X"=439.6183098591548, "Y"=607.6951048951049}, {"X"=435.61267605633793, "Y"=608.6979020979021}, {"X"=422.594366197183, "Y"=608.6979020979021}, {"X"=418.5887323943661, "Y"=608.6979020979021}, {"X"=410.5774647887323, "Y"=609.7006993006993}, {"X"=407.5732394366196, "Y"=609.7006993006993}, {"X"=399.56197183098584, "Y"=610.7034965034965}, {"X"=396.5577464788731, "Y"=611.7062937062938}, {"X"=392.55211267605625, "Y"=613.7118881118881}, {"X"=391.55070422535204, "Y"=614.7146853146853}, {"X"=390.54929577464776, "Y"=616.7202797202797}, {"X"=389.54788732394354, "Y"=618.7258741258742}, {"X"=388.5464788732393, "Y"=620.7314685314685}, {"X"=387.5450704225351, "Y"=623.7398601398602}, {"X"=387.5450704225351, "Y"=624.7426573426574}, {"X"=387.5450704225351, "Y"=625.7454545454545}, {"X"=387.5450704225351, "Y"=627.7510489510489}, {"X"=387.5450704225351, "Y"=628.7538461538461}, {"X"=388.5464788732393, "Y"=630.7594405594406}, {"X"=389.54788732394354, "Y"=631.7622377622378}, {"X"=391.55070422535204, "Y"=632.7650349650349}, {"X"=394.5549295774647, "Y"=634.7706293706294}, {"X"=396.5577464788731, "Y"=634.7706293706294}, {"X"=400.56338028169006, "Y"=635.7734265734266}, {"X"=402.5661971830985, "Y"=636.7762237762238}, {"X"=404.56901408450693, "Y"=636.7762237762238}, {"X"=405.57042253521115, "Y"=636.7762237762238}, {"X"=406.57183098591537, "Y"=635.7734265734266}, {"X"=406.57183098591537, "Y"=636.7762237762238}, {"X"=405.57042253521115, "Y"=636.7762237762238}, {"X"=404.56901408450693, "Y"=635.7734265734266}, {"X"=403.5676056338027, "Y"=635.7734265734266}] ("XY Graph")
  (unwired) cluster{"Horizontal":i32, "Vertical":i32}[] [{"Horizontal"=354, "Vertical"=79}, {"Horizontal"=359, "Vertical"=724}, {"Horizontal"=928, "Vertical"=727}, {"Horizontal"=920, "Vertical"=76}, {"Horizontal"=375, "Vertical"=75}, {"Horizontal"=348, "Vertical"=534}, {"Horizontal"=379, "Vertical"=519}, {"Horizontal"=407, "Vertical"=510}, {"Horizontal"=436, "Vertical"=501}, {"Horizontal"=463, "Vertical"=490}, {"Horizontal"=491, "Vertical"=484}, {"Horizontal"=514, "Vertical"=473}, {"Horizontal"=528, "Vertical"=466}, {"Horizontal"=536, "Vertical"=452}, {"Horizontal"=523, "Vertical"=437}, {"Horizontal"=518, "Vertical"=417}, {"Horizontal"=512, "Vertical"=396}, {"Horizontal"=508, "Vertical"=372}, {"Horizontal"=503, "Vertical"=348}, {"Horizontal"=490, "Vertical"=331}, {"Horizontal"=491, "Vertical"=315}, {"Horizontal"=502, "Vertical"=290}, {"Horizontal"=511, "Vertical"=302}, {"Horizontal"=520, "Vertical"=312}, {"Horizontal"=529, "Vertical"=324}, {"Horizontal"=531, "Vertical"=338}, {"Horizontal"=536, "Vertical"=353}, {"Horizontal"=547, "Vertical"=354}, {"Horizontal"=563, "Vertical"=359}, {"Horizontal"=570, "Vertical"=361}, {"Horizontal"=586, "Vertical"=363}, {"Horizontal"=595, "Vertical"=363}, {"Horizontal"=610, "Vertical"=363}, {"Horizontal"=617, "Vertical"=349}, {"Horizontal"=623, "Vertical"=335}, {"Horizontal"=629, "Vertical"=318}, {"Horizontal"=618, "Vertical"=309}, {"Horizontal"=601, "Vertical"=306}, {"Horizontal"=587, "Vertical"=303}, {"Horizontal"=567, "Vertical"=299}, {"Horizontal"=551, "Vertical"=301}, {"Horizontal"=539, "Vertical"=305}, {"Horizontal"=529, "Vertical"=306}, {"Horizontal"=520, "Vertical"=296}, {"Horizontal"=512, "Vertical"=281}, {"Horizontal"=506, "Vertical"=277}, {"Horizontal"=502, "Vertical"=269}, {"Horizontal"=508, "Vertical"=250}, {"Horizontal"=516, "Vertical"=232}, {"Horizontal"=525, "Vertical"=213}, {"Horizontal"=539, "Vertical"=188}, {"Horizontal"=547, "Vertical"=174}, {"Horizontal"=563, "Vertical"=162}, {"Horizontal"=579, "Vertical"=144}, {"Horizontal"=587, "Vertical"=136}, {"Horizontal"=610, "Vertical"=128}, {"Horizontal"=629, "Vertical"=129}, {"Horizontal"=656, "Vertical"=127}, {"Horizontal"=666, "Vertical"=131}, {"Horizontal"=697, "Vertical"=140}, {"Horizontal"=711, "Vertical"=143}, {"Horizontal"=745, "Vertical"=163}, {"Horizontal"=750, "Vertical"=169}, {"Horizontal"=757, "Vertical"=193}, {"Horizontal"=771, "Vertical"=200}, {"Horizontal"=767, "Vertical"=224}, {"Horizontal"=774, "Vertical"=238}, {"Horizontal"=779, "Vertical"=268}, {"Horizontal"=783, "Vertical"=284}, {"Horizontal"=765, "Vertical"=286}, {"Horizontal"=746, "Vertical"=291}, {"Horizontal"=737, "Vertical"=300}, {"Horizontal"=718, "Vertical"=302}, {"Horizontal"=696, "Vertical"=299}, {"Horizontal"=679, "Vertical"=302}, {"Horizontal"=655, "Vertical"=304}, {"Horizontal"=650, "Vertical"=306}, {"Horizontal"=636, "Vertical"=308}, {"Horizontal"=620, "Vertical"=309}, {"Horizontal"=643, "Vertical"=317}, {"Horizontal"=651, "Vertical"=334}, {"Horizontal"=656, "Vertical"=342}, {"Horizontal"=664, "Vertical"=358}, {"Horizontal"=674, "Vertical"=367}, {"Horizontal"=689, "Vertical"=360}, {"Horizontal"=712, "Vertical"=361}, {"Horizontal"=731, "Vertical"=353}, {"Horizontal"=738, "Vertical"=346}, {"Horizontal"=747, "Vertical"=326}, {"Horizontal"=744, "Vertical"=315}, {"Horizontal"=751, "Vertical"=304}, {"Horizontal"=759, "Vertical"=294}, {"Horizontal"=773, "Vertical"=291}, {"Horizontal"=785, "Vertical"=286}, {"Horizontal"=770, "Vertical"=296}, {"Horizontal"=778, "Vertical"=306}, {"Horizontal"=776, "Vertical"=317}, {"Horizontal"=775, "Vertical"=326}, {"Horizontal"=773, "Vertical"=340}, {"Horizontal"=771, "Vertical"=353}, {"Horizontal"=765, "Vertical"=360}, {"Horizontal"=762, "Vertical"=383}, {"Horizontal"=763, "Vertical"=406}, {"Horizontal"=761, "Vertical"=420}, {"Horizontal"=778, "Vertical"=434}, {"Horizontal"=782, "Vertical"=446}, {"Horizontal"=798, "Vertical"=459}, {"Horizontal"=811, "Vertical"=468}, {"Horizontal"=829, "Vertical"=476}, {"Horizontal"=847, "Vertical"=485}, {"Horizontal"=865, "Vertical"=489}, {"Horizontal"=878, "Vertical"=495}, {"Horizontal"=891, "Vertical"=500}, {"Horizontal"=903, "Vertical"=505}, {"Horizontal"=926, "Vertical"=511}, {"Horizontal"=912, "Vertical"=713}, {"Horizontal"=794, "Vertical"=706}, {"Horizontal"=812, "Vertical"=684}, {"Horizontal"=820, "Vertical"=665}, {"Horizontal"=829, "Vertical"=650}, {"Horizontal"=835, "Vertical"=631}, {"Horizontal"=844, "Vertical"=612}, {"Horizontal"=853, "Vertical"=594}, {"Horizontal"=859, "Vertical"=579}, {"Horizontal"=851, "Vertical"=571}, {"Horizontal"=840, "Vertical"=563}, {"Horizontal"=827, "Vertical"=556}, {"Horizontal"=837, "Vertical"=547}, {"Horizontal"=849, "Vertical"=536}, {"Horizontal"=851, "Vertical"=528}, {"Horizontal"=844, "Vertical"=519}, {"Horizontal"=840, "Vertical"=498}, {"Horizontal"=832, "Vertical"=485}, {"Horizontal"=829, "Vertical"=473}, {"Horizontal"=758, "Vertical"=419}, {"Horizontal"=760, "Vertical"=437}, {"Horizontal"=762, "Vertical"=465}, {"Horizontal"=755, "Vertical"=482}, {"Horizontal"=751, "Vertical"=506}, {"Horizontal"=744, "Vertical"=525}, {"Horizontal"=739, "Vertical"=547}, {"Horizontal"=731, "Vertical"=561}, {"Horizontal"=726, "Vertical"=580}, {"Horizontal"=723, "Vertical"=604}, {"Horizontal"=719, "Vertical"=620}, {"Horizontal"=715, "Vertical"=637}, {"Horizontal"=706, "Vertical"=665}, {"Horizontal"=705, "Vertical"=683}, {"Horizontal"=701, "Vertical"=700}, {"Horizontal"=698, "Vertical"=709}, {"Horizontal"=694, "Vertical"=718}, {"Horizontal"=689, "Vertical"=722}, {"Horizontal"=676, "Vertical"=712}, {"Horizontal"=674, "Vertical"=695}, {"Horizontal"=667, "Vertical"=682}, {"Horizontal"=671, "Vertical"=666}, {"Horizontal"=660, "Vertical"=646}, {"Horizontal"=664, "Vertical"=635}, {"Horizontal"=668, "Vertical"=624}, {"Horizontal"=675, "Vertical"=620}, {"Horizontal"=679, "Vertical"=623}, {"Horizontal"=692, "Vertical"=630}, {"Horizontal"=693, "Vertical"=633}, {"Horizontal"=698, "Vertical"=635}, {"Horizontal"=711, "Vertical"=628}, {"Horizontal"=721, "Vertical"=615}, {"Horizontal"=726, "Vertical"=586}, {"Horizontal"=746, "Vertical"=531}, {"Horizontal"=758, "Vertical"=482}, {"Horizontal"=753, "Vertical"=456}, {"Horizontal"=740, "Vertical"=475}, {"Horizontal"=727, "Vertical"=490}, {"Horizontal"=713, "Vertical"=503}, {"Horizontal"=696, "Vertical"=531}, {"Horizontal"=683, "Vertical"=529}, {"Horizontal"=671, "Vertical"=538}, {"Horizontal"=659, "Vertical"=550}, {"Horizontal"=642, "Vertical"=552}, {"Horizontal"=628, "Vertical"=553}, {"Horizontal"=602, "Vertical"=550}, {"Horizontal"=592, "Vertical"=529}, {"Horizontal"=586, "Vertical"=528}, {"Horizontal"=579, "Vertical"=519}, {"Horizontal"=570, "Vertical"=508}, {"Horizontal"=564, "Vertical"=492}, {"Horizontal"=557, "Vertical"=481}, {"Horizontal"=553, "Vertical"=470}, {"Horizontal"=548, "Vertical"=456}, {"Horizontal"=540, "Vertical"=468}, {"Horizontal"=541, "Vertical"=485}, {"Horizontal"=542, "Vertical"=508}, {"Horizontal"=539, "Vertical"=527}, {"Horizontal"=544, "Vertical"=555}, {"Horizontal"=543, "Vertical"=588}, {"Horizontal"=539, "Vertical"=614}, {"Horizontal"=539, "Vertical"=631}, {"Horizontal"=539, "Vertical"=656}, {"Horizontal"=542, "Vertical"=673}, {"Horizontal"=539, "Vertical"=687}, {"Horizontal"=545, "Vertical"=712}, {"Horizontal"=542, "Vertical"=723}, {"Horizontal"=547, "Vertical"=727}, {"Horizontal"=572, "Vertical"=724}, {"Horizontal"=578, "Vertical"=696}, {"Horizontal"=578, "Vertical"=682}, {"Horizontal"=586, "Vertical"=659}, {"Horizontal"=588, "Vertical"=638}, {"Horizontal"=593, "Vertical"=613}, {"Horizontal"=601, "Vertical"=601}, {"Horizontal"=609, "Vertical"=614}, {"Horizontal"=613, "Vertical"=626}, {"Horizontal"=625, "Vertical"=640}, {"Horizontal"=614, "Vertical"=670}, {"Horizontal"=610, "Vertical"=680}, {"Horizontal"=604, "Vertical"=701}, {"Horizontal"=604, "Vertical"=706}, {"Horizontal"=602, "Vertical"=710}, {"Horizontal"=597, "Vertical"=718}, {"Horizontal"=596, "Vertical"=718}, {"Horizontal"=597, "Vertical"=718}, {"Horizontal"=596, "Vertical"=717}, {"Horizontal"=596, "Vertical"=717}, {"Horizontal"=597, "Vertical"=715}, {"Horizontal"=598, "Vertical"=709}, {"Horizontal"=598, "Vertical"=709}, {"Horizontal"=597, "Vertical"=709}, {"Horizontal"=573, "Vertical"=709}, {"Horizontal"=585, "Vertical"=684}, {"Horizontal"=591, "Vertical"=655}, {"Horizontal"=597, "Vertical"=623}, {"Horizontal"=599, "Vertical"=596}, {"Horizontal"=588, "Vertical"=609}, {"Horizontal"=577, "Vertical"=631}, {"Horizontal"=566, "Vertical"=639}, {"Horizontal"=539, "Vertical"=591}, {"Horizontal"=545, "Vertical"=484}, {"Horizontal"=563, "Vertical"=510}, {"Horizontal"=582, "Vertical"=478}, {"Horizontal"=595, "Vertical"=486}, {"Horizontal"=606, "Vertical"=492}, {"Horizontal"=641, "Vertical"=500}, {"Horizontal"=652, "Vertical"=495}, {"Horizontal"=660, "Vertical"=496}, {"Horizontal"=684, "Vertical"=488}, {"Horizontal"=695, "Vertical"=478}, {"Horizontal"=701, "Vertical"=471}, {"Horizontal"=695, "Vertical"=427}, {"Horizontal"=683, "Vertical"=432}, {"Horizontal"=660, "Vertical"=437}, {"Horizontal"=651, "Vertical"=441}, {"Horizontal"=635, "Vertical"=438}, {"Horizontal"=615, "Vertical"=436}, {"Horizontal"=605, "Vertical"=434}, {"Horizontal"=594, "Vertical"=429}, {"Horizontal"=587, "Vertical"=422}, {"Horizontal"=591, "Vertical"=415}, {"Horizontal"=603, "Vertical"=422}, {"Horizontal"=619, "Vertical"=424}, {"Horizontal"=629, "Vertical"=424}, {"Horizontal"=645, "Vertical"=423}, {"Horizontal"=653, "Vertical"=422}, {"Horizontal"=661, "Vertical"=422}, {"Horizontal"=679, "Vertical"=421}, {"Horizontal"=686, "Vertical"=419}, {"Horizontal"=687, "Vertical"=418}, {"Horizontal"=705, "Vertical"=409}, {"Horizontal"=696, "Vertical"=390}, {"Horizontal"=687, "Vertical"=382}, {"Horizontal"=676, "Vertical"=378}, {"Horizontal"=664, "Vertical"=386}, {"Horizontal"=648, "Vertical"=397}, {"Horizontal"=642, "Vertical"=397}, {"Horizontal"=626, "Vertical"=394}, {"Horizontal"=616, "Vertical"=389}, {"Horizontal"=605, "Vertical"=383}, {"Horizontal"=606, "Vertical"=375}, {"Horizontal"=616, "Vertical"=361}, {"Horizontal"=624, "Vertical"=344}, {"Horizontal"=631, "Vertical"=329}, {"Horizontal"=641, "Vertical"=322}, {"Horizontal"=648, "Vertical"=330}, {"Horizontal"=657, "Vertical"=349}, {"Horizontal"=669, "Vertical"=360}, {"Horizontal"=681, "Vertical"=369}] ("XY Graph")
  n1 = while {
    shift-right: [w7] -> _
    shift-left: cluster{"X":dbl, "Y":dbl}[] [] -> [w8]
    stop <- w6 stop-if-true
    n2 = event shown="[2] \"stop\": Value Change" {
      selector: _ -> [_ _ _]
      dyn-events: _ -> [_ _ _]
      timeout: _ -> [_ _ _]
      tunnel: [w10 w18 w20] -> w7
      tunnel: w8 -> [w11 w17 w20]
      tunnel: [_ _ "stop"] -> w6
      event "XY Graph": Mouse Down? {
        n3 = event-data() -> ("CtlRef"=w14:refnum<vi>, "Coords"=w12:T2)  [unwired: 1 in, 3 out]
        n4 = invoke class="XYGraph (strict)" method="Map Coords To XY"(reference=w14, "Coords"=w12) -> (reference out=w13:refnum<vi>, "XY"=w9:cluster{"X":dbl, "Y":dbl})  [unwired: 5 in, 5 out]
        n5 = property class="XYGraph (strict)"(reference=w13, "Cursor.Cursor Position"=w9) -> ()  [unwired: 1 in, 2 out]
        n6 = Build Array (concatenate)(w11, w9) -> (w10:cluster{"X":dbl, "Y":dbl}[])
        n7 = event-data() -> ()  [unwired: 5 in, 1 out]
      }
      event "XY Graph": Cursor Move {
        n8 = event-data() -> ("CursLoc"=w16:cluster{"X":dbl, "Y":dbl})  [unwired: 1 in, 4 out]
        n9 = Build Array (concatenate)(w17, w16) -> (w18:cluster{"X":dbl, "Y":dbl}[])
        n10 = Wait (ms)(milliseconds to wait=u32 25) -> ()  [unwired: 1 out]
      }
      event "stop": Value Change {
        n11 = event-data() -> ()  [unwired: 1 in, 6 out]
      }
    }
    "XY Graph" <- w7
  }
  n12 = property on="XY Graph" class="XYGraph (strict)"() -> ("Plot Area Size"=w3:T1)  [unwired: 2 in, 2 out]
  "Plot Area:Size" <- w3
  n13 = Unbundle By Name(w3) -> ("Width"=w1:u32, "Height"=w2:u32)
  n14 = property on="XY Graph" class="XYGraph (strict)"("XScale.Maximum"=w1, "XScale.Minimum"=w4) -> ()  [unwired: 2 in, 2 out]
  n15 = property on="XY Graph" class="XYGraph (strict)"("YScale.Maximum"=w2, "YScale.Minimum"=w4) -> ()  [unwired: 2 in, 2 out]
